vi "DL-SMART-MS-Modify-06-18-7.0.vi"() -> ()   [LabVIEW 2013]
uses:
  <vilib>/Utility/file.llb/Read From Spreadsheet File (DBL).vi
  <userlib>/caLab/Private/CaLabEvent_PV-1D.vi
  <userlib>/caLab/Private/Put_DBL-1D_PV.vi
  <userlib>/caLab/Private/Put_I32_PV.vi
  cal_p.vi
  <userlib>/caLab/Private/Get_PV.vi
  <vilib>/Utility/file.llb/Write To Spreadsheet File (DBL).vi
  <vilib>/vision/driver/NI_Vision_Acquisition_Software.lvlib
  <resource>/objmgr/imaqdx.rc
  <vilib>/Analysis/NI_AALPro.lvlib
panel:
  out "LaserEnergy uJ 2":dbl
  out "idn status":string
  out "MS":cluster{dbl[], "filtered data":dbl[]}(graph)
  out "std sample":T1(array[cluster])
  out "Image":T2(plugin-control)
  out "selected id":i32
  out "selected row":i32
  out "currentNO":string
  out "commet":string
  out "sampleID":string
  in  "Shots/Point":i32=100
  in  "chamber in":bool caption="TakeMS"
  in  "chamber out":bool caption="TakeMS"
  in  "Laser parameter":T4
  in  "ADC parameter":T5
  in  "ShutDownSystem":bool
  in  "ADC reference":refnum<vi>
  in  "SetLaserTransmission":dbl(slide) min=0.0 max=50.0 scale=0.0..20.0
  in  "LaserHV":u8=50 min=1 max=100
  in  "频率/Hz":u8=30
  out "Pul.HV-Real":dbl
  out "Identify Spcetrum":cluster{"ID1:X":dbl[], "ID1:Y":dbl[]}[](graph)
  in  "测试记录":i32(listbox)=6
  in  "Identification Results (单靶鉴定结果)":i32(listbox)=2
  in  "HVEnable":bool
  out "GateClose":bool
  out "LaserOK":bool
  out "HV-OK":bool
  out "Vacuum-OK":bool
  in  "Tab Control":T6(tab)
  in  "helix-Zeta-Step":dbl=100.0
  in  "helix-b":dbl=0.2
  in  "AcquireMS-Methods":u8(ring) items=["SinglePoint", "Multipoints", "MultiTar"]
  in  "Thresh":dbl=-0.005 format="%#_13g"
  in  "right rank":i32=2
  in  "left rank":i32=2
  in  "deBaseline":bool
  in  "MCPHV-Set":dbl=1400.0 min=0.0 max=1600.0
  in  "LensHV-Set":dbl=8000.0 min=0.0 max=10000.0
  in  "Tar.HV-Set":dbl=18010.0 min=0.0 max=20000.0
  in  "Pul.HV-Set":dbl=1400.0 min=0.0 max=2000.0
  in  "PulseDelay":dbl
  in  "ADCFreq":dbl
  in  "CH1_Coupling":u64(ring)=2 items=["Volt DC"=1, "Volt AC"=2, "Ampere DC"=4, "Ampere AC"=8, "Ohm"=16]
  in  "Channel 1_Range":dbl(ring)=4.0 items=["80 V"=80.0, "40 V"=40.0, "20 V"=20.0, "8 V"=8.0, "4 V"=4.0, "2 V"=2.0, "800 mV"=0.8, "400 mV"=0.4, "200 mV"=0.2]
  in  "Anal. Setting File":string="High Mass"
  in  "SettingFileSave":bool caption="TakeMS"
  in  "SettingFileAppl":bool caption="TakeMS"
  in  "SettingDel":bool caption="TakeMS"
  in  "RunADC":bool caption="TakeMS"
  out "ADCstatus":bool
  in  "Vac_Prot.":bool
  in  "Turbo_Fore":bool
  in  "Main_Samp":bool
  in  "Samp_Atmos":bool
  in  "Fore_Samp":bool
  in  "StartPump":bool
  in  "SopPump":bool
  out "TurboSpeed":dbl(knob) scale=0.0..100.0
  out "PumpKW":dbl
  out "PumpAmps":dbl
  out "PumpTemp":u16
  out "PumpVolts":dbl
  in  "laser OFF":bool
  in  "laser ON":bool
  out "cluster":T7
  in  "laser Deactive":bool
  out "A1-position-Y":dbl=45.0 caption="Y" min=0.0 max=55.0
  out "A1-position-X":dbl=53.4 caption="X" min=0.0 max=55.0
  in  "GO":bool
  in  "Y":dbl min=0.0 max=55.0
  in  "X":dbl min=0.0 max=55.0
  in  "A1-Position":bool caption="X-"
  in  "Plat_To_Zero":bool caption="TakeMS"
  in  "Plat_Cal":bool caption="TakeMS"
  out "Y当前":dbl
  out "X当前":dbl
  out "移动":bool
  out "Y满":bool
  out "Y标":bool
  out "X满":bool
  out "Y0":bool
  out "X0":bool
  out "靶位In/Out":bool
  out "仓门":bool
  out "Y过热":bool
  out "X过热":bool
  out "通讯":bool
  in  "Operation Record":i32(listbox)
  in  "OptionRecordLoad 2":bool caption="TakeMS"
  in  "OptionRecordClear":bool caption="TakeMS"
  out "c:":dbl
  out "b:":dbl
  out "a:":dbl
  in  "cancel cal":bool
  in  "cal save":bool
  in  "peak cal":bool
  in  "peak detect":bool
  in  "标准样品":u16(ring) items=["肺炎克雷伯菌", "铜绿假单胞菌"]
  in  "定标参数":i32(listbox)
  out "Tar.HV-Real":dbl
  out "LensHV-Real":dbl
  out "MCPHV-Real":dbl
  out "Lvaccum":dbl=0.83 format="%#_2e"
  out "Hvaccum":dbl=3.4e-05 format="%#_2e"
  in  "H12":bool
  in  "G12":bool
  in  "F12":bool
  in  "E12":bool
  in  "D12":bool
  in  "C12":bool
  in  "B12":bool
  in  "A12":bool
  in  "H11":bool
  in  "G11":bool
  in  "F11":bool
  in  "E11":bool
  in  "D11":bool
  in  "C11":bool
  in  "B11":bool
  in  "A11":bool
  in  "H10":bool
  in  "G10":bool
  in  "F10":bool
  in  "E10":bool
  in  "D10":bool
  in  "C10":bool
  in  "B10":bool
  in  "A10":bool
  in  "H9":bool
  in  "G9":bool
  in  "F9":bool
  in  "E9":bool
  in  "D9":bool
  in  "C9":bool
  in  "B9":bool
  in  "A9":bool
  in  "H8":bool
  in  "G8":bool
  in  "F8":bool
  in  "E8":bool
  in  "D8":bool
  in  "C8":bool
  in  "B8":bool
  in  "A8":bool
  in  "H7":bool
  in  "G7":bool
  in  "F7":bool
  in  "E7":bool
  in  "D7":bool
  in  "C7":bool
  in  "B7":bool
  in  "A7":bool
  in  "H6":bool
  in  "G6":bool
  in  "F6":bool
  in  "E6":bool
  in  "D6":bool
  in  "C6":bool
  in  "B6":bool
  in  "A6":bool
  in  "H5":bool
  in  "G5":bool
  in  "F5":bool
  in  "E5":bool
  in  "D5":bool
  in  "C5":bool
  in  "B5":bool
  in  "A5":bool
  in  "H4":bool
  in  "G4":bool
  in  "F4":bool
  in  "E4":bool
  in  "D4":bool
  in  "C4":bool
  in  "B4":bool
  in  "A4":bool
  in  "H3":bool
  in  "G3":bool
  in  "F3":bool
  in  "E3":bool
  in  "D3":bool
  in  "C3":bool
  in  "B3":bool
  in  "A3":bool
  in  "H2":bool
  in  "G2":bool
  in  "F2":bool
  in  "E2":bool
  in  "D2":bool
  in  "C2":bool
  in  "B2":bool
  in  "A2":bool
  in  "H1":bool
  in  "G1":bool
  in  "F1":bool
  in  "E1":bool
  in  "D1":bool
  in  "C1":bool
  in  "B1":bool
  in  "A1":bool
  in  "Clear":bool caption="TakeMS"
  in  "Add":bool caption="TakeMS"
  in  "TakeMS-Stop":bool caption="TakeMS"
  in  "TakeMS-Run":bool caption="TakeMS"
  # "Laser (激光)"
  # "光栅"
  # "uJ"
  # "Acq.(采谱)"
  # "Vacuum(真空)"
  # "1"
  # "2"
  # "3"
  # "4"
  # "5"
  # "6"
  # "7"
  # "8"
  # "9"
  # "10"
  # "11"
  # "12"
  # "A"
  # "Pa"
  # "High"
  # "B"
  # "Low"
  # "Pa"
  # "C"
  # "H.V.(高压)"
  # "D"
  # "MCP"
  # "V"
  # "E"
  # "Tar."
  # "V"
  # "F"
  # "Pul."
  # "V"
  # "G"
  # "Lens"
  # "V"
  # "H"
  # "Vauum (真空)"
  # "H.V. (高压)"
  # "Laser (激光)"
  # "Gate (仓门)"
  # "mm"
  # "Radian"
  # "H.V. (高压参数)"
  # "ADC(采集卡设置)"
  # "ADCFreq(采样)"
  # "MCP (探测器)"
  # "V"
  # "Hz"
  # "Tar. (靶)"
  # "V"
  # "Setting File(设置文件)"
  # "Coupling"
  # "Pulse (脉冲)"
  # "V"
  # "IntRange"
  # "V"
  # "Lens (透镜)"
  # "Delay (延时)"
  # "ns"
  # "Sole. Valves"
  # "Turbo Pump"
  # "自锁保护"
  # "机械/分子"
  # "主仓/样仓"
  # "样仓/大气"
  # "机械/样仓"
  # "激光器状态"
  # "mm"
  # "mm"
  # "mm"
  # "mm"
  # "mm"
  # "mm"
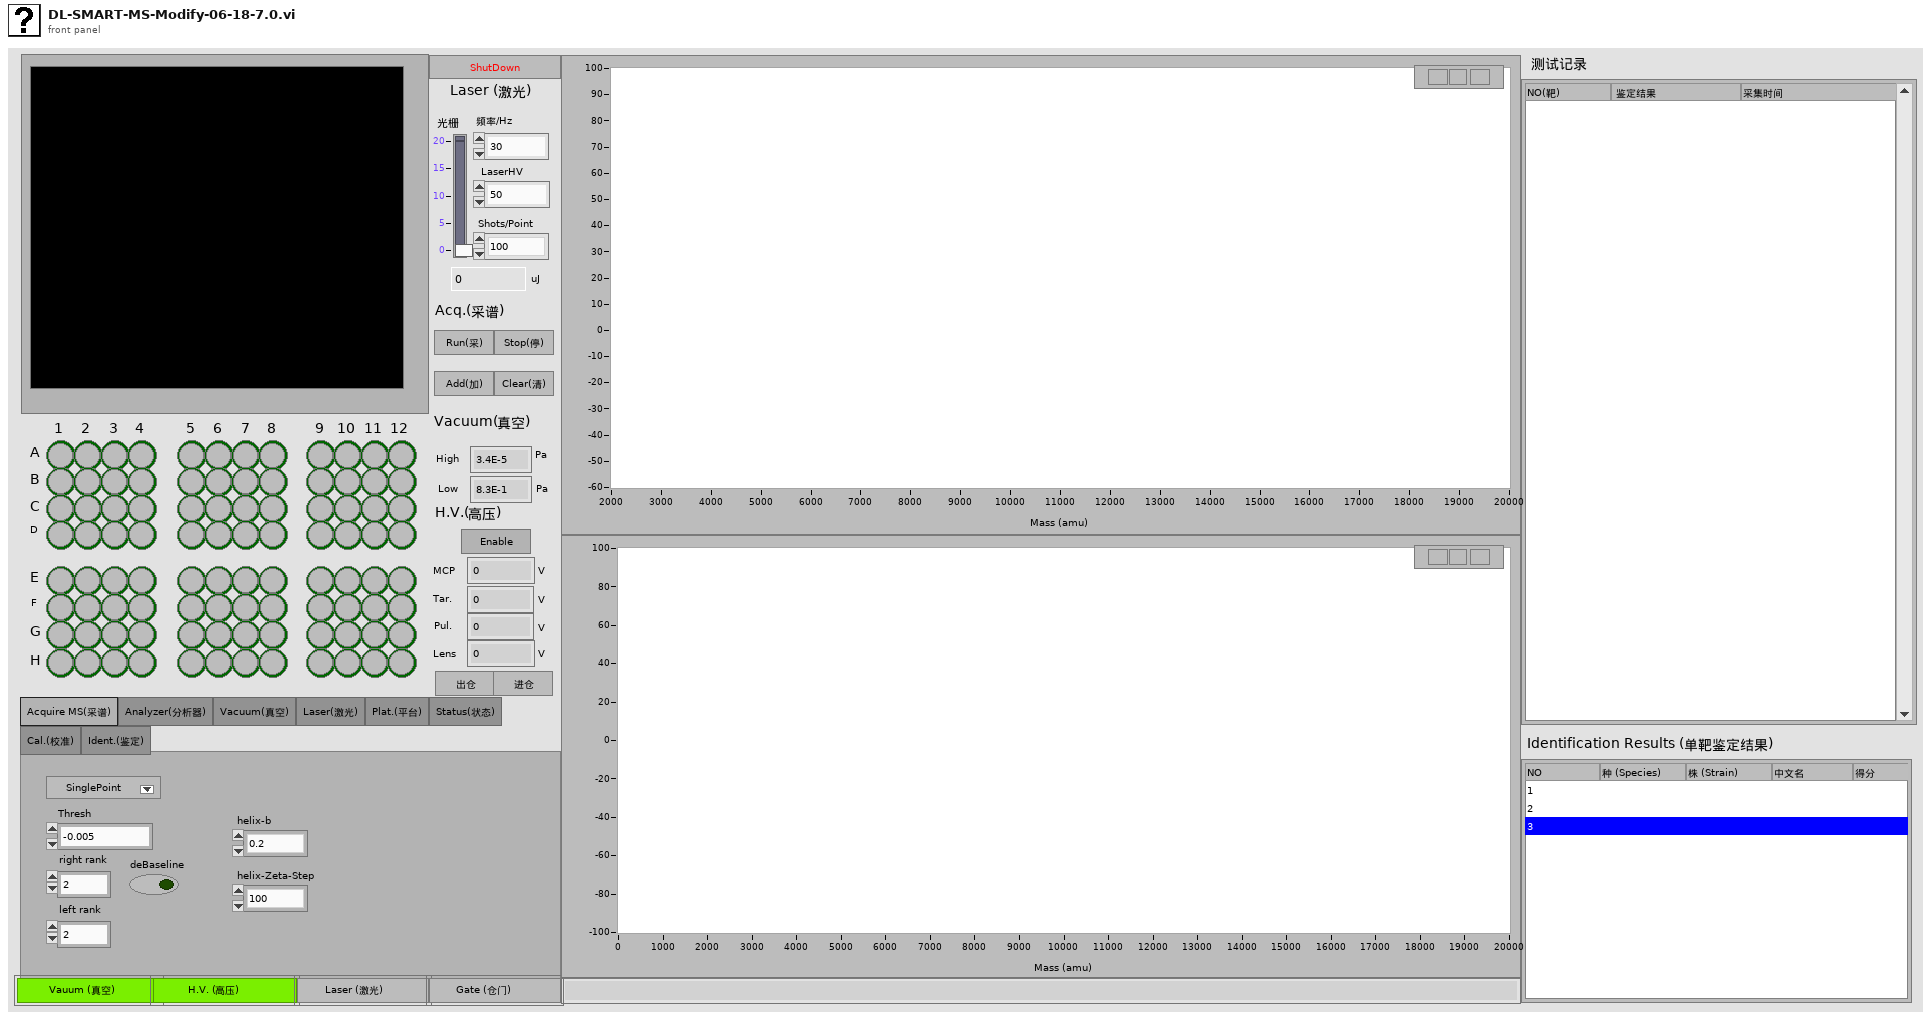
[diagram p1: front panel]
types:
  T1 = cluster{"name":string, "mz":dbl[], "time":dbl[]}[]
  T2 = typedef "IMAQ Image.ctl" = refnum<image>
  T3 = typedef "Semaphore RefNum" = refnum<k1>
  T4 = cluster{"VISA resource name":refnum<visa-resource-name>, "standby":bool, "semaphore in":T3, "SetLaserEnergy":dbl}
  T5 = cluster{"TpDeviceHandle_t":u32, "Record Length/Samples":u64, "ShotsPerPoint":u16}
  T6 = enum32{"Acquire MS(采谱)", "Analyzer(分析器)", "Vacuum(真空)", "Laser(激光)", "Plat.(平台)", "Status(状态)", "Cal.(校准)", "Ident.(鉴定)"}
  T7 = cluster{"链接":bool, "待机":bool, "发射":bool, "[3]":bool, "内存":bool, "测能":bool, "温警":bool, "静态":bool, "操作":bool}
  T8 = cluster{"tag1":string, "tag2":string, "x":dbl[], "y":dbl[], "ID1:X":dbl[], "ID1:Y":dbl[], "ID1:REF:X":dbl[], "ID1:REF:Y":dbl[], "ID2:X":dbl[], "ID2:Y":dbl[], "ID2:REF:X":dbl[], "ID2:REF:Y":dbl[], "ID3:X":dbl[], "ID3:Y":dbl[], "ID3:REF:X":dbl[], "ID3:REF:Y":dbl[], "ID1:TAG1":string, "ID1:TAG2":string, "ID2:TAG1":string, "ID2:TAG2":string, "ID3:TAG1":string, "ID3:TAG2":string, "ID1:NAME":string, "ID2:NAME":string, "ID3:NAME":string, "ID1:SCORE":string, "ID2:SCORE":string, "ID3:SCORE":string, "NO":string}[]
  T9 = cluster{"laser semaphore":T3, "pump semaphore":T3}
  T10 = enum8{"Enabled", "Disabled", "Disabled and Grayed Out"}
  T11 = cluster{"tag1":string, "tag2":string, "x":dbl[], "y":dbl[], "ID1:X":dbl[], "ID1:Y":dbl[], "ID1:REF:X":dbl[], "ID1:REF:Y":dbl[], "ID2:X":dbl[], "ID2:Y":dbl[], "ID2:REF:X":dbl[], "ID2:REF:Y":dbl[], "ID3:X":dbl[], "ID3:Y":dbl[], "ID3:REF:X":dbl[], "ID3:REF:Y":dbl[], "ID1:TAG1":string, "ID1:TAG2":string, "ID2:TAG1":string, "ID2:TAG2":string, "ID3:TAG1":string, "ID3:TAG2":string, "ID1:NAME":string, "ID2:NAME":string, "ID3:NAME":string, "ID1:SCORE":string, "ID2:SCORE":string, "ID3:SCORE":string, "NO":string}
  T12 = cluster{"monitor":refnum<user-event>, "motor status":refnum<user-event>, "motor":refnum<user-event>, "notifier out":refnum<notifier>, "queue out":refnum<queue>, "AI":T3, "DI":T3, "CX":T3, "CY":T3}
  T13 = cluster{"AI Task":refnum<k21>, "AO Task":refnum<k21>, "DO Task":refnum<k21>, "DI Task":refnum<k21>, "PWM x":refnum<k21>, "PWM y":refnum<k21>, "counter x":refnum<k21>, "counter y":refnum<k21>}
  T14 = cluster{"tasks":cluster{"AI Task":refnum<k21>, "AO Task":refnum<k21>, "DO Task":refnum<k21>, "DI Task":refnum<k21>, "PWM x":refnum<k21>, "PWM y":refnum<k21>, "counter x":refnum<k21>, "counter y":refnum<k21>}, "interface":cluster{"monitor":refnum<user-event>, "motor status":refnum<user-event>, "motor":refnum<user-event>, "notifier out":refnum<notifier>, "queue out":refnum<queue>, "AI":T3, "DI":T3, "CX":T3, "CY":T3}, "error out":errorcluster}
  T15 = cluster{"ConfiguredPumpCom":refnum<visa-resource-name>, "ConfiguredLaserCom":refnum<visa-resource-name>}
  T16 = typedef "LVPoint32TypeDef.ctl" = cluster{"Horizontal":i32, "Vertical":i32}
  T17 = typedef "LVRowAndColumnTypeDef.ctl" = cluster{"Row":i32, "Column":i32}
  T18 = cluster{"Type":u32, "Version":u32, "Flags":u32, "SerialNumberHigh":u32, "SerialNumberLow":u32, "BusType":u32, "InterfaceName":string, "VendorName":string, "ModelName":string, "CameraFileName":string, "CameraAttributeURL":string}[]
  T19 = cluster{"Type":u32, "Version":u32, "Flags":u32, "SerialNumberHigh":u32, "SerialNumberLow":u32, "BusType":u32, "InterfaceName":string, "VendorName":string, "ModelName":string, "CameraFileName":string, "CameraAttributeURL":string}
  T20 = typedef "IMAQdx.ctl" = refnum<k21>
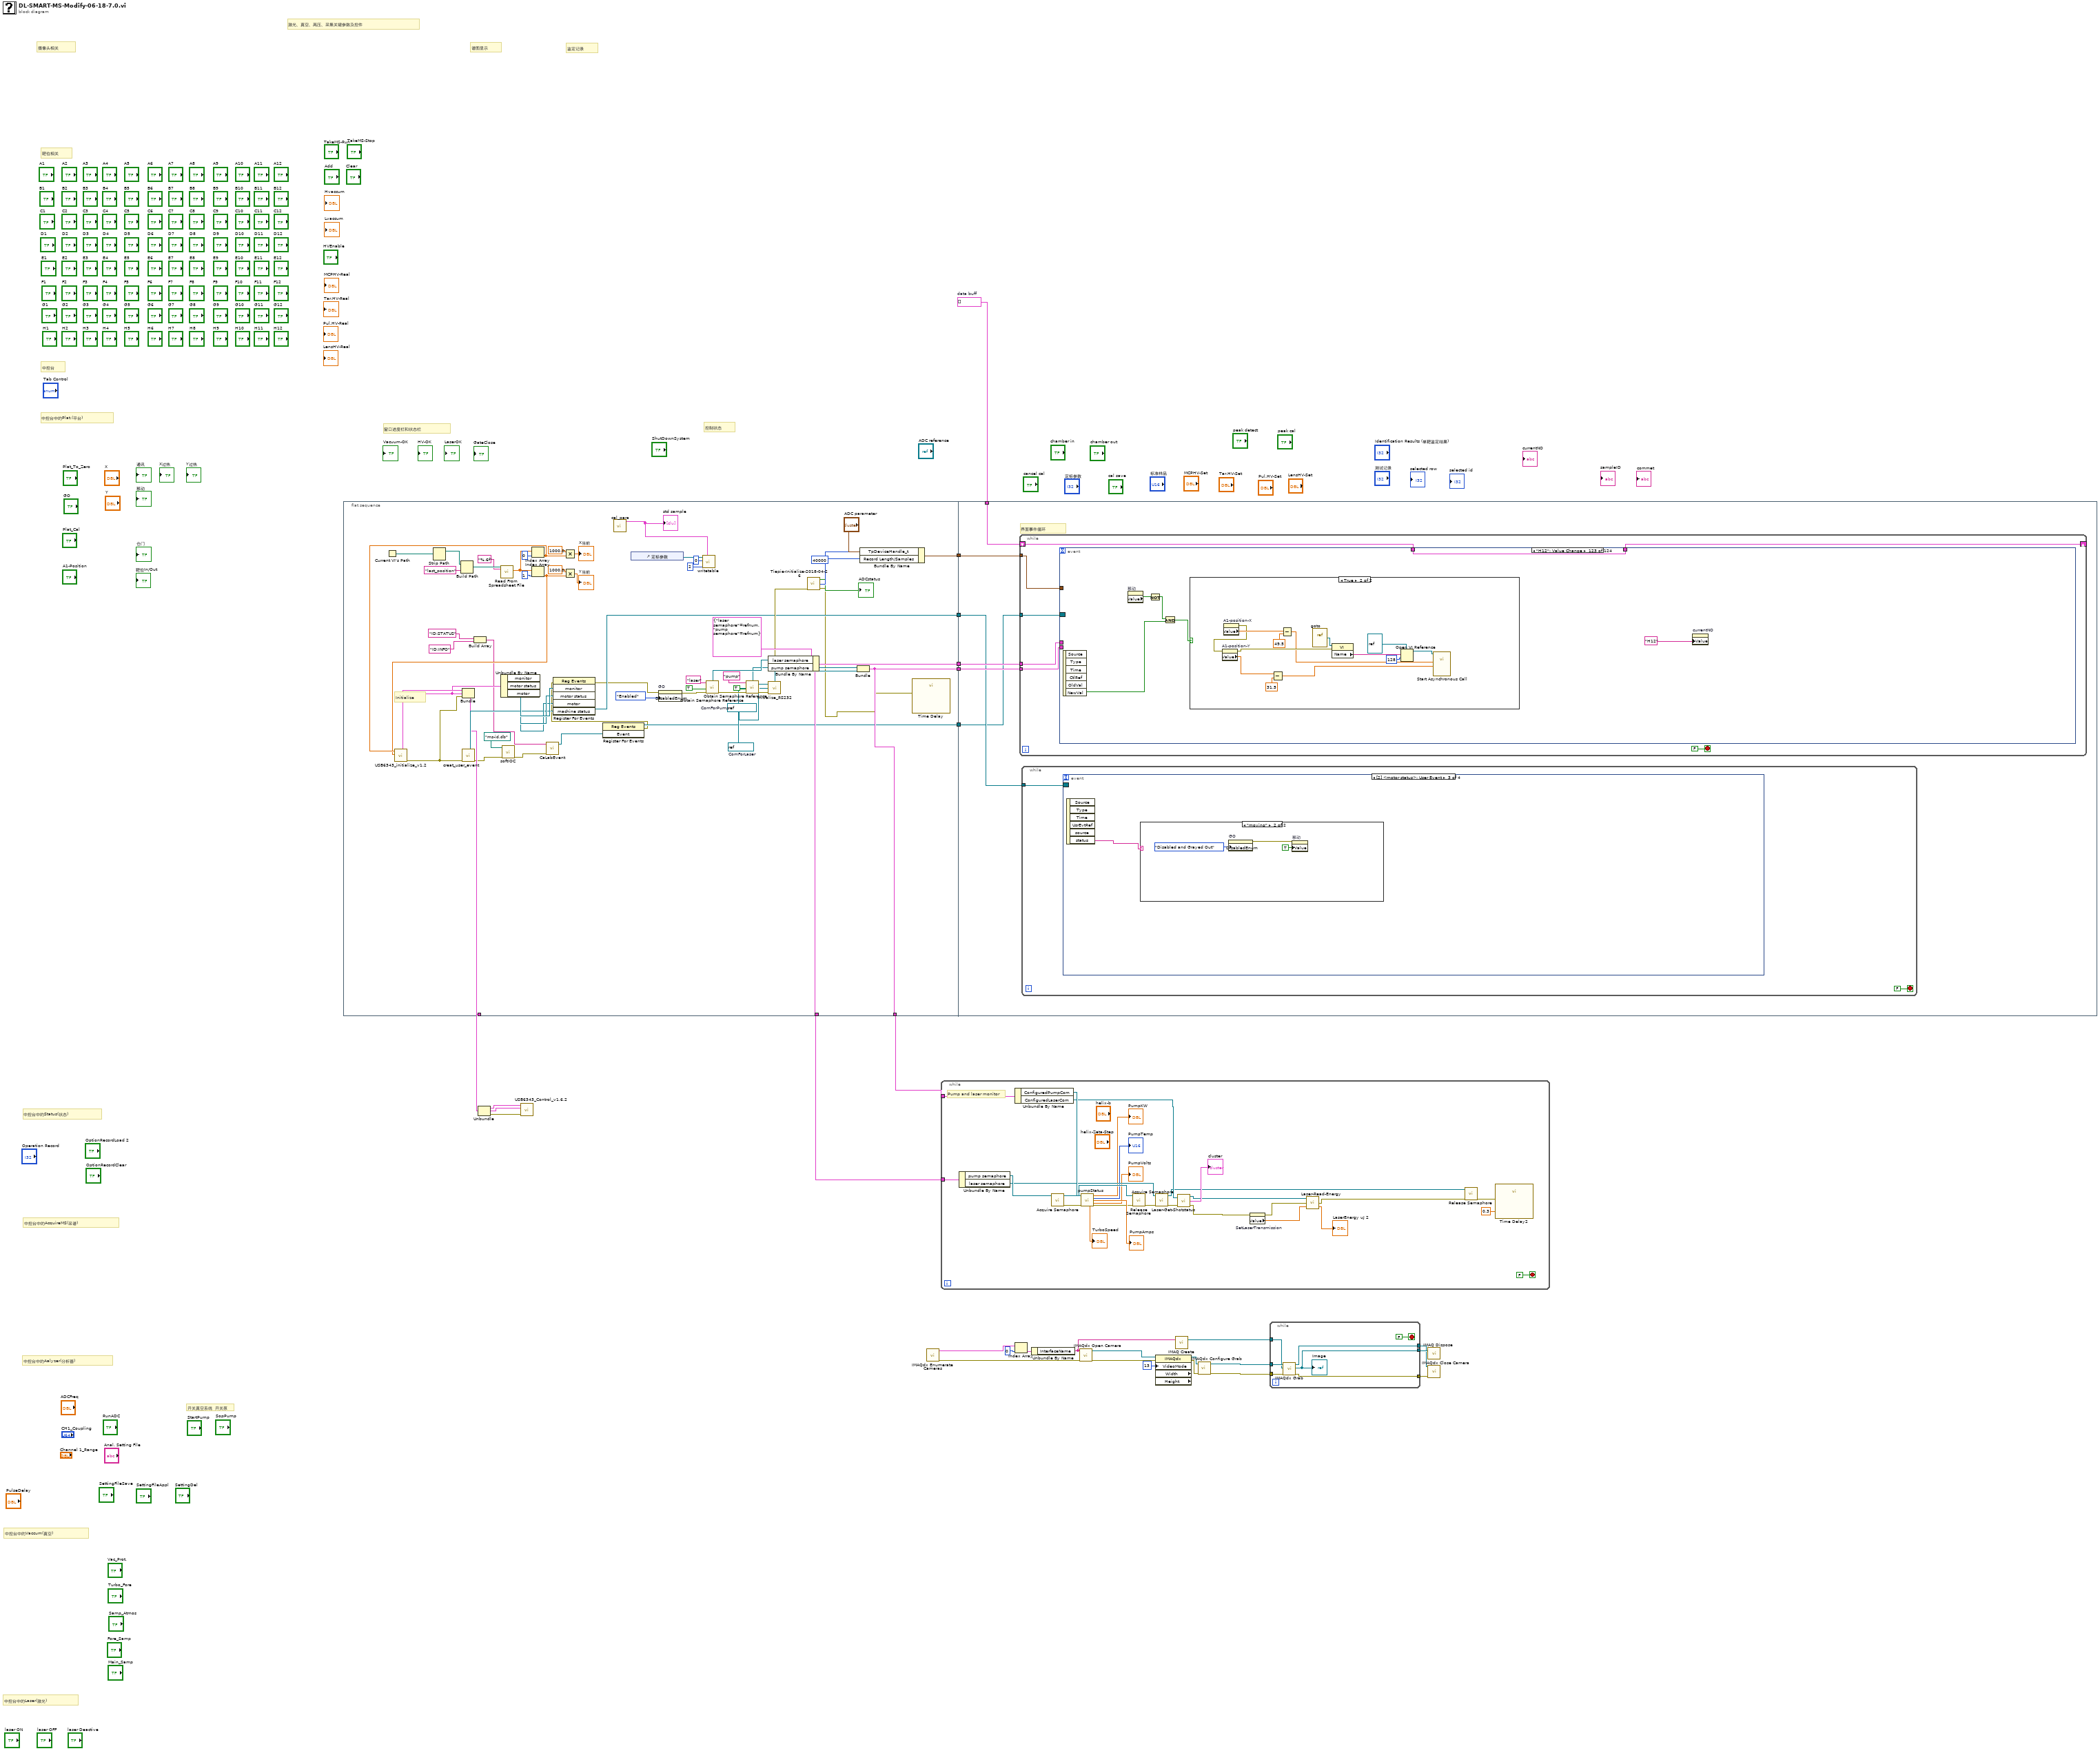
[diagram p0: block diagram]
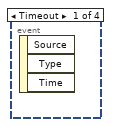
[diagram p2: hidden frame]
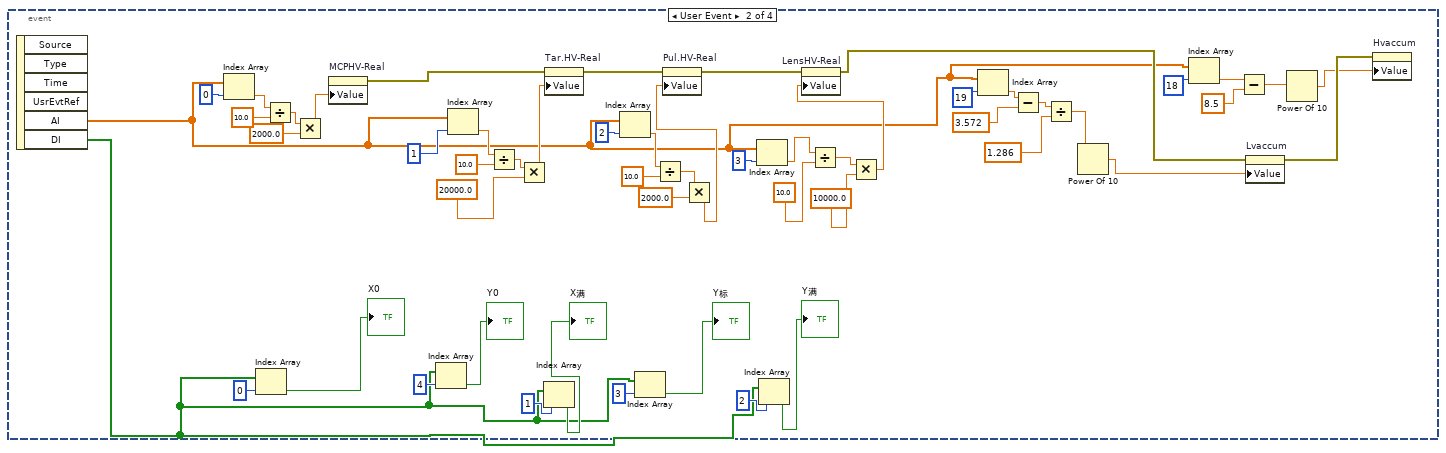
[diagram p3: hidden frame]
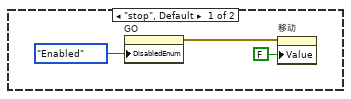
[diagram p4: hidden frame]
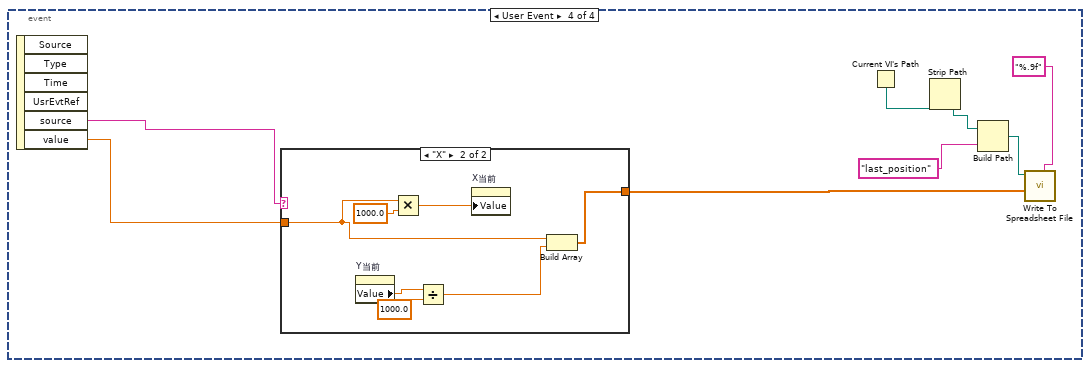
[diagram p5: hidden frame]
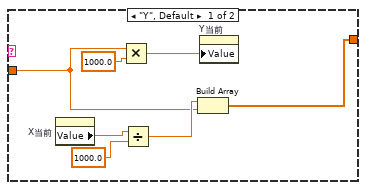
[diagram p6: hidden frame]
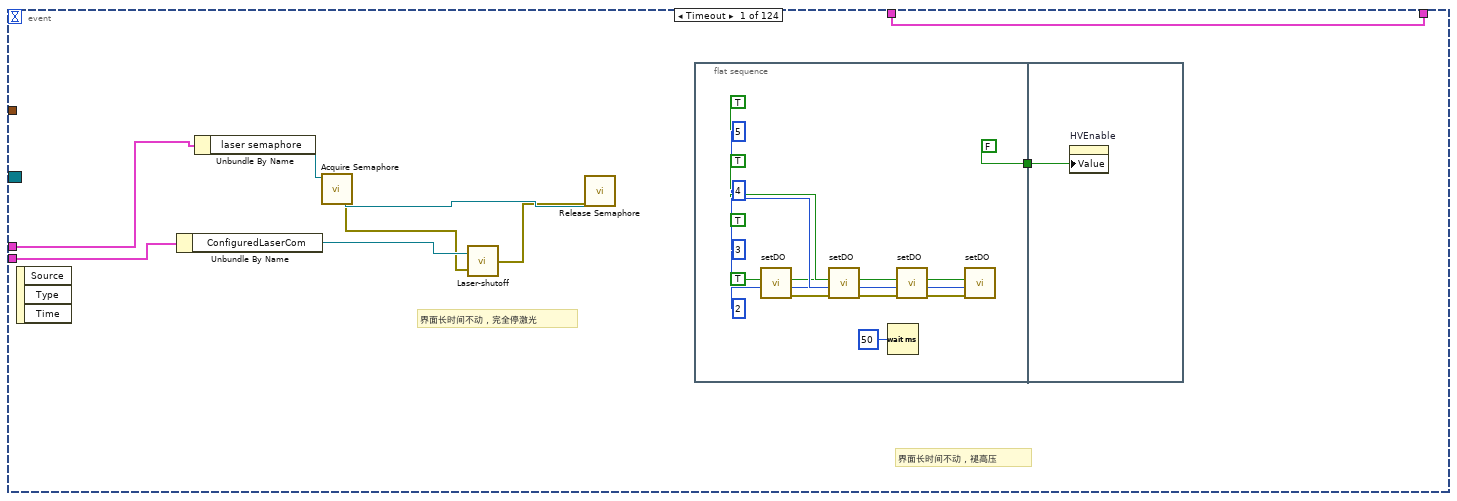
[diagram p7: hidden frame]
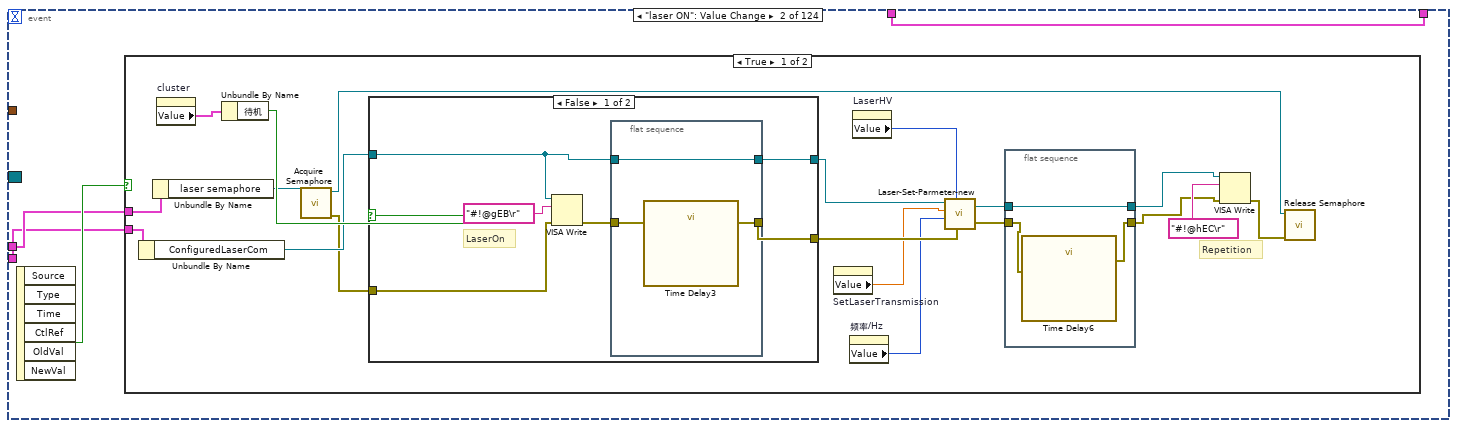
[diagram p8: hidden frame]
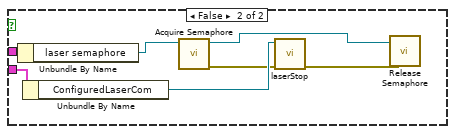
[diagram p10: hidden frame]
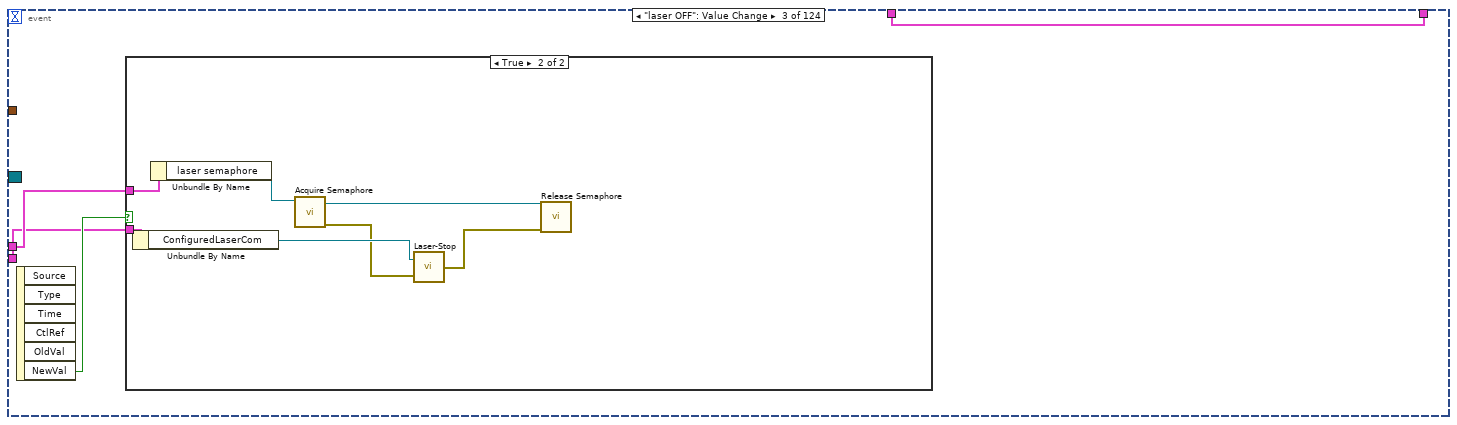
[diagram p11: hidden frame]
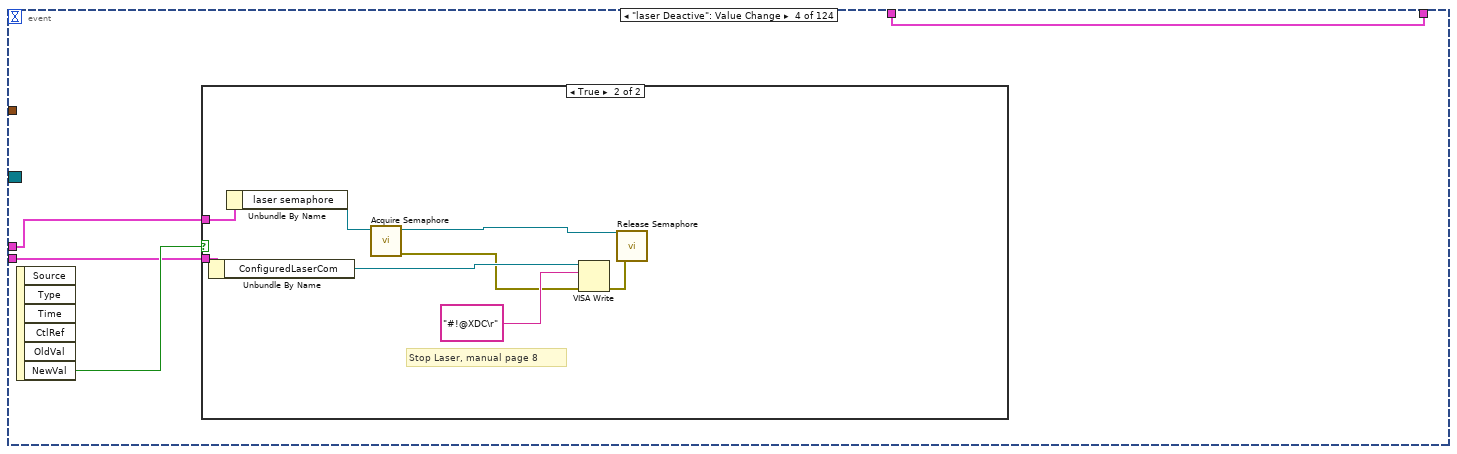
[diagram p13: hidden frame]
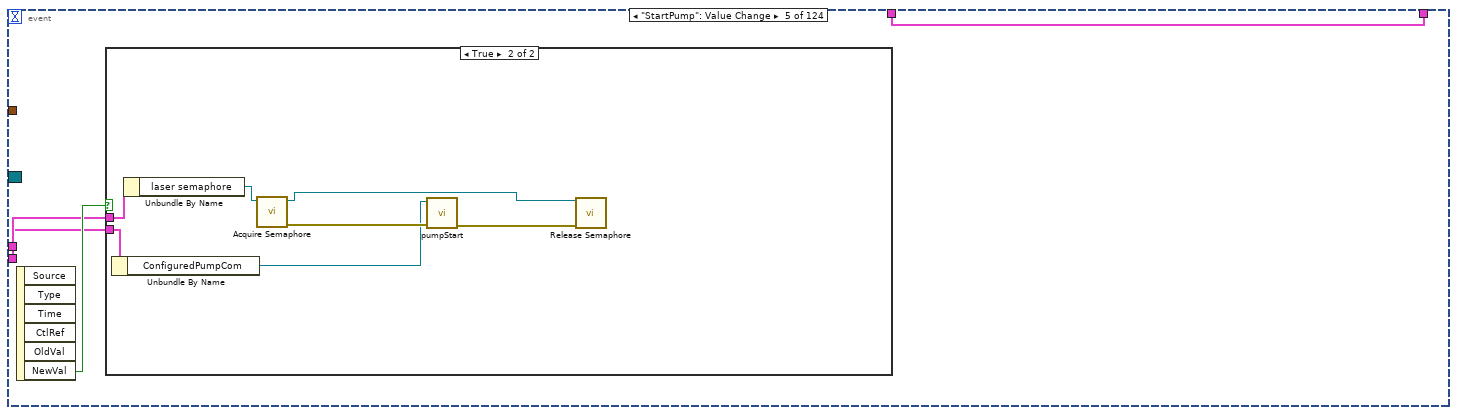
[diagram p15: hidden frame]
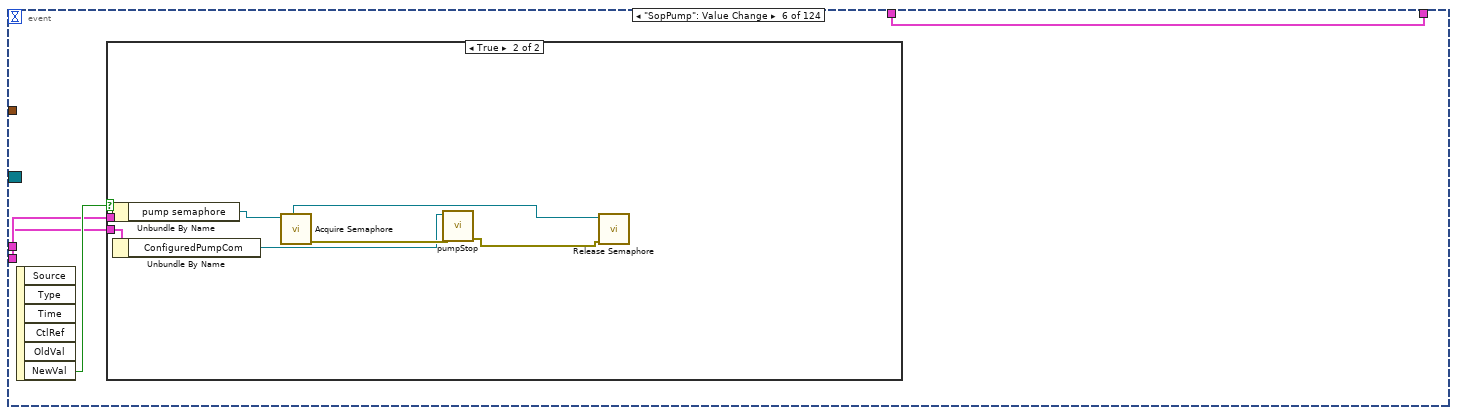
[diagram p17: hidden frame]
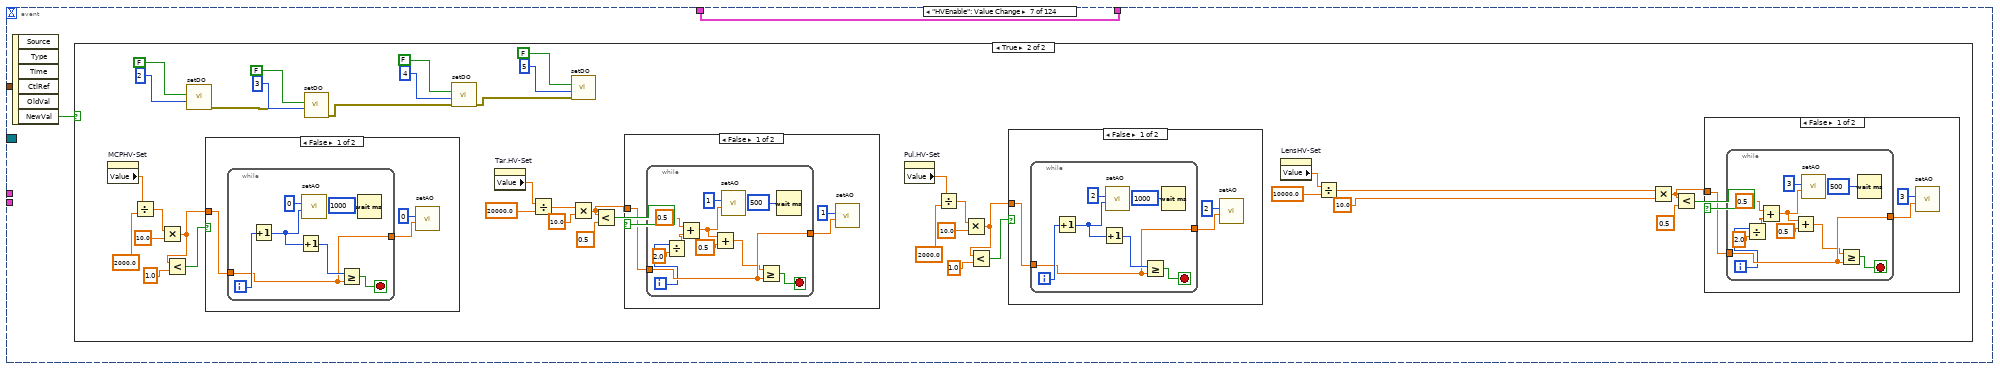
[diagram p19: hidden frame]
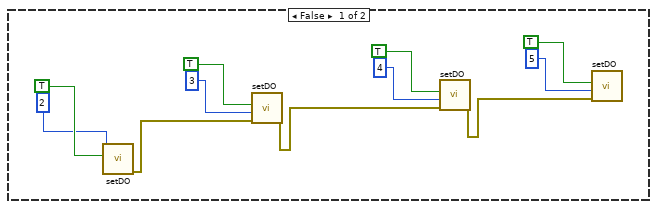
[diagram p20: hidden frame]
diagram:
  w21 = T8 []  # data buff
  # "Pump and laser monitor"
  # "开关真空系统  开关泵"
  # "控制状态"
  # "鉴定记录"
  # "谱图显示"
  # "激光、真空、高压、采集关键参数及控件"
  # "窗口进度栏和状态栏"
  # "中控台中的Laser(激光)"
  # "中控台中的Vaccum(真空)"
  # "中控台中的Aalyzer(分析器)"
  # "中控台中的AcquireMS(采谱)"
  # "中控台中的Status(状态)"
  # "中控台中的Plat.(平台)"
  # "中控台"
  # "靶位相关"
  # "摄像头相关"
  n1 = flat-sequence {
    tunnel: [w43] -> w28
    tunnel: [w68] -> w27
    tunnel: [w68] -> w25
    tunnel: [w67] -> w26
    tunnel: [w67] -> w24
    tunnel: [w71] -> w23
    tunnel: [w60] -> w22
    tunnel: [w30] -> w1
    tunnel: w28 -> [w91]
    tunnel: w27 -> [w95]
    tunnel: w26 -> [w94]
    tunnel: w22 -> [w93]
    tunnel: w21 -> [w92]
    tunnel: w1 -> [w90]
    frame #0 {
      w65 = refnum<visa-resource-name> "COM9"  # ComForLaser
      w66 = refnum<visa-resource-name> "COM10"  # ComForPump
      # "Initialize"
      n2 = Current VI's Path() -> (path=w58:path)
      n3 = Strip Path(path=w58) -> (stripped path=w57:path)  [unwired: 1 out]
      n4 = Build Path(base path=w57, name or relative path="last_position") -> (appended path=w55:path)
      n5 = Build Array("ID:STATUS", "ID:INFO") -> (w32:string[])
      n6 = call-poly <vilib>:"Read From Spreadsheet File.vi"("format (%.3f)"="%.6f", "file path (dialog if empty)"=w55) -> ("first row"=w53:dbl[])  [unwired: 5 in, 4 out]
      n7 = Index Array(array=w53, index=0) -> (element=w50:dbl)
      n8 = Index Array(array=w53, index=1) -> (element=w47:dbl)
      n9 = call "USB6343_initialize_v1.2.vi"("Y initial position"=w47, "X initial position"=w50) -> ("error out"=w72:errorcluster, "interface"=w73:T12, "tasks"=w74:T13)  [unwired: 7 in]
      n10 = Bundle("tasks"=w74, "interface"=w73, "error out"=w72) -> (w71:T14)  [unwired: 1 in]
      n11 = call "creat_user_event.vi"("error in (no error)"=w72) -> ("error out"=w40:errorcluster, "machine status"=w82:refnum<user-event>)  [unwired: 9 in]
      n12 = Unbundle By Name(w73) -> ("monitor"=w89:refnum<user-event>, "motor status"=w88:refnum<user-event>, "motor"=w87:refnum<user-event>)
      n13 = call "softIOC.vi"("error in (no error)"=w40, "路径"=path "ms-id.db") -> ("error out"=w41:errorcluster)  [unwired: 8 in, 1 out]
      n14 = call-poly <userlib>:"CaLabEvent.vi"("error in (no error)"=w41, "PV Names"=w32) -> ("Event"=w31:refnum<user-event>)  [unwired: 7 in, 2 out]
      n15 = Multiply(x=1000.0, y=w50) -> (x*y=→"X当前":dbl)
      n16 = Multiply(x=1000.0, y=w47) -> (x*y=→"Y当前":dbl)
      n17 = register-events(w31) -> (reference out=w30:refnum<event-registration>, error out=w29:errorcluster)  [unwired: 2 in]
      n18 = register-events(error in=w29, w89, w88, w87, w82) -> (reference out=w43:refnum<event-registration>, error out=w39:errorcluster)  [unwired: 1 in]
      n19 = call "cal_para.vi"() -> ("std sample"=w36:T1)  [unwired: 11 in]
      "std sample" <- w36
      n20 = control-ref of="定标参数"() -> (w38:refnum<vi>)
      n21 = property on="GO" class="Bool (strict)"(error in=w39, "DisabledEnum"=T10."Enabled" ("Disabled")) -> (error out=w83:errorcluster)  [unwired: 1 in, 1 out]
      n22 = call "writetable.vi"("std sample"=w36, "col"=2, "type"=0, "reference"=w38) -> ()  [unwired: 8 in]
      n23 = call <vilib>:"Obtain Semaphore Reference.vi"("error in (no error)"=w83, "create if not found (T)"=TRUE, "name (unnamed)"="laser") -> ("error out"=w78:errorcluster, "semaphore"=w75:T3)  [unwired: 2 in, 1 out]
      n24 = call <vilib>:"Obtain Semaphore Reference.vi"("error in (no error)"=w78, "create if not found (T)"=TRUE, "name (unnamed)"="pump") -> ("error out"=w77:errorcluster, "semaphore"=w69:T3)  [unwired: 2 in, 1 out]
      n25 = Bundle By Name(cluster=T9 {"laser semaphore"=refnum, "pump semaphore"=refnum}, "laser semaphore"=w75, "pump semaphore"=w69) -> (w68:T9)
      n26 = call "Initialize_RS232.vi"("error in (no error)"=w77, "ComForLaser"=w65, "ComForPump"=w66) -> ("error out"=w64:errorcluster, "ConfiguredLaserCom"=w80:refnum<visa-resource-name>, "ConfiguredPumpCom"=w81:refnum<visa-resource-name>)
      n27 = call "Tiepie-Initialize-2018-04-26.vi"("error in (no error)"=w64) -> ("error out"=w42:errorcluster, "TpDeviceHandle_t"=w62:u32, "Card-OK"=→"ADCstatus":bool)  [unwired: 3 in]
      n28 = Bundle("ConfiguredPumpCom"=w81, "ConfiguredLaserCom"=w80) -> (w67:T15)  [unwired: 1 in]
      n29 = Bundle By Name(cluster="ADC parameter", "TpDeviceHandle_t"=w62, "Record Length/Samples"=u64 40000) -> (w60:T5)
      n30 = call "Time Delay"("error in (no error)"=w42) -> ()  [unwired: 10 in, 1 out]
    }
    frame #1 {
      # "界面事件循环"
      n31 = while {
        tunnel: w90 -> [w186]
        tunnel: w94 -> [w185]
        tunnel: w95 -> [w184]
        tunnel: w93 -> [w182]
        shift-right: [w180] -> _
        shift-left: w92 -> [w181]
        stop <- FALSE stop-if-true
        n32 = event shown="[122] \"H12\": Value Change" {
          selector: w186 -> [_ _ _ _ _ _ _ _ _ _ _ _ _ _ _ _ _ _ _ _ _ _ _ _ _ _ _ _ _ _ _ _ _ _ _ _ _ _ _ _ _ _ _ _ _ _ _ _ _ _ _ _ _ _ _ _ _ _ _ _ _ _ _ _ _ _ _ _ _ _ _ _ _ _ _ _ _ _ _ _ _ _ _ _ _ _ _ _ _ _ _ _ _ _ _ _ _ _ _ _ _ _ _ _ _ _ _ _ _ _ _ _ _ _ _ _ _ _ _ _ _ _ _ _]
          dyn-events: _ -> [_ _ _ _ _ _ _ _ _ _ _ _ _ _ _ _ _ _ _ _ _ _ _ _ _ _ _ _ _ _ _ _ _ _ _ _ _ _ _ _ _ _ _ _ _ _ _ _ _ _ _ _ _ _ _ _ _ _ _ _ _ _ _ _ _ _ _ _ _ _ _ _ _ _ _ _ _ _ _ _ _ _ _ _ _ _ _ _ _ _ _ _ _ _ _ _ _ _ _ _ _ _ _ _ _ _ _ _ _ _ _ _ _ _ _ _ _ _ _ _ _ _ _ _]
          timeout: _ -> [_ _ _ _ _ _ _ _ _ _ _ _ _ _ _ _ _ _ _ _ _ _ _ _ _ _ _ _ _ _ _ _ _ _ _ _ _ _ _ _ _ _ _ _ _ _ _ _ _ _ _ _ _ _ _ _ _ _ _ _ _ _ _ _ _ _ _ _ _ _ _ _ _ _ _ _ _ _ _ _ _ _ _ _ _ _ _ _ _ _ _ _ _ _ _ _ _ _ _ _ _ _ _ _ _ _ _ _ _ _ _ _ _ _ _ _ _ _ _ _ _ _ _ _]
          tunnel: w185 -> [w189 w211 w254 w265 w277 w288 _ _ _ _ _ _ _ _ w483 w542 _ _ _ _ _ _ _ _ _ _ _ _ _ _ _ _ _ _ _ _ _ _ _ _ _ _ _ _ _ _ _ _ _ _ _ _ _ _ _ _ _ _ _ _ _ _ _ _ _ _ _ _ _ _ _ _ _ _ _ _ _ _ _ _ _ _ _ _ _ _ _ _ _ _ _ _ _ _ _ _ _ _ _ _ _ _ _ _ _ _ _ _ _ _ _ _ _ _ _ _ _ _ _ _ _ _ _ w2602]
          tunnel: w184 -> [w190 w212 w255 w264 w278 w289 _ _ _ _ _ _ _ _ w484 w543 _ _ _ _ _ _ _ _ _ _ _ _ _ _ _ _ _ _ _ _ _ _ _ _ _ _ _ _ _ _ _ _ _ _ _ _ _ _ _ _ _ _ _ _ _ _ _ _ _ _ _ _ _ _ _ _ _ _ _ _ _ _ _ _ _ _ _ _ _ _ _ _ _ _ _ _ _ _ _ _ _ _ _ _ _ _ _ _ _ _ _ _ _ _ _ _ _ _ _ _ _ _ _ _ _ _ _ _]
          tunnel: w182 -> [_ _ _ _ _ _ _ _ _ _ _ _ _ _ w485 _ _ _ _ _ _ _ _ _ _ _ _ _ _ _ _ _ _ _ _ _ _ _ _ _ _ _ _ _ _ _ _ _ _ _ _ _ _ _ _ _ _ _ _ _ _ _ _ _ _ _ _ _ _ _ _ _ _ _ _ _ _ _ _ _ _ _ _ _ _ _ _ _ _ _ _ _ _ _ _ _ _ _ _ _ _ _ _ _ _ _ _ _ _ _ _ _ _ _ _ _ _ _ _ _ _ _ _ _]
          tunnel: w181 -> [w187 w210 w253 w267 w276 w287 w298 w406 w421 w436 w443 w450 w457 w466 w482 w544 w546 w576 w611 w650 w652 w659 w694 w729 w731 w770 w775 w791 w809 w826 w843 w860 w877 w896 w921 w938 w955 w972 w989 w1006 w1025 w1044 w1063 w1082 w1101 w1120 w1139 w1158 w1177 w1196 w1215 w1234 w1253 w1272 w1291 w1310 w1329 w1348 w1367 w1386 w1405 w1424 w1443 w1462 w1481 w1500 w1519 w1538 w1557 w1576 w1599 w1618 w1637 w1656 w1675 w1694 w1713 w1732 w1751 w1770 w1789 w1808 w1827 w1846 w1865 w1884 w1903 w1922 w1941 w1960 w1979 w1998 w2017 w2036 w2055 w2074 w2093 w2112 w2131 w2150 w2169 w2188 w2207 w2226 w2245 w2264 w2283 w2302 w2321 w2340 w2359 w2378 w2397 w2416 w2435 w2454 w2473 w2492 w2511 w2530 w2549 w2568 w2587 w2601]
          tunnel: [w187 w210 w253 w267 w276 w287 w298 w406 w421 w436 w443 w450 w457 w466 w481 w544 w545 w576 w611 w650 w652 w659 w694 w729 w731 w770 w775 w791 w809 w826 w843 w860 w877 w895 w921 w938 w955 w972 w989 w1006 w1025 w1044 w1063 w1082 w1101 w1120 w1139 w1158 w1177 w1196 w1215 w1234 w1253 w1272 w1291 w1310 w1329 w1348 w1367 w1386 w1405 w1424 w1443 w1462 w1481 w1500 w1519 w1538 w1557 w1576 w1599 w1618 w1637 w1656 w1675 w1694 w1713 w1732 w1751 w1770 w1789 w1808 w1827 w1846 w1865 w1884 w1903 w1922 w1941 w1960 w1979 w1998 w2017 w2036 w2055 w2074 w2093 w2112 w2131 w2150 w2169 w2188 w2207 w2226 w2245 w2264 w2283 w2302 w2321 w2340 w2359 w2378 w2397 w2416 w2435 w2454 w2473 w2492 w2511 w2530 w2549 w2568 w2587 w2601] -> w180
          event Timeout {
            # "界面长时间不动，褪高压"
            # "界面长时间不动，完全停激光"
            n33 = event-data() -> ()  [unwired: 1 in, 3 out]
            n34 = Unbundle By Name(w189) -> ("ConfiguredLaserCom"=w193:refnum<visa-resource-name>)
            n35 = Unbundle By Name(w190) -> ("laser semaphore"=w195:T3)
            n36 = call <vilib>:"Acquire Semaphore.vi"("semaphore"=w195) -> ("error out"=w192:errorcluster, "semaphore out"=w194:T3)  [unwired: 4 in, 1 out]
            n37 = call "Laser-shutoff.vi"("error in (no error)"=w192, "VISA resource name"=w193) -> ("error out"=w191:errorcluster)
            n38 = call <vilib>:"Release Semaphore.vi"("error in (no error)"=w191, "semaphore"=w194) -> ()  [unwired: 4 in, 2 out]
            n39 = flat-sequence {
              tunnel: [FALSE ("HVEnable")] -> w188
              tunnel: w188 -> [w209]
              frame #0 {
                n40 = call "setDO.vi"("channel"=2, "on/off"=TRUE) -> ("错误输出"=w206:errorcluster)  [unwired: 9 in]
                n41 = call "setDO.vi"("错误输入（无错误）"=w206, "channel"=3, "on/off"=TRUE) -> ("错误输出"=w207:errorcluster)  [unwired: 8 in]
                n42 = Wait (ms)(milliseconds to wait=u32 50) -> ()  [unwired: 1 out]
                n43 = call "setDO.vi"("错误输入（无错误）"=w207, "channel"=4, "on/off"=TRUE) -> ("错误输出"=w208:errorcluster)  [unwired: 8 in]
                n44 = call "setDO.vi"("错误输入（无错误）"=w208, "channel"=5, "on/off"=TRUE) -> ()  [unwired: 8 in, 1 out]
              }
              frame #1 {
                n45 = property on="HVEnable" class="Bool (strict)"("Value"=w209) -> ()  [unwired: 2 in, 2 out]
              }
            }
          }
          event "laser ON": Value Change {
            n46 = event-data() -> ("NewVal"=w213:bool)  [unwired: 1 in, 5 out]
            n47 = case shown="True" w213 {
              tunnel: w212 -> [w232 w252]
              tunnel: w211 -> [w231 w250]
              frame True {
                # "Repetition"
                n48 = Unbundle By Name(w231) -> ("ConfiguredLaserCom"=w228:refnum<visa-resource-name>)
                n49 = Unbundle By Name(w232) -> ("laser semaphore"=w225:T3)
                n50 = property on="cluster" class="Clust (strict)"() -> ("Value"=w230:T7)  [unwired: 2 in, 2 out]
                n51 = Unbundle By Name(w230) -> ("待机"=w229:bool)
                n52 = call <vilib>:"Acquire Semaphore.vi"("semaphore"=w225) -> ("error out"=w223:errorcluster, "semaphore out"=w224:T3)  [unwired: 4 in, 1 out]
                n53 = case shown="False" w229 {
                  tunnel: w228 -> [w240 w245]
                  tunnel: [w239 w245] -> w222
                  tunnel: [w237 w244] -> w221
                  tunnel: w223 -> [w236 w244]
                  frame False {
                    # "LaserOn"
                    n54 = VISA Write(VISA resource name=w240, write buffer="#!@gEB\r", error in (no error)=w236) -> (error out=w238:errorcluster)  [unwired: 2 out]
                    n55 = flat-sequence {
                      tunnel: w238 -> [w243]
                      tunnel: [w243] -> w237
                      tunnel: w240 -> [w242]
                      tunnel: [w242] -> w239
                      frame #0 {
                        n56 = call "Time Delay3"() -> ()  [unwired: 11 in, 1 out]
                      }
                    }
                  }
                  frame True {
                  }
                }
                n57 = property on="SetLaserTransmission" class="Slide (strict)"() -> ("Value"=w215:dbl)  [unwired: 2 in, 2 out]
                n58 = property on="频率/Hz" class="DigNum (strict)"() -> ("Value"=w214:u8)  [unwired: 2 in, 2 out]
                n59 = property on="LaserHV" class="DigNum (strict)"() -> ("Value"=w216:u8)  [unwired: 2 in, 2 out]
                n60 = call "Laser-Set-Parmeter-new.vi"("error in (no error)"=w221, "LaserHV"=w216, "LaserFreq"=w214, "SetTransmission"=w215, "VISA resource name"=w222) -> ("error out"=w218:errorcluster, "VISA resource name out"=w220:refnum<visa-resource-name>)  [unwired: 1 in]
                n61 = flat-sequence {
                  tunnel: w220 -> [w235]
                  tunnel: [w235] -> w219
                  tunnel: w218 -> [w234]
                  tunnel: [w233] -> w217
                  frame #0 {
                    n62 = call "Time Delay6"("error in (no error)"=w234) -> ("error out"=w233:errorcluster)  [unwired: 10 in]
                  }
                }
                n63 = VISA Write(VISA resource name=w219, write buffer="#!@hEC\r", error in (no error)=w217) -> (error out=w226:errorcluster)  [unwired: 2 out]
                n64 = call <vilib>:"Release Semaphore.vi"("error in (no error)"=w226, "semaphore"=w224) -> ()  [unwired: 4 in, 2 out]
              }
              frame False {
                n65 = Unbundle By Name(w252) -> ("laser semaphore"=w251:T3)
                n66 = Unbundle By Name(w250) -> ("ConfiguredLaserCom"=w249:refnum<visa-resource-name>)
                n67 = call <vilib>:"Acquire Semaphore.vi"("semaphore"=w251) -> ("error out"=w248:errorcluster, "semaphore out"=w246:T3)  [unwired: 4 in, 1 out]
                n68 = call "laserStop.vi"("error in (no error)"=w248, "VISA resource name"=w249) -> ("error out"=w247:errorcluster)  [unwired: 9 in]
                n69 = call <vilib>:"Release Semaphore.vi"("error in (no error)"=w247, "semaphore"=w246) -> ()  [unwired: 4 in, 2 out]
              }
            }
          }
          event "laser OFF": Value Change {
            n70 = event-data() -> ("NewVal"=w256:bool)  [unwired: 1 in, 5 out]
            n71 = case shown="True" w256 {
              tunnel: w255 -> [_ w263]
              tunnel: w254 -> [_ w261]
              frame False {
              }
              frame True {
                n72 = Unbundle By Name(w261) -> ("ConfiguredLaserCom"=w259:refnum<visa-resource-name>)
                n73 = Unbundle By Name(w263) -> ("laser semaphore"=w262:T3)
                n74 = call <vilib>:"Acquire Semaphore.vi"("semaphore"=w262) -> ("error out"=w258:errorcluster, "semaphore out"=w260:T3)  [unwired: 4 in, 1 out]
                n75 = call "Laser-Stop.vi"("error in (no error)"=w258, "VISA resource name"=w259) -> ("error out"=w257:errorcluster)
                n76 = call <vilib>:"Release Semaphore.vi"("error in (no error)"=w257, "semaphore"=w260) -> ()  [unwired: 4 in, 2 out]
              }
            }
          }
          event "laser Deactive": Value Change {
            n77 = event-data() -> ("NewVal"=w266:bool)  [unwired: 1 in, 5 out]
            n78 = case shown="True" w266 {
              tunnel: w264 -> [_ w275]
              tunnel: w265 -> [_ w273]
              frame False {
              }
              frame True {
                # "Stop Laser, manual page 8"
                n79 = Unbundle By Name(w273) -> ("ConfiguredLaserCom"=w270:refnum<visa-resource-name>)
                n80 = Unbundle By Name(w275) -> ("laser semaphore"=w274:T3)
                n81 = call <vilib>:"Acquire Semaphore.vi"("semaphore"=w274) -> ("error out"=w269:errorcluster, "semaphore out"=w272:T3)  [unwired: 4 in, 1 out]
                n82 = VISA Write(VISA resource name=w270, write buffer="#!@XDC\r", error in (no error)=w269) -> (error out=w268:errorcluster)  [unwired: 2 out]
                n83 = call <vilib>:"Release Semaphore.vi"("error in (no error)"=w268, "semaphore"=w272) -> ()  [unwired: 4 in, 2 out]
              }
            }
          }
          event "StartPump": Value Change {
            n84 = event-data() -> ("NewVal"=w279:bool)  [unwired: 1 in, 5 out]
            n85 = case shown="True" w279 {
              tunnel: w278 -> [_ w284]
              tunnel: w277 -> [_ w283]
              frame False {
              }
              frame True {
                n86 = Unbundle By Name(w283) -> ("ConfiguredPumpCom"=w282:refnum<visa-resource-name>)
                n87 = Unbundle By Name(w284) -> ("laser semaphore"=w281:T3)
                n88 = call <vilib>:"Acquire Semaphore.vi"("semaphore"=w281) -> ("error out"=w286:errorcluster, "semaphore out"=w280:T3)  [unwired: 4 in, 1 out]
                n89 = call "pumpStart.vi"("error in (no error)"=w286, "VISA resource name"=w282) -> ("error out"=w285:errorcluster)  [unwired: 9 in]
                n90 = call <vilib>:"Release Semaphore.vi"("error in (no error)"=w285, "semaphore"=w280) -> ()  [unwired: 4 in, 2 out]
              }
            }
          }
          event "SopPump": Value Change {
            n91 = event-data() -> ("NewVal"=w290:bool)  [unwired: 1 in, 5 out]
            n92 = case shown="True" w290 {
              tunnel: w289 -> [_ w294]
              tunnel: w288 -> [_ w292]
              frame False {
              }
              frame True {
                n93 = Unbundle By Name(w294) -> ("pump semaphore"=w293:T3)
                n94 = Unbundle By Name(w292) -> ("ConfiguredPumpCom"=w291:refnum<visa-resource-name>)
                n95 = call <vilib>:"Acquire Semaphore.vi"("semaphore"=w293) -> ("error out"=w297:errorcluster, "semaphore out"=w295:T3)  [unwired: 4 in, 1 out]
                n96 = call "pumpStop.vi"("error in (no error)"=w297, "VISA resource name"=w291) -> ("error out"=w296:errorcluster)  [unwired: 9 in]
                n97 = call <vilib>:"Release Semaphore.vi"("error in (no error)"=w296, "semaphore"=w295) -> ()  [unwired: 4 in, 2 out]
              }
            }
          }
          event "HVEnable": Value Change {
            n98 = event-data() -> ("NewVal"=w299:bool)  [unwired: 1 in, 5 out]
            n99 = case shown="True" w299 {
              frame False {
                n100 = call "setDO.vi"("channel"=2, "on/off"=TRUE) -> ("错误输出"=w302:errorcluster)  [unwired: 9 in]
                n101 = call "setDO.vi"("错误输入（无错误）"=w302, "channel"=3, "on/off"=TRUE) -> ("错误输出"=w301:errorcluster)  [unwired: 8 in]
                n102 = call "setDO.vi"("错误输入（无错误）"=w301, "channel"=4, "on/off"=TRUE) -> ("错误输出"=w300:errorcluster)  [unwired: 8 in]
                n103 = call "setDO.vi"("错误输入（无错误）"=w300, "channel"=5, "on/off"=TRUE) -> ()  [unwired: 8 in, 1 out]
              }
              frame True {
                n104 = property on="MCPHV-Set" class="DigNum (strict)"() -> ("Value"=w335:dbl)  [unwired: 2 in, 2 out]
                n105 = Divide(x=w335, y=2000.0) -> (x/y=w337:dbl)
                n106 = Multiply(x=w337, y=10.0) -> (x*y=w328:dbl)
                n107 = Less?(x=w328, y=1.0) -> (x < y?=w329:bool)
                n108 = call "setDO.vi"("channel"=2, "on/off"=FALSE) -> ("错误输出"=w341:errorcluster)  [unwired: 9 in]
                n109 = case shown="False" w329 {
                  tunnel: w328 -> [w396 w404]
                  frame False {
                    n110 = while {
                      tunnel: w396 -> [w398]
                      tunnel: [w398] -> w394
                      i -> [w402]
                      stop <- w399 stop-if-true
                      n111 = Increment(x=w402) -> (x+1=w401:i32)
                      n112 = Increment(x=w401) -> (x+1=w400:i32)
                      n113 = call "setAO.vi"("value"=w401, "channel"=0) -> ()  [unwired: 9 in, 1 out]
                      n114 = Greater Or Equal?(x=w400, y=w398) -> (x >= y?=w399:bool)
                      n115 = Wait (ms)(milliseconds to wait=1000) -> ()  [unwired: 1 out]
                    }
                    n116 = call "setAO.vi"("value"=w394, "channel"=0) -> ()  [unwired: 9 in, 1 out]
                  }
                  frame True {
                    n117 = call "setAO.vi"("value"=w404, "channel"=0) -> ()  [unwired: 9 in, 1 out]
                  }
                }
                n118 = call "setDO.vi"("错误输入（无错误）"=w341, "channel"=3, "on/off"=FALSE) -> ("错误输出"=w340:errorcluster)  [unwired: 8 in]
                n119 = call "setDO.vi"("错误输入（无错误）"=w340, "channel"=4, "on/off"=FALSE) -> ("错误输出"=w339:errorcluster)  [unwired: 8 in]
                n120 = property on="Tar.HV-Set" class="DigNum (strict)"() -> ("Value"=w331:dbl)  [unwired: 2 in, 2 out]
                n121 = Divide(x=w331, y=20000.0) -> (x/y=w333:dbl)
                n122 = call "setDO.vi"("错误输入（无错误）"=w339, "channel"=5, "on/off"=FALSE) -> ()  [unwired: 8 in, 1 out]
                n123 = Multiply(x=w333, y=10.0) -> (x*y=w325:dbl)
                n124 = Less?(x=w325, y=0.5) -> (x < y?=w326:bool)
                n125 = case shown="False" w326 {
                  tunnel: w325 -> [w380 w392]
                  frame False {
                    n126 = while {
                      tunnel: w380 -> [w389]
                      tunnel: [w389] -> w378
                      i -> [w385]
                      stop <- w390 stop-if-true
                      n127 = Divide(x=w385, y=2.0) -> (x/y=w386:dbl)
                      n128 = Add(x=0.5, y=w386) -> (x+y=w383:dbl)
                      n129 = Add(x=w383, y=0.5) -> (x+y=w381:dbl)
                      n130 = call "setAO.vi"("value"=w383, "channel"=1) -> ()  [unwired: 9 in, 1 out]
                      n131 = Greater Or Equal?(x=w381, y=w389) -> (x >= y?=w390:bool)
                      n132 = Wait (ms)(milliseconds to wait=500) -> ()  [unwired: 1 out]
                    }
                    n133 = call "setAO.vi"("value"=w378, "channel"=1) -> ()  [unwired: 9 in, 1 out]
                  }
                  frame True {
                    n134 = call "setAO.vi"("value"=w392, "channel"=1) -> ()  [unwired: 9 in, 1 out]
                  }
                }
                n135 = property on="Pul.HV-Set" class="DigNum (strict)"() -> ("Value"=w324:dbl)  [unwired: 2 in, 2 out]
                n136 = Divide(x=w324, y=2000.0) -> (x/y=w319:dbl)
                n137 = Multiply(x=w319, y=10.0) -> (x*y=w323:dbl)
                n138 = Less?(x=w323, y=1.0) -> (x < y?=w322:bool)
                n139 = case shown="False" w322 {
                  tunnel: w323 -> [w368 w376]
                  frame False {
                    n140 = while {
                      tunnel: w368 -> [w370]
                      tunnel: [w370] -> w366
                      i -> [w374]
                      stop <- w371 stop-if-true
                      n141 = Increment(x=w374) -> (x+1=w373:i32)
                      n142 = Increment(x=w373) -> (x+1=w372:i32)
                      n143 = call "setAO.vi"("value"=w373, "channel"=2) -> ()  [unwired: 9 in, 1 out]
                      n144 = Greater Or Equal?(x=w372, y=w370) -> (x >= y?=w371:bool)
                      n145 = Wait (ms)(milliseconds to wait=1000) -> ()  [unwired: 1 out]
                    }
                    n146 = call "setAO.vi"("value"=w366, "channel"=2) -> ()  [unwired: 9 in, 1 out]
                  }
                  frame True {
                    n147 = call "setAO.vi"("value"=w376, "channel"=2) -> ()  [unwired: 9 in, 1 out]
                  }
                }
                n148 = property on="LensHV-Set" class="DigNum (strict)"() -> ("Value"=w317:dbl)  [unwired: 2 in, 2 out]
                n149 = Divide(x=w317, y=10000.0) -> (x/y=w312:dbl)
                n150 = Multiply(x=w312, y=10.0) -> (x*y=w316:dbl)
                n151 = Less?(x=w316, y=0.5) -> (x < y?=w315:bool)
                n152 = case shown="False" w315 {
                  tunnel: w316 -> [w352 w364]
                  frame False {
                    n153 = while {
                      tunnel: w352 -> [w361]
                      tunnel: [w361] -> w350
                      i -> [w357]
                      stop <- w362 stop-if-true
                      n154 = Divide(x=w357, y=2.0) -> (x/y=w358:dbl)
                      n155 = Add(x=0.5, y=w358) -> (x+y=w355:dbl)
                      n156 = Add(x=w355, y=0.5) -> (x+y=w353:dbl)
                      n157 = call "setAO.vi"("value"=w355, "channel"=3) -> ()  [unwired: 9 in, 1 out]
                      n158 = Greater Or Equal?(x=w353, y=w361) -> (x >= y?=w362:bool)
                      n159 = Wait (ms)(milliseconds to wait=500) -> ()  [unwired: 1 out]
                    }
                    n160 = call "setAO.vi"("value"=w350, "channel"=3) -> ()  [unwired: 9 in, 1 out]
                  }
                  frame True {
                    n161 = call "setAO.vi"("value"=w364, "channel"=3) -> ()  [unwired: 9 in, 1 out]
                  }
                }
              }
            }
          }
          event "Samp_Atmos": Value Change {
            n162 = event-data() -> ("OldVal"=w407:bool, "NewVal"=w411:bool)  [unwired: 1 in, 4 out]
            n163 = property on="Fore_Samp" class="Bool (strict)"() -> ("Value"=w410:bool)  [unwired: 2 in, 2 out]
            n164 = And(x=w411, y=w410) -> (x .and. y?=w409:bool)
            n165 = Not(x=w409) -> (.not. x?=w408:bool)
            n166 = case shown="True" w408 {
              tunnel: w411 -> [_ w414]
              tunnel: w407 -> [w413 _]
              frame False {
                n167 = property on="Samp_Atmos" class="Bool (strict)"("Value"=w413) -> (error out=w412:errorcluster)  [unwired: 2 in, 1 out]
                n168 = call "Display Message to User7"("error in (no error)"=w412) -> ()  [unwired: 9 in, 2 out]
              }
              frame True {
                n169 = case shown="False" w414 {
                  frame False {
                    n170 = call "setDO.vi"("channel"=6, "on/off"=FALSE) -> ()  [unwired: 9 in, 1 out]
                  }
                  frame True {
                    n171 = property on="Y满" class="Bool (strict)"() -> ("Value"=w418:bool)  [unwired: 2 in, 2 out]
                    n172 = Not(x=w418) -> (.not. x?=w417:bool)
                    n173 = case shown="False" w417 {
                      frame False {
                        n174 = call "setDO.vi"("channel"=6, "on/off"=TRUE) -> ()  [unwired: 9 in, 1 out]
                      }
                      frame True {
                        n175 = call "Display Message to User6"() -> ()  [unwired: 10 in, 2 out]
                      }
                    }
                  }
                }
              }
            }
          }
          event "Fore_Samp": Value Change {
            n176 = event-data() -> ("OldVal"=w422:bool, "NewVal"=w426:bool)  [unwired: 1 in, 4 out]
            n177 = property on="Samp_Atmos" class="Bool (strict)"() -> ("Value"=w425:bool)  [unwired: 2 in, 2 out]
            n178 = And(x=w426, y=w425) -> (x .and. y?=w424:bool)
            n179 = Not(x=w424) -> (.not. x?=w423:bool)
            n180 = case shown="True" w423 {
              tunnel: w426 -> [_ w429]
              tunnel: w422 -> [w428 _]
              frame False {
                n181 = property on="Fore_Samp" class="Bool (strict)"("Value"=w428) -> (error out=w427:errorcluster)  [unwired: 2 in, 1 out]
                n182 = call "Display Message to User8"("error in (no error)"=w427) -> ()  [unwired: 9 in, 2 out]
              }
              frame True {
                n183 = case shown="True" w429 {
                  frame False {
                    n184 = call "setDO.vi"("channel"=7, "on/off"=FALSE) -> ()  [unwired: 9 in, 1 out]
                  }
                  frame True {
                    n185 = property on="Y满" class="Bool (strict)"() -> ("Value"=w433:bool)  [unwired: 2 in, 2 out]
                    n186 = Not(x=w433) -> (.not. x?=w432:bool)
                    n187 = case shown="True" w432 {
                      frame False {
                        n188 = call "setDO.vi"("channel"=7, "on/off"=TRUE) -> ()  [unwired: 9 in, 1 out]
                      }
                      frame True {
                        n189 = call "Display Message to User"() -> ()  [unwired: 10 in, 2 out]
                      }
                    }
                  }
                }
              }
            }
          }
          event "MCPHV-Set": Value Change {
            n190 = event-data() -> ("NewVal"=w437:dbl)  [unwired: 1 in, 5 out]
            n191 = Divide(x=w437, y=2000.0) -> (x/y=w440:dbl)
            n192 = Multiply(x=w440, y=10.0) -> (x*y=w438:dbl)
            n193 = call "setAO.vi"("value"=w438, "channel"=0) -> ()  [unwired: 9 in, 1 out]
          }
          event "Tar.HV-Set": Value Change {
            n194 = event-data() -> ("NewVal"=w449:dbl)  [unwired: 1 in, 5 out]
            n195 = Divide(x=w449, y=20000.0) -> (x/y=w446:dbl)
            n196 = Multiply(x=w446, y=10.0) -> (x*y=w444:dbl)
            n197 = call "setAO.vi"("value"=w444, "channel"=1) -> ()  [unwired: 9 in, 1 out]
          }
          event "Pul.HV-Set": Value Change {
            n198 = event-data() -> ("NewVal"=w456:dbl)  [unwired: 1 in, 5 out]
            n199 = Divide(x=w456, y=2000.0) -> (x/y=w453:dbl)
            n200 = Multiply(x=w453, y=10.0) -> (x*y=w451:dbl)
            n201 = call "setAO.vi"("value"=w451, "channel"=2) -> ()  [unwired: 9 in, 1 out]
          }
          event "LensHV-Set": Value Change {
            n202 = event-data() -> ("NewVal"=w463:dbl)  [unwired: 1 in, 5 out]
            n203 = Divide(x=w463, y=10000.0) -> (x/y=w460:dbl)
            n204 = Multiply(x=w460, y=10.0) -> (x*y=w459:dbl)
            n205 = call "setAO.vi"("value"=w459, "channel"=3) -> ()  [unwired: 9 in, 1 out]
          }
          event "Image": Mouse Down {
            n206 = event-data() -> ("Coords"=w464:T16)  [unwired: 1 in, 7 out]
            n207 = property on="移动" class="Bool (strict)"() -> ("Value"=w465:bool)  [unwired: 2 in, 2 out]
            n208 = case shown="False" w465 {
              tunnel: w464 -> [w476 _]
              frame False {
                w473 = -0.005 ("x")
                n209 = Unbundle(w476) -> ("Horizontal"=w475:i32, "Vertical"=w474:i32)
                n210 = property on="X当前" class="DigNum (strict)"() -> ("Value"=w472:dbl)  [unwired: 2 in, 2 out]
                n211 = property on="Y当前" class="DigNum (strict)"() -> ("Value"=w468:dbl)  [unwired: 2 in, 2 out]
                n212 = Subtract(x=w475, y=252.0) -> (x-y=w478:dbl)
                n213 = Subtract(x=w474, y=191.0) -> (x-y=w477:dbl)
                n214 = Multiply(x=w473, y=w478) -> (x*y=w471:dbl)
                n215 = Multiply(x=w473, y=w477) -> (x*y=w469:dbl)
                n216 = Add(x=w472, y=w471) -> (x+y=w470:dbl)
                n217 = Add(x=w469, y=w468) -> (x+y=w467:dbl)
                n218 = call "goto.vi"("Y(mm)"=w467, "X(mm)"=w470) -> ()  [unwired: 9 in, 1 out]
              }
              frame True {
              }
            }
          }
          event "TakeMS-Run": Value Change {
            n219 = event-data() -> ("NewVal"=w486:bool)  [unwired: 1 in, 5 out]
            n220 = case shown="True" w486 {
              tunnel: w485 -> [_ w502]
              tunnel: w484 -> [_ w499]
              tunnel: w483 -> [_ w498]
              tunnel: w482 -> [w487 w489]
              tunnel: [w487 w488] -> w481
              frame False {
              }
              frame True {
                n221 = Unbundle By Name(w498) -> ("ConfiguredLaserCom"=w495:refnum<visa-resource-name>)
                n222 = Unbundle By Name(w499) -> ("laser semaphore"=w493:T3)
                n223 = property on="cluster" class="Clust (strict)"() -> ("Value"=w497:T7)  [unwired: 2 in, 2 out]
                n224 = Bundle By Name(cluster=w502, "ShotsPerPoint"="Shots/Point") -> (w500:T5)
                n225 = Unbundle By Name(w497) -> ("待机"=w494:bool)
                n226 = property on="SetLaserTransmission" class="Slide (strict)"() -> ("Value"=w492:dbl)  [unwired: 2 in, 2 out]
                n227 = Bundle By Name(cluster="Laser parameter", "VISA resource name"=w495, "standby"=w494, "semaphore in"=w493, "SetLaserEnergy"=w492) -> (w491:T4)
                n228 = case shown="0, Default" "AcquireMS-Methods" {
                  tunnel: w500 -> [w522 _ _]
                  tunnel: w491 -> [w523 _ _]
                  tunnel: w489 -> [w521 w532 w533]
                  tunnel: [w512 w532 w533] -> w488
                  frame 0, Default {
                    n229 = Get Date/Time String() -> (date string=w519:string, time string=w518:string)  [unwired: 3 in]
                    n230 = Concatenate Strings(w519, " " ("字符串"), w518) -> (w513:string)
                    n231 = call "Tiepie-takeData-2018-06-01.vi"("left rank"="left rank", "right rank"="right rank", "deBaseline"="deBaseline", "Thresh"="Thresh", "Laser parameter"=w523, "ADC parameter"=w522) -> ("output cluster"=w504:cluster{dbl[], "filtered data":dbl[]})  [unwired: 1 in, 1 out]
                    "MS" <- w504
                    n232 = Unbundle(w504) -> (w505:dbl[], "filtered data"=w520:dbl[])
                    n233 = property on="currentNO" class="Str"() -> ("Value"=w515:string)  [unwired: 2 in, 2 out]
                    n234 = Bundle By Name(cluster=T11 {"tag1"="", "tag2"="", "x"=[], "y"=[], "ID1:X"=[], "ID1:Y"=[], "ID1:REF:X"=[], "ID1:REF:Y"=[], "ID2:X"=[], "ID2:Y"=[], "ID2:REF:X"=[], "ID2:REF:Y"=[], "ID3:X"=[], "ID3:Y"=[], "ID3:REF:X"=[], "ID3:REF:Y"=[], "ID1:TAG1"="", "ID1:TAG2"="", "ID2:TAG1"="", "ID2:TAG2"="", "ID3:TAG1"="", "ID3:TAG2"="", "ID1:NAME"="", "ID2:NAME"="", "ID3:NAME"="", "ID1:SCORE"="", "ID2:SCORE"="", "ID3:SCORE"="", "NO"=""}, "y"=w520, "x"=w505, "tag1"="未鉴定", "tag2"=w513, "NO"=w515) -> (w514:T11)
                    n235 = Build Array (concatenate)(w521, w514) -> (w512:T8)
                    n236 = for {
                      tunnel: w512 -> [w531] mode=indexing
                      shift-right: [w524] -> w510
                      shift-left: string[][] [] ("Item Names") -> [w526]
                      i -> [w527]
                      n237 = Unbundle By Name(w531) -> ("NO"=w530:string, "tag1"=w529:string, "tag2"=w528:string)
                      n238 = Build Array(w530, w529, w528) -> (w525:string[])
                      n239 = Insert Into Array "Insert Into Array"(array=w526, index (row)=w527, new element=w525) -> (w524:string[][])  [unwired: 1 in]
                    }
                    n240 = property on="测试记录" class="MCListbox (strict)"("ItemNames"=w510) -> ()  [unwired: 2 in, 2 out]
                  }
                  frame 1 {
                  }
                  frame 2 {
                  }
                }
              }
            }
          }
          event "LaserHV", "频率/Hz", "SetLaserTransmission": Value Change {
            n241 = event-data() -> ()  [unwired: 1 in, 6 out]
            n242 = Unbundle By Name(w542) -> ("ConfiguredLaserCom"=w534:refnum<visa-resource-name>)
            n243 = Unbundle By Name(w543) -> ("laser semaphore"=w538:T3)
            n244 = call <vilib>:"Acquire Semaphore.vi"("semaphore"=w538) -> ("error out"=w537:errorcluster, "semaphore out"=w535:T3)  [unwired: 4 in, 1 out]
            n245 = call "Laser-Set-Parmeter-new.vi"("error in (no error)"=w537, "LaserHV"="LaserHV", "LaserFreq"="频率/Hz", "SetTransmission"="SetLaserTransmission", "VISA resource name"=w534) -> ("error out"=w536:errorcluster)  [unwired: 1 in, 1 out]
            n246 = call <vilib>:"Release Semaphore.vi"("error in (no error)"=w536, "semaphore"=w535) -> ()  [unwired: 4 in, 2 out]
          }
          event "测试记录": Shortcut Menu Selection (User) {
            n247 = event-data() -> ("ItemTag"=w547:string)  [unwired: 1 in, 7 out]
            n248 = case shown="\"鉴定\"" w547 {
              tunnel: w546 -> [w548 w555 w562 w567]
              tunnel: [w548 w555 w562 w563] -> w545
              frame "假", Default {
              }
              frame "鉴定" {
                n249 = property on="selected row" class="DigNum (strict)"() -> ("Value"=w551:i32)  [unwired: 2 in, 2 out]
                n250 = Index Array(array=w555, index=w551) -> (element=w561:T11)
                n251 = Unbundle By Name(w561) -> ("x"=w560:dbl[], "y"=w556:dbl[])
                n252 = call-poly <userlib>:"CaLabPut.vi"("Values"=w560, "PV Names"="MS:X") -> ("Error out"=w558:errorcluster)  [unwired: 6 in, 3 out]
                n253 = call-poly <userlib>:"CaLabPut.vi"("Error in (no error)"=w558, "Values"=w556, "PV Names"="MS:Y") -> ("Error out"=w554:errorcluster)  [unwired: 5 in, 3 out]
                n254 = call-poly <userlib>:"CaLabPut.vi"("Error in (no error)"=w554, "Value"=w551, "PV Name"="MS:NUM") -> ("Error out"=w553:errorcluster)  [unwired: 5 in, 3 out]
                n255 = call-poly <userlib>:"CaLabPut.vi"("Error in (no error)"=w553, "Value"=1, "PV Name"="MS:START") -> ()  [unwired: 5 in, 4 out]
              }
              frame "参数" {
              }
              frame "删除" {
                n256 = property on="selected row" class="DigNum (strict)"() -> ("Value"=w566:i32)  [unwired: 2 in, 2 out]
                n257 = Delete From Array "Delete From Array"(array=w567, index=w566) -> (array with subset deleted=w563:T8)  [unwired: 1 in, 1 out]
                n258 = for {
                  tunnel: w563 -> [w575] mode=indexing
                  shift-right: [w568] -> w564
                  shift-left: string[][] [] ("Item Names") -> [w570]
                  i -> [w571]
                  n259 = Unbundle By Name(w575) -> ("NO"=w574:string, "tag1"=w573:string, "tag2"=w572:string)
                  n260 = Build Array(w574, w573, w572) -> (w569:string[])
                  n261 = Insert Into Array "Insert Into Array"(array=w570, index (row)=w571, new element=w569) -> (w568:string[][])  [unwired: 1 in]
                }
                n262 = property on="测试记录" class="MCListbox (strict)"("ItemNames"=w564) -> ()  [unwired: 2 in, 2 out]
              }
            }
          }
          event "测试记录": Mouse Down {
            n263 = event-data() -> ("Coords"=w581:T16)  [unwired: 1 in, 7 out]
            n264 = invoke on="测试记录" class="MCListbox (严格)" method="Point To Row Column"("Point"=w581) -> ("CellPosition"=w580:T17)  [unwired: 6 in, 6 out]
            n265 = Unbundle By Name(w580) -> ("Row"=w577:i32)
            n266 = Array Size(array=w576) -> (size(s)=w579:i32)
            n267 = Greater Or Equal?(x=w579, y=w577) -> (x >= y?=w578:bool)
            n268 = case shown="True" w578 {
              tunnel: w577 -> [_ w608]
              tunnel: w576 -> [_ w609]
              frame False {
              }
              frame True {
                n269 = property on="selected row" class="DigNum (strict)"("Value"=w608) -> ()  [unwired: 2 in, 2 out]
                n270 = Index Array(array=w609, index=w608) -> (element=w607:T11)
                n271 = Unbundle By Name(w607) -> ("ID1:TAG1"=w590:string, "ID1:TAG2"=w604:string, "ID1:NAME"=w603:string, "ID1:SCORE"=w594:string, "ID2:TAG1"=w588:string, "ID2:TAG2"=w601:string, "ID2:NAME"=w600:string, "ID2:SCORE"=w593:string, "ID3:TAG1"=w586:string, "ID3:TAG2"=w585:string, "ID3:NAME"=w584:string, "ID3:SCORE"=w583:string)
                n272 = Build Array("1" ("element"), w590, w604, w603, w594) -> (w602:string[])
                n273 = Build Array("2" ("element"), w588, w601, w600, w593) -> (w597:string[])
                n274 = Build Array("3" ("element"), w586, w585, w584, w583) -> (w592:string[])
                n275 = Insert Into Array(array=string[][] [] ("项名"), index (row)=0 ("索引 (行)"), new element=w602) -> (w599:string[][])  [unwired: 1 in]
                n276 = Insert Into Array(array=w599, index (row)=1 ("索引 (行)"), new element=w597) -> (w596:string[][])  [unwired: 1 in]
                n277 = Insert Into Array(array=w596, index (row)=2 ("索引 (行)"), new element=w592) -> (w591:string[][])  [unwired: 1 in]
                n278 = property on="Identification Results (单靶鉴定结果)" class="MCListbox (strict)"("ItemNames"=w591) -> ()  [unwired: 2 in, 2 out]
              }
            }
          }
          event "Identification Results (单靶鉴定结果)": Mouse Down {
            n279 = event-data() -> ("Coords"=w615:T16)  [unwired: 1 in, 7 out]
            n280 = invoke on="Identification Results (单靶鉴定结果)" class="MCListbox (严格)" method="Point To Row Column"("Point"=w615) -> ("CellPosition"=w614:T17)  [unwired: 6 in, 6 out]
            n281 = Unbundle By Name(w614) -> ("Row"=w610:i32)
            n282 = Less Or Equal?(x=w610, y=2) -> (x <= y?=w612:bool)
            n283 = case shown="True" w612 {
              tunnel: w611 -> [_ w622]
              tunnel: w610 -> [_ w616]
              frame False {
              }
              frame True {
                n284 = property on="selected row" class="DigNum (strict)"() -> ("Value"=w621:i32)  [unwired: 2 in, 2 out]
                n285 = Index Array(array=w622, index=w621) -> (element=w620:T11)
                n286 = case shown="2" w616 {
                  tunnel: w620 -> [w628 w640 w649]
                  tunnel: [w627 w636 w645] -> w619
                  tunnel: [w626 w635 w644] -> w617
                  frame 0, Default {
                    n287 = Unbundle By Name(w628) -> ("x"=w630:dbl[], "y"=w629:dbl[], "ID1:REF:X"=w631:dbl[], "ID1:REF:Y"=w625:dbl[])
                    n288 = Multiply(x=w625, y=-1.0) -> (x*y=w623:dbl[])
                    n289 = Bundle("x"=w630, "y"=w629) -> (w627:cluster{"x":dbl[], "y":dbl[]})  [unwired: 1 in]
                    n290 = Bundle("ID1:REF:X"=w631, w623) -> (w626:cluster{"ID1:REF:X":dbl[], dbl[]})  [unwired: 1 in]
                  }
                  frame 1 {
                    n291 = Unbundle By Name(w640) -> ("x"=w638:dbl[], "y"=w637:dbl[], "ID2:REF:X"=w639:dbl[], "ID2:REF:Y"=w634:dbl[])
                    n292 = Multiply(x=w634, y=-1.0) -> (x*y=w632:dbl[])
                    n293 = Bundle("x"=w638, "y"=w637) -> (w636:cluster{"x":dbl[], "y":dbl[]})  [unwired: 1 in]
                    n294 = Bundle("ID2:REF:X"=w639, w632) -> (w635:cluster{"ID2:REF:X":dbl[], dbl[]})  [unwired: 1 in]
                  }
                  frame 2 {
                    n295 = Unbundle By Name(w649) -> ("x"=w647:dbl[], "y"=w646:dbl[], "ID3:REF:X"=w648:dbl[], "ID3:REF:Y"=w643:dbl[])
                    n296 = Multiply(x=w643, y=-1.0) -> (x*y=w641:dbl[])
                    n297 = Bundle("x"=w647, "y"=w646) -> (w645:cluster{"x":dbl[], "y":dbl[]})  [unwired: 1 in]
                    n298 = Bundle("ID3:REF:X"=w648, w641) -> (w644:cluster{"ID3:REF:X":dbl[], dbl[]})  [unwired: 1 in]
                  }
                }
                n299 = Build Array(w619, w617) -> (→"Identify Spcetrum":cluster{"ID3:REF:X":dbl[], "y":dbl[]}[])
              }
            }
          }
          event "Plat_To_Zero": Value Change {
            n300 = event-data() -> ("NewVal"=w651:bool)  [unwired: 1 in, 5 out]
            n301 = case shown="False" w651 {
              frame False {
              }
              frame True {
                (unwired) TRUE ("plat zeroed")
                n302 = call "plate_cal.vi"() -> ()  [unwired: 11 in, 1 out]
              }
            }
          }
          event "GO": Value Change {
            n303 = event-data() -> ("NewVal"=w654:bool)  [unwired: 1 in, 5 out]
            n304 = property on="移动" class="Bool (strict)"() -> ("Value"=w656:bool)  [unwired: 2 in, 2 out]
            n305 = Not(x=w656) -> (.not. x?=w655:bool)
            n306 = And(x=w655, y=w654) -> (x .and. y?=w653:bool)
            n307 = case shown="True" w653 {
              frame False {
              }
              frame True {
                n308 = property on="X" class="DigNum (strict)"() -> ("Value"=w658:dbl)  [unwired: 2 in, 2 out]
                n309 = property on="Y" class="DigNum (strict)"() -> ("Value"=w657:dbl)  [unwired: 2 in, 2 out]
                n310 = call "goto.vi"("Y(mm)"=w657, "X(mm)"=w658) -> ()  [unwired: 9 in, 1 out]
              }
            }
          }
          event "chamber in": Value Change {
            n311 = event-data() -> ("NewVal"=w661:bool)  [unwired: 1 in, 5 out]
            n312 = property on="HVEnable" class="Bool (strict)"() -> ("Value"=w666:bool)  [unwired: 2 in, 2 out]
            n313 = property on="Y满" class="Bool (strict)"() -> ("Value"=w662:bool)  [unwired: 2 in, 2 out]
            n314 = property on="移动" class="Bool (strict)"() -> ("Value"=w665:bool)  [unwired: 2 in, 2 out]
            n315 = Not(x=w666) -> (.not. x?=w663:bool)
            n316 = Not(x=w665) -> (.not. x?=w664:bool)
            n317 = Compound Arithmetic op=AND(w663, w662, w664, w661) -> (w660:bool)
            n318 = case shown="True" w660 {
              frame False {
              }
              frame True {
                n319 = flat-sequence {
                  tunnel: [w671] -> w667
                  tunnel: w667 -> [w681]
                  frame #0 {
                    n320 = call "样品标识与备注"() -> ("备注"=w668:string, "样品名称"=w669:string)  [unwired: 16 in, 2 out]
                    n321 = property on="sampleID" class="Str"("Value"=w669) -> ()  [unwired: 2 in, 2 out]
                    n322 = property on="commet" class="Str"("Value"=w668) -> ()  [unwired: 2 in, 2 out]
                  }
                  frame #1 {
                    w672 = FALSE ("on/off")
                    # "关样仓/大气"
                    n323 = Wait (ms)(milliseconds to wait=1500) -> ()  [unwired: 1 out]
                    n324 = call "setDO.vi"("channel"=6, "on/off"=w672) -> ("错误输出"=w670:errorcluster)  [unwired: 9 in]
                    n325 = property on="Samp_Atmos" class="Bool (strict)"(error in=w670, "Value"=w672) -> (error out=w671:errorcluster)  [unwired: 1 in, 1 out]
                  }
                  frame #2 {
                    # "开前泵/样仓"
                    n326 = call "setDO.vi"("错误输入（无错误）"=w681, "channel"=7, "on/off"=TRUE) -> ("错误输出"=w680:errorcluster)  [unwired: 8 in]
                    n327 = flat-sequence {
                      tunnel: w680 -> [w691]
                      tunnel: [w691] -> w676
                      frame #0 {
                        n328 = Wait (ms)(milliseconds to wait=10000) -> ()  [unwired: 1 out]
                      }
                    }
                    n329 = property on="Lvaccum" class="DigNum (strict)"(error in=w676) -> (error out=w675:errorcluster, "Value"=w679:dbl)  [unwired: 1 in, 1 out]
                    n330 = Less?(x=w679, y=10) -> (x < y?=w677:bool)
                    n331 = case shown="False" w677 {
                      tunnel: w675 -> [w685 w687]
                      frame False {
                        (unwired) 7
                        n332 = call "setDO.vi"("错误输入（无错误）"=w685, "on/off"=FALSE) -> ("错误输出"=w684:errorcluster)  [unwired: 9 in]
                        n333 = call "Display Message to User4"("error in (no error)"=w684) -> ()  [unwired: 9 in, 2 out]
                      }
                      frame True {
                        n334 = flat-sequence {
                          tunnel: w687 -> [w688]
                          frame #0 {
                            n335 = call "setDO.vi"("错误输入（无错误）"=w688, "channel"=7, "on/off"=FALSE) -> ()  [unwired: 8 in, 1 out]
                          }
                          frame #1 {
                            n336 = call "chamber_in.vi"() -> ()  [unwired: 12 in]
                          }
                        }
                      }
                    }
                  }
                }
              }
            }
          }
          event "chamber out": Value Change {
            n337 = event-data() -> ("NewVal"=w693:bool)  [unwired: 1 in, 5 out]
            n338 = case shown="True" w693 {
              frame False {
              }
              frame True {
                n339 = property on="移动" class="Bool (strict)"() -> ("Value"=w699:bool)  [unwired: 2 in, 2 out]
                n340 = property on="Y满" class="Bool (strict)"() -> ("Value"=w700:bool)  [unwired: 2 in, 2 out]
                n341 = property on="HVEnable" class="Bool (strict)"() -> ("Value"=w701:bool)  [unwired: 2 in, 2 out]
                n342 = Not "非"(x=w699) -> (.not. x?=w697:bool)
                n343 = Not "非"(x=w700) -> (.not. x?=w698:bool)
                n344 = Not "非"(x=w701) -> (.not. x?=w695:bool)
                n345 = Compound Arithmetic op=AND "复合运算"(w695, w698, w697) -> (w696:bool)
                n346 = case shown="True" w696 {
                  frame False {
                    n347 = call "Display Message to User3"() -> ()  [unwired: 10 in, 2 out]
                  }
                  frame True {
                    n348 = flat-sequence {
                      tunnel: [w705] -> w703
                      tunnel: w703 -> [w711]
                      tunnel: [w712] -> w702
                      tunnel: w702 -> [w723]
                      frame #0 {
                        n349 = call "chamber_out.vi"() -> ()  [unwired: 12 in]
                      }
                      frame #1 {
                        w706 = FALSE ("on/off")
                        # "关前泵/样仓"
                        n350 = Wait (ms)(milliseconds to wait=1500) -> ()  [unwired: 1 out]
                        n351 = call "setDO.vi"("channel"=7, "on/off"=w706) -> ("错误输出"=w704:errorcluster)  [unwired: 9 in]
                        n352 = property on="Fore_Samp" class="Bool (strict)"(error in=w704, "Value"=w706) -> (error out=w705:errorcluster)  [unwired: 1 in, 1 out]
                      }
                      frame #2 {
                        # "开样仓/大气"
                        n353 = call "Time Delay4"("error in (no error)"=w711, "Delay Time (s)"=3.0) -> ("error out"=w710:errorcluster)  [unwired: 9 in]
                        n354 = property on="Y满" class="Bool (strict)"(error in=w710) -> (error out=w713:errorcluster, "Value"=w714:bool)  [unwired: 1 in, 1 out]
                        n355 = case shown="True" w714 {
                          tunnel: w713 -> [w716 w718]
                          tunnel: [w715 w717] -> w712
                          frame False {
                            n356 = call "Display Message to User2"("error in (no error)"=w716) -> ("error out"=w715:errorcluster)  [unwired: 9 in, 1 out]
                          }
                          frame True {
                            n357 = call "setDO.vi"("错误输入（无错误）"=w718, "channel"=6, "on/off"=TRUE) -> ("错误输出"=w717:errorcluster)  [unwired: 8 in]
                          }
                        }
                      }
                      frame #3 {
                        n358 = call "Time Delay5"("error in (no error)"=w723, "Delay Time (s)"=3.0) -> ("error out"=w722:errorcluster)  [unwired: 9 in]
                        n359 = call "setDO.vi"("错误输入（无错误）"=w722, "channel"=6, "on/off"=FALSE) -> ()  [unwired: 8 in, 1 out]
                      }
                    }
                  }
                }
              }
            }
          }
          event "标准样品": Value Change {
            n360 = event-data() -> ("NewVal"=w727:u16)  [unwired: 1 in, 5 out]
            n361 = control-ref of="定标参数"() -> (w728:refnum<vi>)
            n362 = local read "std sample"() -> (w726:T1)
            n363 = call "writetable.vi"("std sample"=w726, "type"=w727, "reference"=w728) -> ()  [unwired: 9 in]
          }
          event "peak cal": Value Change {
            n364 = event-data() -> ("NewVal"=w730:bool)  [unwired: 1 in, 5 out]
            n365 = case shown="True" w730 {
              frame False {
              }
              frame True {
                n366 = property on="定标参数" class="MCListbox (strict)"() -> ("ItemNames"=w750:string[][])  [unwired: 2 in, 2 out]
                n367 = Index Array(array=w750, index (col)=1 ("disabled index (col)")) -> (element=w751:string[])  [unwired: 1 in]
                n368 = Index Array(array=w750, index (col)=3 ("disabled index (col)")) -> (element=w748:string[])  [unwired: 1 in]
                n369 = Fract/Exp String To Number(string=w751) -> (number=w740:dbl[])  [unwired: 3 in, 1 out]
                n370 = Fract/Exp String To Number(string=w748) -> (number=w742:dbl[])  [unwired: 3 in, 1 out]
                n371 = call <vilib>:"General Polynomial Fit.vi"("Y"=w740, "polynomial order"=2, "X"=w742) -> ("Polynomial Coefficients"=w744:dbl[])  [unwired: 9 in, 3 out]
                n372 = Index Array(array=w744, index=2) -> (element=w732:dbl)
                "a:" <- w732
                n373 = Index Array(array=w744, index=1) -> (element=w733:dbl)
                "b:" <- w733
                n374 = Index Array(array=w744, index=0) -> (element=w734:dbl)
                "c:" <- w734
                n375 = global write "cal_p.vi" "a"(w732) -> ()
                n376 = global write "cal_p.vi" "b"(w733) -> ()
                n377 = for {
                  tunnel: w742 -> [w765] mode=indexing
                  tunnel: [w769] -> w741 mode=indexing
                  tunnel: w734 -> [w766]
                  tunnel: w733 -> [w767]
                  tunnel: w732 -> [w768]
                  n378 = formula code="m=a*x*x+b*x+c;"("a"=w768, "b"=w767, "c"=w766, "x"=w765) -> ("m"=w769:dbl)
                }
                n379 = global write "cal_p.vi" "c"(w734) -> ()
                n380 = for {
                  tunnel: w741 -> [w763] mode=indexing
                  tunnel: w740 -> [w764] mode=indexing
                  tunnel: [w762] -> w735 mode=indexing
                  n381 = formula code="delta=100*(m-m0)/m0;"("m0"=w764, "m"=w763) -> ("delta"=w762:dbl)
                }
                n382 = control-ref of="定标参数"() -> (w739:refnum<vi>)
                n383 = property on="Property Node" class="MCListbox (strict)"(reference=w739) -> (reference out=w738:refnum<vi>, "ItemNames"=w737:string[][])  [unwired: 1 in, 1 out]
                n384 = for {
                  shift-right: [w758] -> w736
                  shift-left: w737 -> [w761]
                  tunnel: w735 -> [w759] mode=indexing
                  i -> [w760]
                  n385 = Number To Fractional String(number=w759, precision (6)=i16 2) -> (F-format string=w756:string)  [unwired: 2 in]
                  n386 = Concatenate Strings(w756, "%" ("string")) -> (w754:string)
                  n387 = Replace Array Subset(array=w761, new element=w754, index (row)=w760, index (col)=4 ("disabled index (col)")) -> (w758:string[][])
                }
                n388 = property on="Property Node" class="MCListbox (strict)"(reference=w738, "ItemNames"=w736) -> ()  [unwired: 1 in, 2 out]
              }
            }
          }
          event "A1-Position": Value Change {
            n389 = event-data() -> ("NewVal"=w771:bool)  [unwired: 1 in, 5 out]
            n390 = case shown="True" w771 {
              frame False {
              }
              frame True {
                n391 = property on="X当前" class="DigNum (strict)"() -> ("Value"=→"A1-position-X":dbl)  [unwired: 2 in, 2 out]
                n392 = property on="Y当前" class="DigNum (strict)"() -> ("Value"=→"A1-position-Y":dbl)  [unwired: 2 in, 2 out]
              }
            }
          }
          event "A1": Value Change {
            n393 = event-data() -> ("NewVal"=w777:bool)  [unwired: 1 in, 5 out]
            n394 = property on="移动" class="Bool (strict)"() -> ("Value"=w779:bool)  [unwired: 2 in, 2 out]
            n395 = Not(x=w779) -> (.not. x?=w778:bool)
            n396 = And(x=w778, y=w777) -> (x .and. y?=w776:bool)
            n397 = case shown="True" w776 {
              frame False {
              }
              frame True {
                n398 = property on="A1-position-X" class="DigNum (strict)"() -> (error out=w784:errorcluster, "Value"=w782:dbl)  [unwired: 2 in, 1 out]
                n399 = property on="A1-position-Y" class="DigNum (strict)"(error in=w784) -> (error out=w783:errorcluster, "Value"=w781:dbl)  [unwired: 1 in, 1 out]
                n400 = vi-ref "goto.vi"() -> (w788:refnum<vi>)
                n401 = property class="VI"(reference=w788, error in=w783) -> ("Name"=w787:string)  [unwired: 2 out]
                n402 = Open VI Reference(type specifier VI Refnum (for type only)=refnum<vi> refnum, vi path=w787, options=128) -> (vi reference=w785:refnum<vi>)  [unwired: 3 in, 1 out]
                n403 = call-by-ref "Start Asynchronous Call"(reference=w785, "Y(mm)"=w781, "X(mm)"=w782) -> ()  [unwired: 10 in, 3 out]
              }
            }
            n404 = property on="currentNO" class="Str"("Value"="A1") -> ()  [unwired: 2 in, 2 out]
          }
          event "A2": Value Change {
            n405 = event-data() -> ("NewVal"=w792:bool)  [unwired: 1 in, 5 out]
            n406 = property on="移动" class="Bool (strict)"() -> ("Value"=w795:bool)  [unwired: 2 in, 2 out]
            n407 = Not(x=w795) -> (.not. x?=w794:bool)
            n408 = And(x=w794, y=w792) -> (x .and. y?=w793:bool)
            n409 = case shown="True" w793 {
              frame False {
              }
              frame True {
                n410 = property on="A1-position-X" class="DigNum (strict)"() -> (error out=w799:errorcluster, "Value"=w806:dbl)  [unwired: 2 in, 1 out]
                n411 = property on="A1-position-Y" class="DigNum (strict)"(error in=w799) -> (error out=w798:errorcluster, "Value"=w796:dbl)  [unwired: 1 in, 1 out]
                n412 = Subtract(x=w806, y=4.5) -> (x-y=w797:dbl)
                n413 = vi-ref "goto.vi"() -> (w804:refnum<vi>)
                n414 = property class="VI"(reference=w804, error in=w798) -> ("Name"=w803:string)  [unwired: 2 out]
                n415 = Open VI Reference(type specifier VI Refnum (for type only)=refnum<vi> refnum, vi path=w803, options=128) -> (vi reference=w801:refnum<vi>)  [unwired: 3 in, 1 out]
                n416 = call-by-ref "Start Asynchronous Call"(reference=w801, "Y(mm)"=w796, "X(mm)"=w797) -> ()  [unwired: 10 in, 3 out]
              }
            }
            n417 = control-ref of="currentNO"() -> (w789:refnum<vi>)
            n418 = property on="属性节点" class="Str"(reference=w789, "Value"="A2") -> ()  [unwired: 1 in, 2 out]
          }
          event "A3": Value Change {
            n419 = event-data() -> ("NewVal"=w810:bool)  [unwired: 1 in, 5 out]
            n420 = property on="移动" class="Bool (strict)"() -> ("Value"=w813:bool)  [unwired: 2 in, 2 out]
            n421 = Not(x=w813) -> (.not. x?=w812:bool)
            n422 = And(x=w812, y=w810) -> (x .and. y?=w811:bool)
            n423 = case shown="True" w811 {
              frame False {
              }
              frame True {
                n424 = property on="A1-position-X" class="DigNum (strict)"() -> (error out=w817:errorcluster, "Value"=w824:dbl)  [unwired: 2 in, 1 out]
                n425 = property on="A1-position-Y" class="DigNum (strict)"(error in=w817) -> (error out=w816:errorcluster, "Value"=w814:dbl)  [unwired: 1 in, 1 out]
                n426 = Subtract(x=w824, y=9.0) -> (x-y=w815:dbl)
                n427 = vi-ref "goto.vi"() -> (w822:refnum<vi>)
                n428 = property class="VI"(reference=w822, error in=w816) -> ("Name"=w821:string)  [unwired: 2 out]
                n429 = Open VI Reference(type specifier VI Refnum (for type only)=refnum<vi> refnum, vi path=w821, options=128) -> (vi reference=w819:refnum<vi>)  [unwired: 3 in, 1 out]
                n430 = call-by-ref "Start Asynchronous Call"(reference=w819, "Y(mm)"=w814, "X(mm)"=w815) -> ()  [unwired: 10 in, 3 out]
              }
            }
            n431 = control-ref of="currentNO"() -> (w807:refnum<vi>)
            n432 = property on="属性节点" class="Str"(reference=w807, "Value"="A3") -> ()  [unwired: 1 in, 2 out]
          }
          event "A4": Value Change {
            n433 = event-data() -> ("NewVal"=w827:bool)  [unwired: 1 in, 5 out]
            n434 = property on="移动" class="Bool (strict)"() -> ("Value"=w830:bool)  [unwired: 2 in, 2 out]
            n435 = Not(x=w830) -> (.not. x?=w829:bool)
            n436 = And(x=w829, y=w827) -> (x .and. y?=w828:bool)
            n437 = case shown="True" w828 {
              frame False {
              }
              frame True {
                n438 = property on="A1-position-X" class="DigNum (strict)"() -> (error out=w834:errorcluster, "Value"=w841:dbl)  [unwired: 2 in, 1 out]
                n439 = property on="A1-position-Y" class="DigNum (strict)"(error in=w834) -> (error out=w833:errorcluster, "Value"=w831:dbl)  [unwired: 1 in, 1 out]
                n440 = Subtract(x=w841, y=13.5) -> (x-y=w832:dbl)
                n441 = vi-ref "goto.vi"() -> (w839:refnum<vi>)
                n442 = property class="VI"(reference=w839, error in=w833) -> ("Name"=w838:string)  [unwired: 2 out]
                n443 = Open VI Reference(type specifier VI Refnum (for type only)=refnum<vi> refnum, vi path=w838, options=128) -> (vi reference=w836:refnum<vi>)  [unwired: 3 in, 1 out]
                n444 = call-by-ref "Start Asynchronous Call"(reference=w836, "Y(mm)"=w831, "X(mm)"=w832) -> ()  [unwired: 10 in, 3 out]
              }
            }
            n445 = property on="currentNO" class="Str"("Value"="A4") -> ()  [unwired: 2 in, 2 out]
          }
          event "A5": Value Change {
            n446 = event-data() -> ("NewVal"=w844:bool)  [unwired: 1 in, 5 out]
            n447 = property on="移动" class="Bool (strict)"() -> ("Value"=w847:bool)  [unwired: 2 in, 2 out]
            n448 = Not(x=w847) -> (.not. x?=w846:bool)
            n449 = And(x=w846, y=w844) -> (x .and. y?=w845:bool)
            n450 = case shown="True" w845 {
              frame False {
              }
              frame True {
                n451 = property on="A1-position-X" class="DigNum (strict)"() -> (error out=w851:errorcluster, "Value"=w858:dbl)  [unwired: 2 in, 1 out]
                n452 = property on="A1-position-Y" class="DigNum (strict)"(error in=w851) -> (error out=w850:errorcluster, "Value"=w848:dbl)  [unwired: 1 in, 1 out]
                n453 = Subtract(x=w858, y=18) -> (x-y=w849:dbl)
                n454 = vi-ref "goto.vi"() -> (w856:refnum<vi>)
                n455 = property class="VI"(reference=w856, error in=w850) -> ("Name"=w855:string)  [unwired: 2 out]
                n456 = Open VI Reference(type specifier VI Refnum (for type only)=refnum<vi> refnum, vi path=w855, options=128) -> (vi reference=w853:refnum<vi>)  [unwired: 3 in, 1 out]
                n457 = call-by-ref "Start Asynchronous Call"(reference=w853, "Y(mm)"=w848, "X(mm)"=w849) -> ()  [unwired: 10 in, 3 out]
              }
            }
            n458 = property on="currentNO" class="Str"("Value"="A5") -> ()  [unwired: 2 in, 2 out]
          }
          event "A6": Value Change {
            n459 = event-data() -> ("NewVal"=w861:bool)  [unwired: 1 in, 5 out]
            n460 = property on="移动" class="Bool (strict)"() -> ("Value"=w864:bool)  [unwired: 2 in, 2 out]
            n461 = Not(x=w864) -> (.not. x?=w863:bool)
            n462 = And(x=w863, y=w861) -> (x .and. y?=w862:bool)
            n463 = case shown="True" w862 {
              frame False {
              }
              frame True {
                n464 = property on="A1-position-X" class="DigNum (strict)"() -> (error out=w868:errorcluster, "Value"=w875:dbl)  [unwired: 2 in, 1 out]
                n465 = property on="A1-position-Y" class="DigNum (strict)"(error in=w868) -> (error out=w867:errorcluster, "Value"=w865:dbl)  [unwired: 1 in, 1 out]
                n466 = Subtract(x=w875, y=22.5) -> (x-y=w866:dbl)
                n467 = vi-ref "goto.vi"() -> (w873:refnum<vi>)
                n468 = property class="VI"(reference=w873, error in=w867) -> ("Name"=w872:string)  [unwired: 2 out]
                n469 = Open VI Reference(type specifier VI Refnum (for type only)=refnum<vi> refnum, vi path=w872, options=128) -> (vi reference=w870:refnum<vi>)  [unwired: 3 in, 1 out]
                n470 = call-by-ref "Start Asynchronous Call"(reference=w870, "Y(mm)"=w865, "X(mm)"=w866) -> ()  [unwired: 10 in, 3 out]
              }
            }
            n471 = property on="currentNO" class="Str"("Value"="A6") -> ()  [unwired: 2 in, 2 out]
          }
          event "A7": Value Change {
            n472 = event-data() -> ("NewVal"=w878:bool)  [unwired: 1 in, 5 out]
            n473 = property on="移动" class="Bool (strict)"() -> ("Value"=w881:bool)  [unwired: 2 in, 2 out]
            n474 = Not(x=w881) -> (.not. x?=w880:bool)
            n475 = And(x=w880, y=w878) -> (x .and. y?=w879:bool)
            n476 = case shown="True" w879 {
              frame False {
              }
              frame True {
                n477 = property on="A1-position-X" class="DigNum (strict)"() -> (error out=w885:errorcluster, "Value"=w892:dbl)  [unwired: 2 in, 1 out]
                n478 = property on="A1-position-Y" class="DigNum (strict)"(error in=w885) -> (error out=w884:errorcluster, "Value"=w882:dbl)  [unwired: 1 in, 1 out]
                n479 = Subtract(x=w892, y=27) -> (x-y=w883:dbl)
                n480 = vi-ref "goto.vi"() -> (w890:refnum<vi>)
                n481 = property class="VI"(reference=w890, error in=w884) -> ("Name"=w889:string)  [unwired: 2 out]
                n482 = Open VI Reference(type specifier VI Refnum (for type only)=refnum<vi> refnum, vi path=w889, options=128) -> (vi reference=w887:refnum<vi>)  [unwired: 3 in, 1 out]
                n483 = call-by-ref "Start Asynchronous Call"(reference=w887, "Y(mm)"=w882, "X(mm)"=w883) -> ()  [unwired: 10 in, 3 out]
              }
            }
            n484 = property on="currentNO" class="Str"("Value"="A7") -> ()  [unwired: 2 in, 2 out]
          }
          event User Event {
            n485 = event-data() -> ("PV name"=w894:string, "value array (string)"=w893:string[])  [unwired: 1 in, 9 out]
            n486 = case shown="\"ID:STATUS\"" w894 {
              tunnel: w896 -> [w900 w906]
              tunnel: [w900 w909] -> w895
              tunnel: w893 -> [w899 _]
              frame "ID:INFO", Default {
                n487 = Index Array(array=w899, index=0) -> (element=→"idn status":string)
              }
              frame "ID:STATUS" {
                n488 = call "getIOCdata.vi"() -> ("输出簇"=w907:T11)  [unwired: 11 in]
                n489 = call-poly <userlib>:"CaLabGet.vi"("PV Name"="MS:NUM") -> ("1rst Value (number)"=w905:dbl)  [unwired: 8 in, 6 out]
                n490 = Index Array(array=w906, index=w905) -> (element=w904:T11)
                n491 = Unbundle By Name(w904) -> ("NO"=w903:string, "tag2"=w902:string)
                n492 = Bundle By Name(cluster=w907, "NO"=w903, "tag2"=w902) -> (w901:T11)
                n493 = Replace Array Subset "Replace Array Subset"(array=w906, new element=w901, index=w905) -> (w909:T8)
                n494 = for {
                  tunnel: w909 -> [w919] mode=indexing
                  shift-right: [w912] -> w908
                  shift-left: string[][] [] ("Item Names") -> [w914]
                  i -> [w915]
                  n495 = Unbundle By Name(w919) -> ("NO"=w918:string, "tag1"=w917:string, "tag2"=w916:string)
                  n496 = Build Array(w918, w917, w916) -> (w913:string[])
                  n497 = Insert Into Array "Insert Into Array"(array=w914, index (row)=w915, new element=w913) -> (w912:string[][])  [unwired: 1 in]
                }
                n498 = property on="测试记录" class="MCListbox (strict)"("ItemNames"=w908) -> ()  [unwired: 2 in, 2 out]
              }
            }
          }
          event "A8": Value Change {
            n499 = event-data() -> ("NewVal"=w922:bool)  [unwired: 1 in, 5 out]
            n500 = property on="移动" class="Bool (strict)"() -> ("Value"=w925:bool)  [unwired: 2 in, 2 out]
            n501 = Not(x=w925) -> (.not. x?=w924:bool)
            n502 = And(x=w924, y=w922) -> (x .and. y?=w923:bool)
            n503 = case shown="False" w923 {
              frame False {
              }
              frame True {
                n504 = property on="A1-position-X" class="DigNum (strict)"() -> (error out=w929:errorcluster, "Value"=w936:dbl)  [unwired: 2 in, 1 out]
                n505 = property on="A1-position-Y" class="DigNum (strict)"(error in=w929) -> (error out=w928:errorcluster, "Value"=w926:dbl)  [unwired: 1 in, 1 out]
                n506 = Subtract(x=w936, y=31.5) -> (x-y=w927:dbl)
                n507 = vi-ref "goto.vi"() -> (w934:refnum<vi>)
                n508 = property class="VI"(reference=w934, error in=w928) -> ("Name"=w933:string)  [unwired: 2 out]
                n509 = Open VI Reference(type specifier VI Refnum (for type only)=refnum<vi> refnum, vi path=w933, options=128) -> (vi reference=w931:refnum<vi>)  [unwired: 3 in, 1 out]
                n510 = call-by-ref "Start Asynchronous Call"(reference=w931, "Y(mm)"=w926, "X(mm)"=w927) -> ()  [unwired: 10 in, 3 out]
              }
            }
            n511 = property on="currentNO" class="Str"("Value"="A8") -> ()  [unwired: 2 in, 2 out]
          }
          event "A9": Value Change {
            n512 = event-data() -> ("NewVal"=w939:bool)  [unwired: 1 in, 5 out]
            n513 = property on="移动" class="Bool (strict)"() -> ("Value"=w942:bool)  [unwired: 2 in, 2 out]
            n514 = Not(x=w942) -> (.not. x?=w941:bool)
            n515 = And(x=w941, y=w939) -> (x .and. y?=w940:bool)
            n516 = case shown="True" w940 {
              frame False {
              }
              frame True {
                n517 = property on="A1-position-X" class="DigNum (strict)"() -> (error out=w946:errorcluster, "Value"=w953:dbl)  [unwired: 2 in, 1 out]
                n518 = property on="A1-position-Y" class="DigNum (strict)"(error in=w946) -> (error out=w945:errorcluster, "Value"=w943:dbl)  [unwired: 1 in, 1 out]
                n519 = Subtract(x=w953, y=36) -> (x-y=w944:dbl)
                n520 = vi-ref "goto.vi"() -> (w951:refnum<vi>)
                n521 = property class="VI"(reference=w951, error in=w945) -> ("Name"=w950:string)  [unwired: 2 out]
                n522 = Open VI Reference(type specifier VI Refnum (for type only)=refnum<vi> refnum, vi path=w950, options=128) -> (vi reference=w948:refnum<vi>)  [unwired: 3 in, 1 out]
                n523 = call-by-ref "Start Asynchronous Call"(reference=w948, "Y(mm)"=w943, "X(mm)"=w944) -> ()  [unwired: 10 in, 3 out]
              }
            }
            n524 = property on="currentNO" class="Str"("Value"="A9") -> ()  [unwired: 2 in, 2 out]
          }
          event "A10": Value Change {
            n525 = event-data() -> ("NewVal"=w956:bool)  [unwired: 1 in, 5 out]
            n526 = property on="移动" class="Bool (strict)"() -> ("Value"=w959:bool)  [unwired: 2 in, 2 out]
            n527 = Not(x=w959) -> (.not. x?=w958:bool)
            n528 = And(x=w958, y=w956) -> (x .and. y?=w957:bool)
            n529 = case shown="True" w957 {
              frame False {
              }
              frame True {
                n530 = property on="A1-position-X" class="DigNum (strict)"() -> (error out=w963:errorcluster, "Value"=w970:dbl)  [unwired: 2 in, 1 out]
                n531 = property on="A1-position-Y" class="DigNum (strict)"(error in=w963) -> (error out=w962:errorcluster, "Value"=w960:dbl)  [unwired: 1 in, 1 out]
                n532 = Subtract(x=w970, y=40.5) -> (x-y=w961:dbl)
                n533 = vi-ref "goto.vi"() -> (w968:refnum<vi>)
                n534 = property class="VI"(reference=w968, error in=w962) -> ("Name"=w967:string)  [unwired: 2 out]
                n535 = Open VI Reference(type specifier VI Refnum (for type only)=refnum<vi> refnum, vi path=w967, options=128) -> (vi reference=w965:refnum<vi>)  [unwired: 3 in, 1 out]
                n536 = call-by-ref "Start Asynchronous Call"(reference=w965, "Y(mm)"=w960, "X(mm)"=w961) -> ()  [unwired: 10 in, 3 out]
              }
            }
            n537 = property on="currentNO" class="Str"("Value"="A10") -> ()  [unwired: 2 in, 2 out]
          }
          event "A11": Value Change {
            n538 = event-data() -> ("NewVal"=w973:bool)  [unwired: 1 in, 5 out]
            n539 = property on="移动" class="Bool (strict)"() -> ("Value"=w976:bool)  [unwired: 2 in, 2 out]
            n540 = Not(x=w976) -> (.not. x?=w975:bool)
            n541 = And(x=w975, y=w973) -> (x .and. y?=w974:bool)
            n542 = case shown="True" w974 {
              frame False {
              }
              frame True {
                n543 = property on="A1-position-X" class="DigNum (strict)"() -> (error out=w980:errorcluster, "Value"=w987:dbl)  [unwired: 2 in, 1 out]
                n544 = property on="A1-position-Y" class="DigNum (strict)"(error in=w980) -> (error out=w979:errorcluster, "Value"=w977:dbl)  [unwired: 1 in, 1 out]
                n545 = Subtract(x=w987, y=45) -> (x-y=w978:dbl)
                n546 = vi-ref "goto.vi"() -> (w985:refnum<vi>)
                n547 = property class="VI"(reference=w985, error in=w979) -> ("Name"=w984:string)  [unwired: 2 out]
                n548 = Open VI Reference(type specifier VI Refnum (for type only)=refnum<vi> refnum, vi path=w984, options=128) -> (vi reference=w982:refnum<vi>)  [unwired: 3 in, 1 out]
                n549 = call-by-ref "Start Asynchronous Call"(reference=w982, "Y(mm)"=w977, "X(mm)"=w978) -> ()  [unwired: 10 in, 3 out]
              }
            }
            n550 = property on="currentNO" class="Str"("Value"="A11") -> ()  [unwired: 2 in, 2 out]
          }
          event "A12": Value Change {
            n551 = event-data() -> ("NewVal"=w990:bool)  [unwired: 1 in, 5 out]
            n552 = property on="移动" class="Bool (strict)"() -> ("Value"=w993:bool)  [unwired: 2 in, 2 out]
            n553 = Not(x=w993) -> (.not. x?=w992:bool)
            n554 = And(x=w992, y=w990) -> (x .and. y?=w991:bool)
            n555 = case shown="True" w991 {
              frame False {
              }
              frame True {
                n556 = property on="A1-position-X" class="DigNum (strict)"() -> (error out=w997:errorcluster, "Value"=w1004:dbl)  [unwired: 2 in, 1 out]
                n557 = property on="A1-position-Y" class="DigNum (strict)"(error in=w997) -> (error out=w996:errorcluster, "Value"=w994:dbl)  [unwired: 1 in, 1 out]
                n558 = Subtract(x=w1004, y=49.5) -> (x-y=w995:dbl)
                n559 = vi-ref "goto.vi"() -> (w1002:refnum<vi>)
                n560 = property class="VI"(reference=w1002, error in=w996) -> ("Name"=w1001:string)  [unwired: 2 out]
                n561 = Open VI Reference(type specifier VI Refnum (for type only)=refnum<vi> refnum, vi path=w1001, options=128) -> (vi reference=w999:refnum<vi>)  [unwired: 3 in, 1 out]
                n562 = call-by-ref "Start Asynchronous Call"(reference=w999, "Y(mm)"=w994, "X(mm)"=w995) -> ()  [unwired: 10 in, 3 out]
              }
            }
            n563 = property on="currentNO" class="Str"("Value"="A12") -> ()  [unwired: 2 in, 2 out]
          }
          event "B1": Value Change {
            n564 = event-data() -> ("NewVal"=w1007:bool)  [unwired: 1 in, 5 out]
            n565 = property on="移动" class="Bool (strict)"() -> ("Value"=w1010:bool)  [unwired: 2 in, 2 out]
            n566 = Not(x=w1010) -> (.not. x?=w1009:bool)
            n567 = And(x=w1009, y=w1007) -> (x .and. y?=w1008:bool)
            n568 = case shown="True" w1008 {
              frame False {
              }
              frame True {
                n569 = property on="A1-position-X" class="DigNum (strict)"() -> (error out=w1016:errorcluster, "Value"=w1023:dbl)  [unwired: 2 in, 1 out]
                n570 = property on="A1-position-Y" class="DigNum (strict)"(error in=w1016) -> (error out=w1015:errorcluster, "Value"=w1012:dbl)  [unwired: 1 in, 1 out]
                n571 = Subtract(x=w1012, y=4.5) -> (x-y=w1011:dbl)
                n572 = Subtract(x=w1023, y=0) -> (x-y=w1014:dbl)
                n573 = vi-ref "goto.vi"() -> (w1021:refnum<vi>)
                n574 = property class="VI"(reference=w1021, error in=w1015) -> ("Name"=w1020:string)  [unwired: 2 out]
                n575 = Open VI Reference(type specifier VI Refnum (for type only)=refnum<vi> refnum, vi path=w1020, options=128) -> (vi reference=w1018:refnum<vi>)  [unwired: 3 in, 1 out]
                n576 = call-by-ref "Start Asynchronous Call"(reference=w1018, "Y(mm)"=w1011, "X(mm)"=w1014) -> ()  [unwired: 10 in, 3 out]
              }
            }
            n577 = property on="currentNO" class="Str"("Value"="B1") -> ()  [unwired: 2 in, 2 out]
          }
          event "B2": Value Change {
            n578 = event-data() -> ("NewVal"=w1026:bool)  [unwired: 1 in, 5 out]
            n579 = property on="移动" class="Bool (strict)"() -> ("Value"=w1029:bool)  [unwired: 2 in, 2 out]
            n580 = Not(x=w1029) -> (.not. x?=w1028:bool)
            n581 = And(x=w1028, y=w1026) -> (x .and. y?=w1027:bool)
            n582 = case shown="True" w1027 {
              frame False {
              }
              frame True {
                n583 = property on="A1-position-X" class="DigNum (strict)"() -> (error out=w1035:errorcluster, "Value"=w1042:dbl)  [unwired: 2 in, 1 out]
                n584 = property on="A1-position-Y" class="DigNum (strict)"(error in=w1035) -> (error out=w1034:errorcluster, "Value"=w1031:dbl)  [unwired: 1 in, 1 out]
                n585 = Subtract(x=w1031, y=4.5) -> (x-y=w1030:dbl)
                n586 = Subtract(x=w1042, y=4.5) -> (x-y=w1033:dbl)
                n587 = vi-ref "goto.vi"() -> (w1040:refnum<vi>)
                n588 = property class="VI"(reference=w1040, error in=w1034) -> ("Name"=w1039:string)  [unwired: 2 out]
                n589 = Open VI Reference(type specifier VI Refnum (for type only)=refnum<vi> refnum, vi path=w1039, options=128) -> (vi reference=w1037:refnum<vi>)  [unwired: 3 in, 1 out]
                n590 = call-by-ref "Start Asynchronous Call"(reference=w1037, "Y(mm)"=w1030, "X(mm)"=w1033) -> ()  [unwired: 10 in, 3 out]
              }
            }
            n591 = property on="currentNO" class="Str"("Value"="B2") -> ()  [unwired: 2 in, 2 out]
          }
          event "B3": Value Change {
            n592 = event-data() -> ("NewVal"=w1045:bool)  [unwired: 1 in, 5 out]
            n593 = property on="移动" class="Bool (strict)"() -> ("Value"=w1048:bool)  [unwired: 2 in, 2 out]
            n594 = Not(x=w1048) -> (.not. x?=w1047:bool)
            n595 = And(x=w1047, y=w1045) -> (x .and. y?=w1046:bool)
            n596 = case shown="True" w1046 {
              frame False {
              }
              frame True {
                n597 = property on="A1-position-X" class="DigNum (strict)"() -> (error out=w1054:errorcluster, "Value"=w1061:dbl)  [unwired: 2 in, 1 out]
                n598 = property on="A1-position-Y" class="DigNum (strict)"(error in=w1054) -> (error out=w1053:errorcluster, "Value"=w1050:dbl)  [unwired: 1 in, 1 out]
                n599 = Subtract(x=w1050, y=4.5) -> (x-y=w1049:dbl)
                n600 = Subtract(x=w1061, y=9) -> (x-y=w1052:dbl)
                n601 = vi-ref "goto.vi"() -> (w1059:refnum<vi>)
                n602 = property class="VI"(reference=w1059, error in=w1053) -> ("Name"=w1058:string)  [unwired: 2 out]
                n603 = Open VI Reference(type specifier VI Refnum (for type only)=refnum<vi> refnum, vi path=w1058, options=128) -> (vi reference=w1056:refnum<vi>)  [unwired: 3 in, 1 out]
                n604 = call-by-ref "Start Asynchronous Call"(reference=w1056, "Y(mm)"=w1049, "X(mm)"=w1052) -> ()  [unwired: 10 in, 3 out]
              }
            }
            n605 = property on="currentNO" class="Str"("Value"="B3") -> ()  [unwired: 2 in, 2 out]
          }
          event "B4": Value Change {
            n606 = event-data() -> ("NewVal"=w1064:bool)  [unwired: 1 in, 5 out]
            n607 = property on="移动" class="Bool (strict)"() -> ("Value"=w1067:bool)  [unwired: 2 in, 2 out]
            n608 = Not(x=w1067) -> (.not. x?=w1066:bool)
            n609 = And(x=w1066, y=w1064) -> (x .and. y?=w1065:bool)
            n610 = case shown="True" w1065 {
              frame False {
              }
              frame True {
                n611 = property on="A1-position-X" class="DigNum (strict)"() -> (error out=w1073:errorcluster, "Value"=w1080:dbl)  [unwired: 2 in, 1 out]
                n612 = property on="A1-position-Y" class="DigNum (strict)"(error in=w1073) -> (error out=w1072:errorcluster, "Value"=w1069:dbl)  [unwired: 1 in, 1 out]
                n613 = Subtract(x=w1069, y=4.5) -> (x-y=w1068:dbl)
                n614 = Subtract(x=w1080, y=13.5) -> (x-y=w1071:dbl)
                n615 = vi-ref "goto.vi"() -> (w1078:refnum<vi>)
                n616 = property class="VI"(reference=w1078, error in=w1072) -> ("Name"=w1077:string)  [unwired: 2 out]
                n617 = Open VI Reference(type specifier VI Refnum (for type only)=refnum<vi> refnum, vi path=w1077, options=128) -> (vi reference=w1075:refnum<vi>)  [unwired: 3 in, 1 out]
                n618 = call-by-ref "Start Asynchronous Call"(reference=w1075, "Y(mm)"=w1068, "X(mm)"=w1071) -> ()  [unwired: 10 in, 3 out]
              }
            }
            n619 = property on="currentNO" class="Str"("Value"="B4") -> ()  [unwired: 2 in, 2 out]
          }
          event "B5": Value Change {
            n620 = event-data() -> ("NewVal"=w1083:bool)  [unwired: 1 in, 5 out]
            n621 = property on="移动" class="Bool (strict)"() -> ("Value"=w1086:bool)  [unwired: 2 in, 2 out]
            n622 = Not(x=w1086) -> (.not. x?=w1085:bool)
            n623 = And(x=w1085, y=w1083) -> (x .and. y?=w1084:bool)
            n624 = case shown="True" w1084 {
              frame False {
              }
              frame True {
                n625 = property on="A1-position-X" class="DigNum (strict)"() -> (error out=w1092:errorcluster, "Value"=w1099:dbl)  [unwired: 2 in, 1 out]
                n626 = property on="A1-position-Y" class="DigNum (strict)"(error in=w1092) -> (error out=w1091:errorcluster, "Value"=w1088:dbl)  [unwired: 1 in, 1 out]
                n627 = Subtract(x=w1088, y=4.5) -> (x-y=w1087:dbl)
                n628 = Subtract(x=w1099, y=18) -> (x-y=w1090:dbl)
                n629 = vi-ref "goto.vi"() -> (w1097:refnum<vi>)
                n630 = property class="VI"(reference=w1097, error in=w1091) -> ("Name"=w1096:string)  [unwired: 2 out]
                n631 = Open VI Reference(type specifier VI Refnum (for type only)=refnum<vi> refnum, vi path=w1096, options=128) -> (vi reference=w1094:refnum<vi>)  [unwired: 3 in, 1 out]
                n632 = call-by-ref "Start Asynchronous Call"(reference=w1094, "Y(mm)"=w1087, "X(mm)"=w1090) -> ()  [unwired: 10 in, 3 out]
              }
            }
            n633 = property on="currentNO" class="Str"("Value"="B5") -> ()  [unwired: 2 in, 2 out]
          }
          event "B6": Value Change {
            n634 = event-data() -> ("NewVal"=w1102:bool)  [unwired: 1 in, 5 out]
            n635 = property on="移动" class="Bool (strict)"() -> ("Value"=w1105:bool)  [unwired: 2 in, 2 out]
            n636 = Not(x=w1105) -> (.not. x?=w1104:bool)
            n637 = And(x=w1104, y=w1102) -> (x .and. y?=w1103:bool)
            n638 = case shown="True" w1103 {
              frame False {
              }
              frame True {
                n639 = property on="A1-position-X" class="DigNum (strict)"() -> (error out=w1111:errorcluster, "Value"=w1118:dbl)  [unwired: 2 in, 1 out]
                n640 = property on="A1-position-Y" class="DigNum (strict)"(error in=w1111) -> (error out=w1110:errorcluster, "Value"=w1107:dbl)  [unwired: 1 in, 1 out]
                n641 = Subtract(x=w1107, y=4.5) -> (x-y=w1106:dbl)
                n642 = Subtract(x=w1118, y=22.5) -> (x-y=w1109:dbl)
                n643 = vi-ref "goto.vi"() -> (w1116:refnum<vi>)
                n644 = property class="VI"(reference=w1116, error in=w1110) -> ("Name"=w1115:string)  [unwired: 2 out]
                n645 = Open VI Reference(type specifier VI Refnum (for type only)=refnum<vi> refnum, vi path=w1115, options=128) -> (vi reference=w1113:refnum<vi>)  [unwired: 3 in, 1 out]
                n646 = call-by-ref "Start Asynchronous Call"(reference=w1113, "Y(mm)"=w1106, "X(mm)"=w1109) -> ()  [unwired: 10 in, 3 out]
              }
            }
            n647 = property on="currentNO" class="Str"("Value"="B6") -> ()  [unwired: 2 in, 2 out]
          }
          event "B7": Value Change {
            n648 = event-data() -> ("NewVal"=w1121:bool)  [unwired: 1 in, 5 out]
            n649 = property on="移动" class="Bool (strict)"() -> ("Value"=w1124:bool)  [unwired: 2 in, 2 out]
            n650 = Not(x=w1124) -> (.not. x?=w1123:bool)
            n651 = And(x=w1123, y=w1121) -> (x .and. y?=w1122:bool)
            n652 = case shown="True" w1122 {
              frame False {
              }
              frame True {
                n653 = property on="A1-position-X" class="DigNum (strict)"() -> (error out=w1130:errorcluster, "Value"=w1137:dbl)  [unwired: 2 in, 1 out]
                n654 = property on="A1-position-Y" class="DigNum (strict)"(error in=w1130) -> (error out=w1129:errorcluster, "Value"=w1126:dbl)  [unwired: 1 in, 1 out]
                n655 = Subtract(x=w1126, y=4.5) -> (x-y=w1125:dbl)
                n656 = Subtract(x=w1137, y=27) -> (x-y=w1128:dbl)
                n657 = vi-ref "goto.vi"() -> (w1135:refnum<vi>)
                n658 = property class="VI"(reference=w1135, error in=w1129) -> ("Name"=w1134:string)  [unwired: 2 out]
                n659 = Open VI Reference(type specifier VI Refnum (for type only)=refnum<vi> refnum, vi path=w1134, options=128) -> (vi reference=w1132:refnum<vi>)  [unwired: 3 in, 1 out]
                n660 = call-by-ref "Start Asynchronous Call"(reference=w1132, "Y(mm)"=w1125, "X(mm)"=w1128) -> ()  [unwired: 10 in, 3 out]
              }
            }
            n661 = property on="currentNO" class="Str"("Value"="B7") -> ()  [unwired: 2 in, 2 out]
          }
          event "B8": Value Change {
            n662 = event-data() -> ("NewVal"=w1140:bool)  [unwired: 1 in, 5 out]
            n663 = property on="移动" class="Bool (strict)"() -> ("Value"=w1143:bool)  [unwired: 2 in, 2 out]
            n664 = Not(x=w1143) -> (.not. x?=w1142:bool)
            n665 = And(x=w1142, y=w1140) -> (x .and. y?=w1141:bool)
            n666 = case shown="True" w1141 {
              frame False {
              }
              frame True {
                n667 = property on="A1-position-X" class="DigNum (strict)"() -> (error out=w1149:errorcluster, "Value"=w1156:dbl)  [unwired: 2 in, 1 out]
                n668 = property on="A1-position-Y" class="DigNum (strict)"(error in=w1149) -> (error out=w1148:errorcluster, "Value"=w1145:dbl)  [unwired: 1 in, 1 out]
                n669 = Subtract(x=w1145, y=4.5) -> (x-y=w1144:dbl)
                n670 = Subtract(x=w1156, y=31.5) -> (x-y=w1147:dbl)
                n671 = vi-ref "goto.vi"() -> (w1154:refnum<vi>)
                n672 = property class="VI"(reference=w1154, error in=w1148) -> ("Name"=w1153:string)  [unwired: 2 out]
                n673 = Open VI Reference(type specifier VI Refnum (for type only)=refnum<vi> refnum, vi path=w1153, options=128) -> (vi reference=w1151:refnum<vi>)  [unwired: 3 in, 1 out]
                n674 = call-by-ref "Start Asynchronous Call"(reference=w1151, "Y(mm)"=w1144, "X(mm)"=w1147) -> ()  [unwired: 10 in, 3 out]
              }
            }
            n675 = property on="currentNO" class="Str"("Value"="B8") -> ()  [unwired: 2 in, 2 out]
          }
          event "B9": Value Change {
            n676 = event-data() -> ("NewVal"=w1159:bool)  [unwired: 1 in, 5 out]
            n677 = property on="移动" class="Bool (strict)"() -> ("Value"=w1162:bool)  [unwired: 2 in, 2 out]
            n678 = Not(x=w1162) -> (.not. x?=w1161:bool)
            n679 = And(x=w1161, y=w1159) -> (x .and. y?=w1160:bool)
            n680 = case shown="True" w1160 {
              frame False {
              }
              frame True {
                n681 = property on="A1-position-X" class="DigNum (strict)"() -> (error out=w1168:errorcluster, "Value"=w1175:dbl)  [unwired: 2 in, 1 out]
                n682 = property on="A1-position-Y" class="DigNum (strict)"(error in=w1168) -> (error out=w1167:errorcluster, "Value"=w1164:dbl)  [unwired: 1 in, 1 out]
                n683 = Subtract(x=w1164, y=4.5) -> (x-y=w1163:dbl)
                n684 = Subtract(x=w1175, y=36) -> (x-y=w1166:dbl)
                n685 = vi-ref "goto.vi"() -> (w1173:refnum<vi>)
                n686 = property class="VI"(reference=w1173, error in=w1167) -> ("Name"=w1172:string)  [unwired: 2 out]
                n687 = Open VI Reference(type specifier VI Refnum (for type only)=refnum<vi> refnum, vi path=w1172, options=128) -> (vi reference=w1170:refnum<vi>)  [unwired: 3 in, 1 out]
                n688 = call-by-ref "Start Asynchronous Call"(reference=w1170, "Y(mm)"=w1163, "X(mm)"=w1166) -> ()  [unwired: 10 in, 3 out]
              }
            }
            n689 = property on="currentNO" class="Str"("Value"="B9") -> ()  [unwired: 2 in, 2 out]
          }
          event "B10": Value Change {
            n690 = event-data() -> ("NewVal"=w1178:bool)  [unwired: 1 in, 5 out]
            n691 = property on="移动" class="Bool (strict)"() -> ("Value"=w1181:bool)  [unwired: 2 in, 2 out]
            n692 = Not(x=w1181) -> (.not. x?=w1180:bool)
            n693 = And(x=w1180, y=w1178) -> (x .and. y?=w1179:bool)
            n694 = case shown="True" w1179 {
              frame False {
              }
              frame True {
                n695 = property on="A1-position-X" class="DigNum (strict)"() -> (error out=w1187:errorcluster, "Value"=w1194:dbl)  [unwired: 2 in, 1 out]
                n696 = property on="A1-position-Y" class="DigNum (strict)"(error in=w1187) -> (error out=w1186:errorcluster, "Value"=w1183:dbl)  [unwired: 1 in, 1 out]
                n697 = Subtract(x=w1183, y=4.5) -> (x-y=w1182:dbl)
                n698 = Subtract(x=w1194, y=40.5) -> (x-y=w1185:dbl)
                n699 = vi-ref "goto.vi"() -> (w1192:refnum<vi>)
                n700 = property class="VI"(reference=w1192, error in=w1186) -> ("Name"=w1191:string)  [unwired: 2 out]
                n701 = Open VI Reference(type specifier VI Refnum (for type only)=refnum<vi> refnum, vi path=w1191, options=128) -> (vi reference=w1189:refnum<vi>)  [unwired: 3 in, 1 out]
                n702 = call-by-ref "Start Asynchronous Call"(reference=w1189, "Y(mm)"=w1182, "X(mm)"=w1185) -> ()  [unwired: 10 in, 3 out]
              }
            }
            n703 = property on="currentNO" class="Str"("Value"="B10") -> ()  [unwired: 2 in, 2 out]
          }
          event "B11": Value Change {
            n704 = event-data() -> ("NewVal"=w1197:bool)  [unwired: 1 in, 5 out]
            n705 = property on="移动" class="Bool (strict)"() -> ("Value"=w1200:bool)  [unwired: 2 in, 2 out]
            n706 = Not(x=w1200) -> (.not. x?=w1199:bool)
            n707 = And(x=w1199, y=w1197) -> (x .and. y?=w1198:bool)
            n708 = case shown="True" w1198 {
              frame False {
              }
              frame True {
                n709 = property on="A1-position-X" class="DigNum (strict)"() -> (error out=w1206:errorcluster, "Value"=w1213:dbl)  [unwired: 2 in, 1 out]
                n710 = property on="A1-position-Y" class="DigNum (strict)"(error in=w1206) -> (error out=w1205:errorcluster, "Value"=w1202:dbl)  [unwired: 1 in, 1 out]
                n711 = Subtract(x=w1202, y=4.5) -> (x-y=w1201:dbl)
                n712 = Subtract(x=w1213, y=45) -> (x-y=w1204:dbl)
                n713 = vi-ref "goto.vi"() -> (w1211:refnum<vi>)
                n714 = property class="VI"(reference=w1211, error in=w1205) -> ("Name"=w1210:string)  [unwired: 2 out]
                n715 = Open VI Reference(type specifier VI Refnum (for type only)=refnum<vi> refnum, vi path=w1210, options=128) -> (vi reference=w1208:refnum<vi>)  [unwired: 3 in, 1 out]
                n716 = call-by-ref "Start Asynchronous Call"(reference=w1208, "Y(mm)"=w1201, "X(mm)"=w1204) -> ()  [unwired: 10 in, 3 out]
              }
            }
            n717 = property on="currentNO" class="Str"("Value"="B11") -> ()  [unwired: 2 in, 2 out]
          }
          event "B12": Value Change {
            n718 = event-data() -> ("NewVal"=w1216:bool)  [unwired: 1 in, 5 out]
            n719 = property on="移动" class="Bool (strict)"() -> ("Value"=w1219:bool)  [unwired: 2 in, 2 out]
            n720 = Not(x=w1219) -> (.not. x?=w1218:bool)
            n721 = And(x=w1218, y=w1216) -> (x .and. y?=w1217:bool)
            n722 = case shown="True" w1217 {
              frame False {
              }
              frame True {
                n723 = property on="A1-position-X" class="DigNum (strict)"() -> (error out=w1225:errorcluster, "Value"=w1232:dbl)  [unwired: 2 in, 1 out]
                n724 = property on="A1-position-Y" class="DigNum (strict)"(error in=w1225) -> (error out=w1224:errorcluster, "Value"=w1221:dbl)  [unwired: 1 in, 1 out]
                n725 = Subtract(x=w1221, y=4.5) -> (x-y=w1220:dbl)
                n726 = Subtract(x=w1232, y=49.5) -> (x-y=w1223:dbl)
                n727 = vi-ref "goto.vi"() -> (w1230:refnum<vi>)
                n728 = property class="VI"(reference=w1230, error in=w1224) -> ("Name"=w1229:string)  [unwired: 2 out]
                n729 = Open VI Reference(type specifier VI Refnum (for type only)=refnum<vi> refnum, vi path=w1229, options=128) -> (vi reference=w1227:refnum<vi>)  [unwired: 3 in, 1 out]
                n730 = call-by-ref "Start Asynchronous Call"(reference=w1227, "Y(mm)"=w1220, "X(mm)"=w1223) -> ()  [unwired: 10 in, 3 out]
              }
            }
            n731 = property on="currentNO" class="Str"("Value"="B12") -> ()  [unwired: 2 in, 2 out]
          }
          event "C1": Value Change {
            n732 = event-data() -> ("NewVal"=w1235:bool)  [unwired: 1 in, 5 out]
            n733 = property on="移动" class="Bool (strict)"() -> ("Value"=w1238:bool)  [unwired: 2 in, 2 out]
            n734 = Not(x=w1238) -> (.not. x?=w1237:bool)
            n735 = And(x=w1237, y=w1235) -> (x .and. y?=w1236:bool)
            n736 = case shown="True" w1236 {
              frame False {
              }
              frame True {
                n737 = property on="A1-position-X" class="DigNum (strict)"() -> (error out=w1244:errorcluster, "Value"=w1251:dbl)  [unwired: 2 in, 1 out]
                n738 = property on="A1-position-Y" class="DigNum (strict)"(error in=w1244) -> (error out=w1243:errorcluster, "Value"=w1240:dbl)  [unwired: 1 in, 1 out]
                n739 = Subtract(x=w1240, y=9) -> (x-y=w1239:dbl)
                n740 = Subtract(x=w1251, y=0) -> (x-y=w1242:dbl)
                n741 = vi-ref "goto.vi"() -> (w1249:refnum<vi>)
                n742 = property class="VI"(reference=w1249, error in=w1243) -> ("Name"=w1248:string)  [unwired: 2 out]
                n743 = Open VI Reference(type specifier VI Refnum (for type only)=refnum<vi> refnum, vi path=w1248, options=128) -> (vi reference=w1246:refnum<vi>)  [unwired: 3 in, 1 out]
                n744 = call-by-ref "Start Asynchronous Call"(reference=w1246, "Y(mm)"=w1239, "X(mm)"=w1242) -> ()  [unwired: 10 in, 3 out]
              }
            }
            n745 = property on="currentNO" class="Str"("Value"="C1") -> ()  [unwired: 2 in, 2 out]
          }
          event "C2": Value Change {
            n746 = event-data() -> ("NewVal"=w1254:bool)  [unwired: 1 in, 5 out]
            n747 = property on="移动" class="Bool (strict)"() -> ("Value"=w1257:bool)  [unwired: 2 in, 2 out]
            n748 = Not(x=w1257) -> (.not. x?=w1256:bool)
            n749 = And(x=w1256, y=w1254) -> (x .and. y?=w1255:bool)
            n750 = case shown="True" w1255 {
              frame False {
              }
              frame True {
                n751 = property on="A1-position-X" class="DigNum (strict)"() -> (error out=w1263:errorcluster, "Value"=w1270:dbl)  [unwired: 2 in, 1 out]
                n752 = property on="A1-position-Y" class="DigNum (strict)"(error in=w1263) -> (error out=w1262:errorcluster, "Value"=w1259:dbl)  [unwired: 1 in, 1 out]
                n753 = Subtract(x=w1259, y=9) -> (x-y=w1258:dbl)
                n754 = Subtract(x=w1270, y=4.5) -> (x-y=w1261:dbl)
                n755 = vi-ref "goto.vi"() -> (w1268:refnum<vi>)
                n756 = property class="VI"(reference=w1268, error in=w1262) -> ("Name"=w1267:string)  [unwired: 2 out]
                n757 = Open VI Reference(type specifier VI Refnum (for type only)=refnum<vi> refnum, vi path=w1267, options=128) -> (vi reference=w1265:refnum<vi>)  [unwired: 3 in, 1 out]
                n758 = call-by-ref "Start Asynchronous Call"(reference=w1265, "Y(mm)"=w1258, "X(mm)"=w1261) -> ()  [unwired: 10 in, 3 out]
              }
            }
            n759 = property on="currentNO" class="Str"("Value"="C2") -> ()  [unwired: 2 in, 2 out]
          }
          event "C3": Value Change {
            n760 = event-data() -> ("NewVal"=w1273:bool)  [unwired: 1 in, 5 out]
            n761 = property on="移动" class="Bool (strict)"() -> ("Value"=w1276:bool)  [unwired: 2 in, 2 out]
            n762 = Not(x=w1276) -> (.not. x?=w1275:bool)
            n763 = And(x=w1275, y=w1273) -> (x .and. y?=w1274:bool)
            n764 = case shown="True" w1274 {
              frame False {
              }
              frame True {
                n765 = property on="A1-position-X" class="DigNum (strict)"() -> (error out=w1282:errorcluster, "Value"=w1289:dbl)  [unwired: 2 in, 1 out]
                n766 = property on="A1-position-Y" class="DigNum (strict)"(error in=w1282) -> (error out=w1281:errorcluster, "Value"=w1278:dbl)  [unwired: 1 in, 1 out]
                n767 = Subtract(x=w1278, y=9) -> (x-y=w1277:dbl)
                n768 = Subtract(x=w1289, y=9) -> (x-y=w1280:dbl)
                n769 = vi-ref "goto.vi"() -> (w1287:refnum<vi>)
                n770 = property class="VI"(reference=w1287, error in=w1281) -> ("Name"=w1286:string)  [unwired: 2 out]
                n771 = Open VI Reference(type specifier VI Refnum (for type only)=refnum<vi> refnum, vi path=w1286, options=128) -> (vi reference=w1284:refnum<vi>)  [unwired: 3 in, 1 out]
                n772 = call-by-ref "Start Asynchronous Call"(reference=w1284, "Y(mm)"=w1277, "X(mm)"=w1280) -> ()  [unwired: 10 in, 3 out]
              }
            }
            n773 = property on="currentNO" class="Str"("Value"="C3") -> ()  [unwired: 2 in, 2 out]
          }
          event "C4": Value Change {
            n774 = event-data() -> ("NewVal"=w1292:bool)  [unwired: 1 in, 5 out]
            n775 = property on="移动" class="Bool (strict)"() -> ("Value"=w1295:bool)  [unwired: 2 in, 2 out]
            n776 = Not(x=w1295) -> (.not. x?=w1294:bool)
            n777 = And(x=w1294, y=w1292) -> (x .and. y?=w1293:bool)
            n778 = case shown="True" w1293 {
              frame False {
              }
              frame True {
                n779 = property on="A1-position-X" class="DigNum (strict)"() -> (error out=w1301:errorcluster, "Value"=w1308:dbl)  [unwired: 2 in, 1 out]
                n780 = property on="A1-position-Y" class="DigNum (strict)"(error in=w1301) -> (error out=w1300:errorcluster, "Value"=w1297:dbl)  [unwired: 1 in, 1 out]
                n781 = Subtract(x=w1297, y=9) -> (x-y=w1296:dbl)
                n782 = Subtract(x=w1308, y=13.5) -> (x-y=w1299:dbl)
                n783 = vi-ref "goto.vi"() -> (w1306:refnum<vi>)
                n784 = property class="VI"(reference=w1306, error in=w1300) -> ("Name"=w1305:string)  [unwired: 2 out]
                n785 = Open VI Reference(type specifier VI Refnum (for type only)=refnum<vi> refnum, vi path=w1305, options=128) -> (vi reference=w1303:refnum<vi>)  [unwired: 3 in, 1 out]
                n786 = call-by-ref "Start Asynchronous Call"(reference=w1303, "Y(mm)"=w1296, "X(mm)"=w1299) -> ()  [unwired: 10 in, 3 out]
              }
            }
            n787 = property on="currentNO" class="Str"("Value"="C4") -> ()  [unwired: 2 in, 2 out]
          }
          event "C5": Value Change {
            n788 = event-data() -> ("NewVal"=w1311:bool)  [unwired: 1 in, 5 out]
            n789 = property on="移动" class="Bool (strict)"() -> ("Value"=w1314:bool)  [unwired: 2 in, 2 out]
            n790 = Not(x=w1314) -> (.not. x?=w1313:bool)
            n791 = And(x=w1313, y=w1311) -> (x .and. y?=w1312:bool)
            n792 = case shown="True" w1312 {
              frame False {
              }
              frame True {
                n793 = property on="A1-position-X" class="DigNum (strict)"() -> (error out=w1320:errorcluster, "Value"=w1327:dbl)  [unwired: 2 in, 1 out]
                n794 = property on="A1-position-Y" class="DigNum (strict)"(error in=w1320) -> (error out=w1319:errorcluster, "Value"=w1316:dbl)  [unwired: 1 in, 1 out]
                n795 = Subtract(x=w1316, y=9) -> (x-y=w1315:dbl)
                n796 = Subtract(x=w1327, y=18) -> (x-y=w1318:dbl)
                n797 = vi-ref "goto.vi"() -> (w1325:refnum<vi>)
                n798 = property class="VI"(reference=w1325, error in=w1319) -> ("Name"=w1324:string)  [unwired: 2 out]
                n799 = Open VI Reference(type specifier VI Refnum (for type only)=refnum<vi> refnum, vi path=w1324, options=128) -> (vi reference=w1322:refnum<vi>)  [unwired: 3 in, 1 out]
                n800 = call-by-ref "Start Asynchronous Call"(reference=w1322, "Y(mm)"=w1315, "X(mm)"=w1318) -> ()  [unwired: 10 in, 3 out]
              }
            }
            n801 = property on="currentNO" class="Str"("Value"="C5") -> ()  [unwired: 2 in, 2 out]
          }
          event "C6": Value Change {
            n802 = event-data() -> ("NewVal"=w1330:bool)  [unwired: 1 in, 5 out]
            n803 = property on="移动" class="Bool (strict)"() -> ("Value"=w1333:bool)  [unwired: 2 in, 2 out]
            n804 = Not(x=w1333) -> (.not. x?=w1332:bool)
            n805 = And(x=w1332, y=w1330) -> (x .and. y?=w1331:bool)
            n806 = case shown="True" w1331 {
              frame False {
              }
              frame True {
                n807 = property on="A1-position-X" class="DigNum (strict)"() -> (error out=w1339:errorcluster, "Value"=w1346:dbl)  [unwired: 2 in, 1 out]
                n808 = property on="A1-position-Y" class="DigNum (strict)"(error in=w1339) -> (error out=w1338:errorcluster, "Value"=w1335:dbl)  [unwired: 1 in, 1 out]
                n809 = Subtract(x=w1335, y=9) -> (x-y=w1334:dbl)
                n810 = Subtract(x=w1346, y=22.5) -> (x-y=w1337:dbl)
                n811 = vi-ref "goto.vi"() -> (w1344:refnum<vi>)
                n812 = property class="VI"(reference=w1344, error in=w1338) -> ("Name"=w1343:string)  [unwired: 2 out]
                n813 = Open VI Reference(type specifier VI Refnum (for type only)=refnum<vi> refnum, vi path=w1343, options=128) -> (vi reference=w1341:refnum<vi>)  [unwired: 3 in, 1 out]
                n814 = call-by-ref "Start Asynchronous Call"(reference=w1341, "Y(mm)"=w1334, "X(mm)"=w1337) -> ()  [unwired: 10 in, 3 out]
              }
            }
            n815 = property on="currentNO" class="Str"("Value"="C6") -> ()  [unwired: 2 in, 2 out]
          }
          event "C7": Value Change {
            n816 = event-data() -> ("NewVal"=w1349:bool)  [unwired: 1 in, 5 out]
            n817 = property on="移动" class="Bool (strict)"() -> ("Value"=w1352:bool)  [unwired: 2 in, 2 out]
            n818 = Not(x=w1352) -> (.not. x?=w1351:bool)
            n819 = And(x=w1351, y=w1349) -> (x .and. y?=w1350:bool)
            n820 = case shown="True" w1350 {
              frame False {
              }
              frame True {
                n821 = property on="A1-position-X" class="DigNum (strict)"() -> (error out=w1358:errorcluster, "Value"=w1365:dbl)  [unwired: 2 in, 1 out]
                n822 = property on="A1-position-Y" class="DigNum (strict)"(error in=w1358) -> (error out=w1357:errorcluster, "Value"=w1354:dbl)  [unwired: 1 in, 1 out]
                n823 = Subtract(x=w1354, y=9) -> (x-y=w1353:dbl)
                n824 = Subtract(x=w1365, y=27) -> (x-y=w1356:dbl)
                n825 = vi-ref "goto.vi"() -> (w1363:refnum<vi>)
                n826 = property class="VI"(reference=w1363, error in=w1357) -> ("Name"=w1362:string)  [unwired: 2 out]
                n827 = Open VI Reference(type specifier VI Refnum (for type only)=refnum<vi> refnum, vi path=w1362, options=128) -> (vi reference=w1360:refnum<vi>)  [unwired: 3 in, 1 out]
                n828 = call-by-ref "Start Asynchronous Call"(reference=w1360, "Y(mm)"=w1353, "X(mm)"=w1356) -> ()  [unwired: 10 in, 3 out]
              }
            }
            n829 = property on="currentNO" class="Str"("Value"="C7") -> ()  [unwired: 2 in, 2 out]
          }
          event "C8": Value Change {
            n830 = event-data() -> ("NewVal"=w1368:bool)  [unwired: 1 in, 5 out]
            n831 = property on="移动" class="Bool (strict)"() -> ("Value"=w1371:bool)  [unwired: 2 in, 2 out]
            n832 = Not(x=w1371) -> (.not. x?=w1370:bool)
            n833 = And(x=w1370, y=w1368) -> (x .and. y?=w1369:bool)
            n834 = case shown="True" w1369 {
              frame False {
              }
              frame True {
                n835 = property on="A1-position-X" class="DigNum (strict)"() -> (error out=w1377:errorcluster, "Value"=w1384:dbl)  [unwired: 2 in, 1 out]
                n836 = property on="A1-position-Y" class="DigNum (strict)"(error in=w1377) -> (error out=w1376:errorcluster, "Value"=w1373:dbl)  [unwired: 1 in, 1 out]
                n837 = Subtract(x=w1373, y=9) -> (x-y=w1372:dbl)
                n838 = Subtract(x=w1384, y=31.5) -> (x-y=w1375:dbl)
                n839 = vi-ref "goto.vi"() -> (w1382:refnum<vi>)
                n840 = property class="VI"(reference=w1382, error in=w1376) -> ("Name"=w1381:string)  [unwired: 2 out]
                n841 = Open VI Reference(type specifier VI Refnum (for type only)=refnum<vi> refnum, vi path=w1381, options=128) -> (vi reference=w1379:refnum<vi>)  [unwired: 3 in, 1 out]
                n842 = call-by-ref "Start Asynchronous Call"(reference=w1379, "Y(mm)"=w1372, "X(mm)"=w1375) -> ()  [unwired: 10 in, 3 out]
              }
            }
            n843 = property on="currentNO" class="Str"("Value"="C8") -> ()  [unwired: 2 in, 2 out]
          }
          event "C9": Value Change {
            n844 = event-data() -> ("NewVal"=w1387:bool)  [unwired: 1 in, 5 out]
            n845 = property on="移动" class="Bool (strict)"() -> ("Value"=w1390:bool)  [unwired: 2 in, 2 out]
            n846 = Not(x=w1390) -> (.not. x?=w1389:bool)
            n847 = And(x=w1389, y=w1387) -> (x .and. y?=w1388:bool)
            n848 = case shown="True" w1388 {
              frame False {
              }
              frame True {
                n849 = property on="A1-position-X" class="DigNum (strict)"() -> (error out=w1396:errorcluster, "Value"=w1403:dbl)  [unwired: 2 in, 1 out]
                n850 = property on="A1-position-Y" class="DigNum (strict)"(error in=w1396) -> (error out=w1395:errorcluster, "Value"=w1392:dbl)  [unwired: 1 in, 1 out]
                n851 = Subtract(x=w1392, y=9) -> (x-y=w1391:dbl)
                n852 = Subtract(x=w1403, y=36) -> (x-y=w1394:dbl)
                n853 = vi-ref "goto.vi"() -> (w1401:refnum<vi>)
                n854 = property class="VI"(reference=w1401, error in=w1395) -> ("Name"=w1400:string)  [unwired: 2 out]
                n855 = Open VI Reference(type specifier VI Refnum (for type only)=refnum<vi> refnum, vi path=w1400, options=128) -> (vi reference=w1398:refnum<vi>)  [unwired: 3 in, 1 out]
                n856 = call-by-ref "Start Asynchronous Call"(reference=w1398, "Y(mm)"=w1391, "X(mm)"=w1394) -> ()  [unwired: 10 in, 3 out]
              }
            }
            n857 = property on="currentNO" class="Str"("Value"="C9") -> ()  [unwired: 2 in, 2 out]
          }
          event "C10": Value Change {
            n858 = event-data() -> ("NewVal"=w1406:bool)  [unwired: 1 in, 5 out]
            n859 = property on="移动" class="Bool (strict)"() -> ("Value"=w1409:bool)  [unwired: 2 in, 2 out]
            n860 = Not(x=w1409) -> (.not. x?=w1408:bool)
            n861 = And(x=w1408, y=w1406) -> (x .and. y?=w1407:bool)
            n862 = case shown="True" w1407 {
              frame False {
              }
              frame True {
                n863 = property on="A1-position-X" class="DigNum (strict)"() -> (error out=w1415:errorcluster, "Value"=w1422:dbl)  [unwired: 2 in, 1 out]
                n864 = property on="A1-position-Y" class="DigNum (strict)"(error in=w1415) -> (error out=w1414:errorcluster, "Value"=w1411:dbl)  [unwired: 1 in, 1 out]
                n865 = Subtract(x=w1411, y=9) -> (x-y=w1410:dbl)
                n866 = Subtract(x=w1422, y=40.5) -> (x-y=w1413:dbl)
                n867 = vi-ref "goto.vi"() -> (w1420:refnum<vi>)
                n868 = property class="VI"(reference=w1420, error in=w1414) -> ("Name"=w1419:string)  [unwired: 2 out]
                n869 = Open VI Reference(type specifier VI Refnum (for type only)=refnum<vi> refnum, vi path=w1419, options=128) -> (vi reference=w1417:refnum<vi>)  [unwired: 3 in, 1 out]
                n870 = call-by-ref "Start Asynchronous Call"(reference=w1417, "Y(mm)"=w1410, "X(mm)"=w1413) -> ()  [unwired: 10 in, 3 out]
              }
            }
            n871 = property on="currentNO" class="Str"("Value"="C10") -> ()  [unwired: 2 in, 2 out]
          }
          event "C11": Value Change {
            n872 = event-data() -> ("NewVal"=w1425:bool)  [unwired: 1 in, 5 out]
            n873 = property on="移动" class="Bool (strict)"() -> ("Value"=w1428:bool)  [unwired: 2 in, 2 out]
            n874 = Not(x=w1428) -> (.not. x?=w1427:bool)
            n875 = And(x=w1427, y=w1425) -> (x .and. y?=w1426:bool)
            n876 = case shown="True" w1426 {
              frame False {
              }
              frame True {
                n877 = property on="A1-position-X" class="DigNum (strict)"() -> (error out=w1434:errorcluster, "Value"=w1441:dbl)  [unwired: 2 in, 1 out]
                n878 = property on="A1-position-Y" class="DigNum (strict)"(error in=w1434) -> (error out=w1433:errorcluster, "Value"=w1430:dbl)  [unwired: 1 in, 1 out]
                n879 = Subtract(x=w1430, y=9) -> (x-y=w1429:dbl)
                n880 = Subtract(x=w1441, y=45) -> (x-y=w1432:dbl)
                n881 = vi-ref "goto.vi"() -> (w1439:refnum<vi>)
                n882 = property class="VI"(reference=w1439, error in=w1433) -> ("Name"=w1438:string)  [unwired: 2 out]
                n883 = Open VI Reference(type specifier VI Refnum (for type only)=refnum<vi> refnum, vi path=w1438, options=128) -> (vi reference=w1436:refnum<vi>)  [unwired: 3 in, 1 out]
                n884 = call-by-ref "Start Asynchronous Call"(reference=w1436, "Y(mm)"=w1429, "X(mm)"=w1432) -> ()  [unwired: 10 in, 3 out]
              }
            }
            n885 = property on="currentNO" class="Str"("Value"="C11") -> ()  [unwired: 2 in, 2 out]
          }
          event "C12": Value Change {
            n886 = event-data() -> ("NewVal"=w1444:bool)  [unwired: 1 in, 5 out]
            n887 = property on="移动" class="Bool (strict)"() -> ("Value"=w1447:bool)  [unwired: 2 in, 2 out]
            n888 = Not(x=w1447) -> (.not. x?=w1446:bool)
            n889 = And(x=w1446, y=w1444) -> (x .and. y?=w1445:bool)
            n890 = case shown="True" w1445 {
              frame False {
              }
              frame True {
                n891 = property on="A1-position-X" class="DigNum (strict)"() -> (error out=w1453:errorcluster, "Value"=w1460:dbl)  [unwired: 2 in, 1 out]
                n892 = property on="A1-position-Y" class="DigNum (strict)"(error in=w1453) -> (error out=w1452:errorcluster, "Value"=w1449:dbl)  [unwired: 1 in, 1 out]
                n893 = Subtract(x=w1449, y=9) -> (x-y=w1448:dbl)
                n894 = Subtract(x=w1460, y=49.5) -> (x-y=w1451:dbl)
                n895 = vi-ref "goto.vi"() -> (w1458:refnum<vi>)
                n896 = property class="VI"(reference=w1458, error in=w1452) -> ("Name"=w1457:string)  [unwired: 2 out]
                n897 = Open VI Reference(type specifier VI Refnum (for type only)=refnum<vi> refnum, vi path=w1457, options=128) -> (vi reference=w1455:refnum<vi>)  [unwired: 3 in, 1 out]
                n898 = call-by-ref "Start Asynchronous Call"(reference=w1455, "Y(mm)"=w1448, "X(mm)"=w1451) -> ()  [unwired: 10 in, 3 out]
              }
            }
            n899 = property on="currentNO" class="Str"("Value"="C12") -> ()  [unwired: 2 in, 2 out]
          }
          event "D1": Value Change {
            n900 = event-data() -> ("NewVal"=w1463:bool)  [unwired: 1 in, 5 out]
            n901 = property on="移动" class="Bool (strict)"() -> ("Value"=w1466:bool)  [unwired: 2 in, 2 out]
            n902 = Not(x=w1466) -> (.not. x?=w1465:bool)
            n903 = And(x=w1465, y=w1463) -> (x .and. y?=w1464:bool)
            n904 = case shown="True" w1464 {
              frame False {
              }
              frame True {
                n905 = property on="A1-position-X" class="DigNum (strict)"() -> (error out=w1472:errorcluster, "Value"=w1479:dbl)  [unwired: 2 in, 1 out]
                n906 = property on="A1-position-Y" class="DigNum (strict)"(error in=w1472) -> (error out=w1471:errorcluster, "Value"=w1468:dbl)  [unwired: 1 in, 1 out]
                n907 = Subtract(x=w1468, y=13.5) -> (x-y=w1467:dbl)
                n908 = Subtract(x=w1479, y=0) -> (x-y=w1470:dbl)
                n909 = vi-ref "goto.vi"() -> (w1477:refnum<vi>)
                n910 = property class="VI"(reference=w1477, error in=w1471) -> ("Name"=w1476:string)  [unwired: 2 out]
                n911 = Open VI Reference(type specifier VI Refnum (for type only)=refnum<vi> refnum, vi path=w1476, options=128) -> (vi reference=w1474:refnum<vi>)  [unwired: 3 in, 1 out]
                n912 = call-by-ref "Start Asynchronous Call"(reference=w1474, "Y(mm)"=w1467, "X(mm)"=w1470) -> ()  [unwired: 10 in, 3 out]
              }
            }
            n913 = property on="currentNO" class="Str"("Value"="D1") -> ()  [unwired: 2 in, 2 out]
          }
          event "D2": Value Change {
            n914 = event-data() -> ("NewVal"=w1482:bool)  [unwired: 1 in, 5 out]
            n915 = property on="移动" class="Bool (strict)"() -> ("Value"=w1485:bool)  [unwired: 2 in, 2 out]
            n916 = Not(x=w1485) -> (.not. x?=w1484:bool)
            n917 = And(x=w1484, y=w1482) -> (x .and. y?=w1483:bool)
            n918 = case shown="True" w1483 {
              frame False {
              }
              frame True {
                n919 = property on="A1-position-X" class="DigNum (strict)"() -> (error out=w1491:errorcluster, "Value"=w1498:dbl)  [unwired: 2 in, 1 out]
                n920 = property on="A1-position-Y" class="DigNum (strict)"(error in=w1491) -> (error out=w1490:errorcluster, "Value"=w1487:dbl)  [unwired: 1 in, 1 out]
                n921 = Subtract(x=w1487, y=13.5) -> (x-y=w1486:dbl)
                n922 = Subtract(x=w1498, y=4.5) -> (x-y=w1489:dbl)
                n923 = vi-ref "goto.vi"() -> (w1496:refnum<vi>)
                n924 = property class="VI"(reference=w1496, error in=w1490) -> ("Name"=w1495:string)  [unwired: 2 out]
                n925 = Open VI Reference(type specifier VI Refnum (for type only)=refnum<vi> refnum, vi path=w1495, options=128) -> (vi reference=w1493:refnum<vi>)  [unwired: 3 in, 1 out]
                n926 = call-by-ref "Start Asynchronous Call"(reference=w1493, "Y(mm)"=w1486, "X(mm)"=w1489) -> ()  [unwired: 10 in, 3 out]
              }
            }
            n927 = property on="currentNO" class="Str"("Value"="D2") -> ()  [unwired: 2 in, 2 out]
          }
          event "D3": Value Change {
            n928 = event-data() -> ("NewVal"=w1501:bool)  [unwired: 1 in, 5 out]
            n929 = property on="移动" class="Bool (strict)"() -> ("Value"=w1504:bool)  [unwired: 2 in, 2 out]
            n930 = Not(x=w1504) -> (.not. x?=w1503:bool)
            n931 = And(x=w1503, y=w1501) -> (x .and. y?=w1502:bool)
            n932 = case shown="True" w1502 {
              frame False {
              }
              frame True {
                n933 = property on="A1-position-X" class="DigNum (strict)"() -> (error out=w1510:errorcluster, "Value"=w1517:dbl)  [unwired: 2 in, 1 out]
                n934 = property on="A1-position-Y" class="DigNum (strict)"(error in=w1510) -> (error out=w1509:errorcluster, "Value"=w1506:dbl)  [unwired: 1 in, 1 out]
                n935 = Subtract(x=w1506, y=13.5) -> (x-y=w1505:dbl)
                n936 = Subtract(x=w1517, y=9) -> (x-y=w1508:dbl)
                n937 = vi-ref "goto.vi"() -> (w1515:refnum<vi>)
                n938 = property class="VI"(reference=w1515, error in=w1509) -> ("Name"=w1514:string)  [unwired: 2 out]
                n939 = Open VI Reference(type specifier VI Refnum (for type only)=refnum<vi> refnum, vi path=w1514, options=128) -> (vi reference=w1512:refnum<vi>)  [unwired: 3 in, 1 out]
                n940 = call-by-ref "Start Asynchronous Call"(reference=w1512, "Y(mm)"=w1505, "X(mm)"=w1508) -> ()  [unwired: 10 in, 3 out]
              }
            }
            n941 = property on="currentNO" class="Str"("Value"="D3") -> ()  [unwired: 2 in, 2 out]
          }
          event "D4": Value Change {
            n942 = event-data() -> ("NewVal"=w1520:bool)  [unwired: 1 in, 5 out]
            n943 = property on="移动" class="Bool (strict)"() -> ("Value"=w1523:bool)  [unwired: 2 in, 2 out]
            n944 = Not(x=w1523) -> (.not. x?=w1522:bool)
            n945 = And(x=w1522, y=w1520) -> (x .and. y?=w1521:bool)
            n946 = case shown="True" w1521 {
              frame False {
              }
              frame True {
                n947 = property on="A1-position-X" class="DigNum (strict)"() -> (error out=w1529:errorcluster, "Value"=w1536:dbl)  [unwired: 2 in, 1 out]
                n948 = property on="A1-position-Y" class="DigNum (strict)"(error in=w1529) -> (error out=w1528:errorcluster, "Value"=w1525:dbl)  [unwired: 1 in, 1 out]
                n949 = Subtract(x=w1525, y=13.5) -> (x-y=w1524:dbl)
                n950 = Subtract(x=w1536, y=13.5) -> (x-y=w1527:dbl)
                n951 = vi-ref "goto.vi"() -> (w1534:refnum<vi>)
                n952 = property class="VI"(reference=w1534, error in=w1528) -> ("Name"=w1533:string)  [unwired: 2 out]
                n953 = Open VI Reference(type specifier VI Refnum (for type only)=refnum<vi> refnum, vi path=w1533, options=128) -> (vi reference=w1531:refnum<vi>)  [unwired: 3 in, 1 out]
                n954 = call-by-ref "Start Asynchronous Call"(reference=w1531, "Y(mm)"=w1524, "X(mm)"=w1527) -> ()  [unwired: 10 in, 3 out]
              }
            }
            n955 = property on="currentNO" class="Str"("Value"="D4") -> ()  [unwired: 2 in, 2 out]
          }
          event "D5": Value Change {
            n956 = event-data() -> ("NewVal"=w1539:bool)  [unwired: 1 in, 5 out]
            n957 = property on="移动" class="Bool (strict)"() -> ("Value"=w1542:bool)  [unwired: 2 in, 2 out]
            n958 = Not(x=w1542) -> (.not. x?=w1541:bool)
            n959 = And(x=w1541, y=w1539) -> (x .and. y?=w1540:bool)
            n960 = case shown="True" w1540 {
              frame False {
              }
              frame True {
                n961 = property on="A1-position-X" class="DigNum (strict)"() -> (error out=w1548:errorcluster, "Value"=w1555:dbl)  [unwired: 2 in, 1 out]
                n962 = property on="A1-position-Y" class="DigNum (strict)"(error in=w1548) -> (error out=w1547:errorcluster, "Value"=w1544:dbl)  [unwired: 1 in, 1 out]
                n963 = Subtract(x=w1544, y=13.5) -> (x-y=w1543:dbl)
                n964 = Subtract(x=w1555, y=18) -> (x-y=w1546:dbl)
                n965 = vi-ref "goto.vi"() -> (w1553:refnum<vi>)
                n966 = property class="VI"(reference=w1553, error in=w1547) -> ("Name"=w1552:string)  [unwired: 2 out]
                n967 = Open VI Reference(type specifier VI Refnum (for type only)=refnum<vi> refnum, vi path=w1552, options=128) -> (vi reference=w1550:refnum<vi>)  [unwired: 3 in, 1 out]
                n968 = call-by-ref "Start Asynchronous Call"(reference=w1550, "Y(mm)"=w1543, "X(mm)"=w1546) -> ()  [unwired: 10 in, 3 out]
              }
            }
            n969 = property on="currentNO" class="Str"("Value"="D5") -> ()  [unwired: 2 in, 2 out]
          }
          event "D6": Value Change {
            n970 = event-data() -> ("NewVal"=w1558:bool)  [unwired: 1 in, 5 out]
            n971 = property on="移动" class="Bool (strict)"() -> ("Value"=w1561:bool)  [unwired: 2 in, 2 out]
            n972 = Not(x=w1561) -> (.not. x?=w1560:bool)
            n973 = And(x=w1560, y=w1558) -> (x .and. y?=w1559:bool)
            n974 = case shown="True" w1559 {
              frame False {
              }
              frame True {
                n975 = property on="A1-position-X" class="DigNum (strict)"() -> (error out=w1567:errorcluster, "Value"=w1574:dbl)  [unwired: 2 in, 1 out]
                n976 = property on="A1-position-Y" class="DigNum (strict)"(error in=w1567) -> (error out=w1566:errorcluster, "Value"=w1563:dbl)  [unwired: 1 in, 1 out]
                n977 = Subtract(x=w1563, y=13.5) -> (x-y=w1562:dbl)
                n978 = Subtract(x=w1574, y=22.5) -> (x-y=w1565:dbl)
                n979 = vi-ref "goto.vi"() -> (w1572:refnum<vi>)
                n980 = property class="VI"(reference=w1572, error in=w1566) -> ("Name"=w1571:string)  [unwired: 2 out]
                n981 = Open VI Reference(type specifier VI Refnum (for type only)=refnum<vi> refnum, vi path=w1571, options=128) -> (vi reference=w1569:refnum<vi>)  [unwired: 3 in, 1 out]
                n982 = call-by-ref "Start Asynchronous Call"(reference=w1569, "Y(mm)"=w1562, "X(mm)"=w1565) -> ()  [unwired: 10 in, 3 out]
              }
            }
            n983 = property on="currentNO" class="Str"("Value"="D6") -> ()  [unwired: 2 in, 2 out]
          }
          event "D7": Value Change {
            n984 = event-data() -> ("NewVal"=w1577:bool)  [unwired: 1 in, 5 out]
            n985 = property on="移动" class="Bool (strict)"() -> ("Value"=w1580:bool)  [unwired: 2 in, 2 out]
            n986 = Not(x=w1580) -> (.not. x?=w1579:bool)
            n987 = And(x=w1579, y=w1577) -> (x .and. y?=w1578:bool)
            n988 = case shown="True" w1578 {
              frame False {
              }
              frame True {
                n989 = property on="A1-position-X" class="DigNum (strict)"() -> (error out=w1586:errorcluster, "Value"=w1593:dbl)  [unwired: 2 in, 1 out]
                n990 = property on="A1-position-Y" class="DigNum (strict)"(error in=w1586) -> (error out=w1585:errorcluster, "Value"=w1582:dbl)  [unwired: 1 in, 1 out]
                n991 = Subtract(x=w1582, y=13.5) -> (x-y=w1581:dbl)
                n992 = Subtract(x=w1593, y=27) -> (x-y=w1584:dbl)
                n993 = vi-ref "goto.vi"() -> (w1591:refnum<vi>)
                n994 = property class="VI"(reference=w1591, error in=w1585) -> ("Name"=w1590:string)  [unwired: 2 out]
                n995 = Open VI Reference(type specifier VI Refnum (for type only)=refnum<vi> refnum, vi path=w1590, options=128) -> (vi reference=w1588:refnum<vi>)  [unwired: 3 in, 1 out]
                n996 = call-by-ref "Start Asynchronous Call"(reference=w1588, "Y(mm)"=w1581, "X(mm)"=w1584) -> ()  [unwired: 10 in, 3 out]
              }
            }
            n997 = property on="currentNO" class="Str"("Value"="D7") -> ()  [unwired: 2 in, 2 out]
          }
          event "D8": Value Change {
            n998 = event-data() -> ("NewVal"=w1595:bool)  [unwired: 1 in, 5 out]
            n999 = property on="移动" class="Bool (strict)"() -> ("Value"=w1598:bool)  [unwired: 2 in, 2 out]
            n1000 = Not(x=w1598) -> (.not. x?=w1597:bool)
            n1001 = And(x=w1597, y=w1595) -> (x .and. y?=w1596:bool)
            n1002 = case shown="True" w1596 {
              frame False {
              }
              frame True {
                n1003 = property on="A1-position-X" class="DigNum (strict)"() -> (error out=w1605:errorcluster, "Value"=w1612:dbl)  [unwired: 2 in, 1 out]
                n1004 = property on="A1-position-Y" class="DigNum (strict)"(error in=w1605) -> (error out=w1604:errorcluster, "Value"=w1601:dbl)  [unwired: 1 in, 1 out]
                n1005 = Subtract(x=w1601, y=13.5) -> (x-y=w1600:dbl)
                n1006 = Subtract(x=w1612, y=31.5) -> (x-y=w1603:dbl)
                n1007 = vi-ref "goto.vi"() -> (w1610:refnum<vi>)
                n1008 = property class="VI"(reference=w1610, error in=w1604) -> ("Name"=w1609:string)  [unwired: 2 out]
                n1009 = Open VI Reference(type specifier VI Refnum (for type only)=refnum<vi> refnum, vi path=w1609, options=128) -> (vi reference=w1607:refnum<vi>)  [unwired: 3 in, 1 out]
                n1010 = call-by-ref "Start Asynchronous Call"(reference=w1607, "Y(mm)"=w1600, "X(mm)"=w1603) -> ()  [unwired: 10 in, 3 out]
              }
            }
            n1011 = property on="currentNO" class="Str"("Value"="D8") -> ()  [unwired: 2 in, 2 out]
          }
          event "D9": Value Change {
            n1012 = event-data() -> ("NewVal"=w1614:bool)  [unwired: 1 in, 5 out]
            n1013 = property on="移动" class="Bool (strict)"() -> ("Value"=w1617:bool)  [unwired: 2 in, 2 out]
            n1014 = Not(x=w1617) -> (.not. x?=w1616:bool)
            n1015 = And(x=w1616, y=w1614) -> (x .and. y?=w1615:bool)
            n1016 = case shown="True" w1615 {
              frame False {
              }
              frame True {
                n1017 = property on="A1-position-X" class="DigNum (strict)"() -> (error out=w1624:errorcluster, "Value"=w1631:dbl)  [unwired: 2 in, 1 out]
                n1018 = property on="A1-position-Y" class="DigNum (strict)"(error in=w1624) -> (error out=w1623:errorcluster, "Value"=w1620:dbl)  [unwired: 1 in, 1 out]
                n1019 = Subtract(x=w1620, y=13.5) -> (x-y=w1619:dbl)
                n1020 = Subtract(x=w1631, y=36) -> (x-y=w1622:dbl)
                n1021 = vi-ref "goto.vi"() -> (w1629:refnum<vi>)
                n1022 = property class="VI"(reference=w1629, error in=w1623) -> ("Name"=w1628:string)  [unwired: 2 out]
                n1023 = Open VI Reference(type specifier VI Refnum (for type only)=refnum<vi> refnum, vi path=w1628, options=128) -> (vi reference=w1626:refnum<vi>)  [unwired: 3 in, 1 out]
                n1024 = call-by-ref "Start Asynchronous Call"(reference=w1626, "Y(mm)"=w1619, "X(mm)"=w1622) -> ()  [unwired: 10 in, 3 out]
              }
            }
            n1025 = property on="currentNO" class="Str"("Value"="D9") -> ()  [unwired: 2 in, 2 out]
          }
          event "D10": Value Change {
            n1026 = event-data() -> ("NewVal"=w1633:bool)  [unwired: 1 in, 5 out]
            n1027 = property on="移动" class="Bool (strict)"() -> ("Value"=w1636:bool)  [unwired: 2 in, 2 out]
            n1028 = Not(x=w1636) -> (.not. x?=w1635:bool)
            n1029 = And(x=w1635, y=w1633) -> (x .and. y?=w1634:bool)
            n1030 = case shown="True" w1634 {
              frame False {
              }
              frame True {
                n1031 = property on="A1-position-X" class="DigNum (strict)"() -> (error out=w1643:errorcluster, "Value"=w1650:dbl)  [unwired: 2 in, 1 out]
                n1032 = property on="A1-position-Y" class="DigNum (strict)"(error in=w1643) -> (error out=w1642:errorcluster, "Value"=w1639:dbl)  [unwired: 1 in, 1 out]
                n1033 = Subtract(x=w1639, y=13.5) -> (x-y=w1638:dbl)
                n1034 = Subtract(x=w1650, y=40.5) -> (x-y=w1641:dbl)
                n1035 = vi-ref "goto.vi"() -> (w1648:refnum<vi>)
                n1036 = property class="VI"(reference=w1648, error in=w1642) -> ("Name"=w1647:string)  [unwired: 2 out]
                n1037 = Open VI Reference(type specifier VI Refnum (for type only)=refnum<vi> refnum, vi path=w1647, options=128) -> (vi reference=w1645:refnum<vi>)  [unwired: 3 in, 1 out]
                n1038 = call-by-ref "Start Asynchronous Call"(reference=w1645, "Y(mm)"=w1638, "X(mm)"=w1641) -> ()  [unwired: 10 in, 3 out]
              }
            }
            n1039 = property on="currentNO" class="Str"("Value"="D10") -> ()  [unwired: 2 in, 2 out]
          }
          event "D11": Value Change {
            n1040 = event-data() -> ("NewVal"=w1652:bool)  [unwired: 1 in, 5 out]
            n1041 = property on="移动" class="Bool (strict)"() -> ("Value"=w1655:bool)  [unwired: 2 in, 2 out]
            n1042 = Not(x=w1655) -> (.not. x?=w1654:bool)
            n1043 = And(x=w1654, y=w1652) -> (x .and. y?=w1653:bool)
            n1044 = case shown="True" w1653 {
              frame False {
              }
              frame True {
                n1045 = property on="A1-position-X" class="DigNum (strict)"() -> (error out=w1662:errorcluster, "Value"=w1669:dbl)  [unwired: 2 in, 1 out]
                n1046 = property on="A1-position-Y" class="DigNum (strict)"(error in=w1662) -> (error out=w1661:errorcluster, "Value"=w1658:dbl)  [unwired: 1 in, 1 out]
                n1047 = Subtract(x=w1658, y=13.5) -> (x-y=w1657:dbl)
                n1048 = Subtract(x=w1669, y=45) -> (x-y=w1660:dbl)
                n1049 = vi-ref "goto.vi"() -> (w1667:refnum<vi>)
                n1050 = property class="VI"(reference=w1667, error in=w1661) -> ("Name"=w1666:string)  [unwired: 2 out]
                n1051 = Open VI Reference(type specifier VI Refnum (for type only)=refnum<vi> refnum, vi path=w1666, options=128) -> (vi reference=w1664:refnum<vi>)  [unwired: 3 in, 1 out]
                n1052 = call-by-ref "Start Asynchronous Call"(reference=w1664, "Y(mm)"=w1657, "X(mm)"=w1660) -> ()  [unwired: 10 in, 3 out]
              }
            }
            n1053 = property on="currentNO" class="Str"("Value"="D11") -> ()  [unwired: 2 in, 2 out]
          }
          event "D12": Value Change {
            n1054 = event-data() -> ("NewVal"=w1671:bool)  [unwired: 1 in, 5 out]
            n1055 = property on="移动" class="Bool (strict)"() -> ("Value"=w1674:bool)  [unwired: 2 in, 2 out]
            n1056 = Not(x=w1674) -> (.not. x?=w1673:bool)
            n1057 = And(x=w1673, y=w1671) -> (x .and. y?=w1672:bool)
            n1058 = case shown="True" w1672 {
              frame False {
              }
              frame True {
                n1059 = property on="A1-position-X" class="DigNum (strict)"() -> (error out=w1681:errorcluster, "Value"=w1688:dbl)  [unwired: 2 in, 1 out]
                n1060 = property on="A1-position-Y" class="DigNum (strict)"(error in=w1681) -> (error out=w1680:errorcluster, "Value"=w1677:dbl)  [unwired: 1 in, 1 out]
                n1061 = Subtract(x=w1677, y=13.5) -> (x-y=w1676:dbl)
                n1062 = Subtract(x=w1688, y=49.5) -> (x-y=w1679:dbl)
                n1063 = vi-ref "goto.vi"() -> (w1686:refnum<vi>)
                n1064 = property class="VI"(reference=w1686, error in=w1680) -> ("Name"=w1685:string)  [unwired: 2 out]
                n1065 = Open VI Reference(type specifier VI Refnum (for type only)=refnum<vi> refnum, vi path=w1685, options=128) -> (vi reference=w1683:refnum<vi>)  [unwired: 3 in, 1 out]
                n1066 = call-by-ref "Start Asynchronous Call"(reference=w1683, "Y(mm)"=w1676, "X(mm)"=w1679) -> ()  [unwired: 10 in, 3 out]
              }
            }
            n1067 = property on="currentNO" class="Str"("Value"="D12") -> ()  [unwired: 2 in, 2 out]
          }
          event "E1": Value Change {
            n1068 = event-data() -> ("NewVal"=w1690:bool)  [unwired: 1 in, 5 out]
            n1069 = property on="移动" class="Bool (strict)"() -> ("Value"=w1693:bool)  [unwired: 2 in, 2 out]
            n1070 = Not(x=w1693) -> (.not. x?=w1692:bool)
            n1071 = And(x=w1692, y=w1690) -> (x .and. y?=w1691:bool)
            n1072 = case shown="True" w1691 {
              frame False {
              }
              frame True {
                n1073 = property on="A1-position-X" class="DigNum (strict)"() -> (error out=w1700:errorcluster, "Value"=w1707:dbl)  [unwired: 2 in, 1 out]
                n1074 = property on="A1-position-Y" class="DigNum (strict)"(error in=w1700) -> (error out=w1699:errorcluster, "Value"=w1696:dbl)  [unwired: 1 in, 1 out]
                n1075 = Subtract(x=w1696, y=18.0) -> (x-y=w1695:dbl)
                n1076 = Subtract(x=w1707, y=0) -> (x-y=w1698:dbl)
                n1077 = vi-ref "goto.vi"() -> (w1705:refnum<vi>)
                n1078 = property class="VI"(reference=w1705, error in=w1699) -> ("Name"=w1704:string)  [unwired: 2 out]
                n1079 = Open VI Reference(type specifier VI Refnum (for type only)=refnum<vi> refnum, vi path=w1704, options=128) -> (vi reference=w1702:refnum<vi>)  [unwired: 3 in, 1 out]
                n1080 = call-by-ref "Start Asynchronous Call"(reference=w1702, "Y(mm)"=w1695, "X(mm)"=w1698) -> ()  [unwired: 10 in, 3 out]
              }
            }
            n1081 = property on="currentNO" class="Str"("Value"="E1") -> ()  [unwired: 2 in, 2 out]
          }
          event "E2": Value Change {
            n1082 = event-data() -> ("NewVal"=w1709:bool)  [unwired: 1 in, 5 out]
            n1083 = property on="移动" class="Bool (strict)"() -> ("Value"=w1712:bool)  [unwired: 2 in, 2 out]
            n1084 = Not(x=w1712) -> (.not. x?=w1711:bool)
            n1085 = And(x=w1711, y=w1709) -> (x .and. y?=w1710:bool)
            n1086 = case shown="True" w1710 {
              frame False {
              }
              frame True {
                n1087 = property on="A1-position-X" class="DigNum (strict)"() -> (error out=w1719:errorcluster, "Value"=w1726:dbl)  [unwired: 2 in, 1 out]
                n1088 = property on="A1-position-Y" class="DigNum (strict)"(error in=w1719) -> (error out=w1718:errorcluster, "Value"=w1715:dbl)  [unwired: 1 in, 1 out]
                n1089 = Subtract(x=w1715, y=18.0) -> (x-y=w1714:dbl)
                n1090 = Subtract(x=w1726, y=4.5) -> (x-y=w1717:dbl)
                n1091 = vi-ref "goto.vi"() -> (w1724:refnum<vi>)
                n1092 = property class="VI"(reference=w1724, error in=w1718) -> ("Name"=w1723:string)  [unwired: 2 out]
                n1093 = Open VI Reference(type specifier VI Refnum (for type only)=refnum<vi> refnum, vi path=w1723, options=128) -> (vi reference=w1721:refnum<vi>)  [unwired: 3 in, 1 out]
                n1094 = call-by-ref "Start Asynchronous Call"(reference=w1721, "Y(mm)"=w1714, "X(mm)"=w1717) -> ()  [unwired: 10 in, 3 out]
              }
            }
            n1095 = property on="currentNO" class="Str"("Value"="E2") -> ()  [unwired: 2 in, 2 out]
          }
          event "E3": Value Change {
            n1096 = event-data() -> ("NewVal"=w1728:bool)  [unwired: 1 in, 5 out]
            n1097 = property on="移动" class="Bool (strict)"() -> ("Value"=w1731:bool)  [unwired: 2 in, 2 out]
            n1098 = Not(x=w1731) -> (.not. x?=w1730:bool)
            n1099 = And(x=w1730, y=w1728) -> (x .and. y?=w1729:bool)
            n1100 = case shown="True" w1729 {
              frame False {
              }
              frame True {
                n1101 = property on="A1-position-X" class="DigNum (strict)"() -> (error out=w1738:errorcluster, "Value"=w1745:dbl)  [unwired: 2 in, 1 out]
                n1102 = property on="A1-position-Y" class="DigNum (strict)"(error in=w1738) -> (error out=w1737:errorcluster, "Value"=w1734:dbl)  [unwired: 1 in, 1 out]
                n1103 = Subtract(x=w1734, y=18.0) -> (x-y=w1733:dbl)
                n1104 = Subtract(x=w1745, y=9) -> (x-y=w1736:dbl)
                n1105 = vi-ref "goto.vi"() -> (w1743:refnum<vi>)
                n1106 = property class="VI"(reference=w1743, error in=w1737) -> ("Name"=w1742:string)  [unwired: 2 out]
                n1107 = Open VI Reference(type specifier VI Refnum (for type only)=refnum<vi> refnum, vi path=w1742, options=128) -> (vi reference=w1740:refnum<vi>)  [unwired: 3 in, 1 out]
                n1108 = call-by-ref "Start Asynchronous Call"(reference=w1740, "Y(mm)"=w1733, "X(mm)"=w1736) -> ()  [unwired: 10 in, 3 out]
              }
            }
            n1109 = property on="currentNO" class="Str"("Value"="E3") -> ()  [unwired: 2 in, 2 out]
          }
          event "E4": Value Change {
            n1110 = event-data() -> ("NewVal"=w1747:bool)  [unwired: 1 in, 5 out]
            n1111 = property on="移动" class="Bool (strict)"() -> ("Value"=w1750:bool)  [unwired: 2 in, 2 out]
            n1112 = Not(x=w1750) -> (.not. x?=w1749:bool)
            n1113 = And(x=w1749, y=w1747) -> (x .and. y?=w1748:bool)
            n1114 = case shown="True" w1748 {
              frame False {
              }
              frame True {
                n1115 = property on="A1-position-X" class="DigNum (strict)"() -> (error out=w1757:errorcluster, "Value"=w1764:dbl)  [unwired: 2 in, 1 out]
                n1116 = property on="A1-position-Y" class="DigNum (strict)"(error in=w1757) -> (error out=w1756:errorcluster, "Value"=w1753:dbl)  [unwired: 1 in, 1 out]
                n1117 = Subtract(x=w1753, y=18.0) -> (x-y=w1752:dbl)
                n1118 = Subtract(x=w1764, y=13.5) -> (x-y=w1755:dbl)
                n1119 = vi-ref "goto.vi"() -> (w1762:refnum<vi>)
                n1120 = property class="VI"(reference=w1762, error in=w1756) -> ("Name"=w1761:string)  [unwired: 2 out]
                n1121 = Open VI Reference(type specifier VI Refnum (for type only)=refnum<vi> refnum, vi path=w1761, options=128) -> (vi reference=w1759:refnum<vi>)  [unwired: 3 in, 1 out]
                n1122 = call-by-ref "Start Asynchronous Call"(reference=w1759, "Y(mm)"=w1752, "X(mm)"=w1755) -> ()  [unwired: 10 in, 3 out]
              }
            }
            n1123 = property on="currentNO" class="Str"("Value"="E4") -> ()  [unwired: 2 in, 2 out]
          }
          event "E5": Value Change {
            n1124 = event-data() -> ("NewVal"=w1766:bool)  [unwired: 1 in, 5 out]
            n1125 = property on="移动" class="Bool (strict)"() -> ("Value"=w1769:bool)  [unwired: 2 in, 2 out]
            n1126 = Not(x=w1769) -> (.not. x?=w1768:bool)
            n1127 = And(x=w1768, y=w1766) -> (x .and. y?=w1767:bool)
            n1128 = case shown="True" w1767 {
              frame False {
              }
              frame True {
                n1129 = property on="A1-position-X" class="DigNum (strict)"() -> (error out=w1776:errorcluster, "Value"=w1783:dbl)  [unwired: 2 in, 1 out]
                n1130 = property on="A1-position-Y" class="DigNum (strict)"(error in=w1776) -> (error out=w1775:errorcluster, "Value"=w1772:dbl)  [unwired: 1 in, 1 out]
                n1131 = Subtract(x=w1772, y=18.0) -> (x-y=w1771:dbl)
                n1132 = Subtract(x=w1783, y=18) -> (x-y=w1774:dbl)
                n1133 = vi-ref "goto.vi"() -> (w1781:refnum<vi>)
                n1134 = property class="VI"(reference=w1781, error in=w1775) -> ("Name"=w1780:string)  [unwired: 2 out]
                n1135 = Open VI Reference(type specifier VI Refnum (for type only)=refnum<vi> refnum, vi path=w1780, options=128) -> (vi reference=w1778:refnum<vi>)  [unwired: 3 in, 1 out]
                n1136 = call-by-ref "Start Asynchronous Call"(reference=w1778, "Y(mm)"=w1771, "X(mm)"=w1774) -> ()  [unwired: 10 in, 3 out]
              }
            }
            n1137 = property on="currentNO" class="Str"("Value"="E5") -> ()  [unwired: 2 in, 2 out]
          }
          event "E6": Value Change {
            n1138 = event-data() -> ("NewVal"=w1785:bool)  [unwired: 1 in, 5 out]
            n1139 = property on="移动" class="Bool (strict)"() -> ("Value"=w1788:bool)  [unwired: 2 in, 2 out]
            n1140 = Not(x=w1788) -> (.not. x?=w1787:bool)
            n1141 = And(x=w1787, y=w1785) -> (x .and. y?=w1786:bool)
            n1142 = case shown="True" w1786 {
              frame False {
              }
              frame True {
                n1143 = property on="A1-position-X" class="DigNum (strict)"() -> (error out=w1795:errorcluster, "Value"=w1802:dbl)  [unwired: 2 in, 1 out]
                n1144 = property on="A1-position-Y" class="DigNum (strict)"(error in=w1795) -> (error out=w1794:errorcluster, "Value"=w1791:dbl)  [unwired: 1 in, 1 out]
                n1145 = Subtract(x=w1791, y=18.0) -> (x-y=w1790:dbl)
                n1146 = Subtract(x=w1802, y=22.5) -> (x-y=w1793:dbl)
                n1147 = vi-ref "goto.vi"() -> (w1800:refnum<vi>)
                n1148 = property class="VI"(reference=w1800, error in=w1794) -> ("Name"=w1799:string)  [unwired: 2 out]
                n1149 = Open VI Reference(type specifier VI Refnum (for type only)=refnum<vi> refnum, vi path=w1799, options=128) -> (vi reference=w1797:refnum<vi>)  [unwired: 3 in, 1 out]
                n1150 = call-by-ref "Start Asynchronous Call"(reference=w1797, "Y(mm)"=w1790, "X(mm)"=w1793) -> ()  [unwired: 10 in, 3 out]
              }
            }
            n1151 = property on="currentNO" class="Str"("Value"="E6") -> ()  [unwired: 2 in, 2 out]
          }
          event "E7": Value Change {
            n1152 = event-data() -> ("NewVal"=w1804:bool)  [unwired: 1 in, 5 out]
            n1153 = property on="移动" class="Bool (strict)"() -> ("Value"=w1807:bool)  [unwired: 2 in, 2 out]
            n1154 = Not(x=w1807) -> (.not. x?=w1806:bool)
            n1155 = And(x=w1806, y=w1804) -> (x .and. y?=w1805:bool)
            n1156 = case shown="True" w1805 {
              frame False {
              }
              frame True {
                n1157 = property on="A1-position-X" class="DigNum (strict)"() -> (error out=w1814:errorcluster, "Value"=w1821:dbl)  [unwired: 2 in, 1 out]
                n1158 = property on="A1-position-Y" class="DigNum (strict)"(error in=w1814) -> (error out=w1813:errorcluster, "Value"=w1810:dbl)  [unwired: 1 in, 1 out]
                n1159 = Subtract(x=w1810, y=18.0) -> (x-y=w1809:dbl)
                n1160 = Subtract(x=w1821, y=27) -> (x-y=w1812:dbl)
                n1161 = vi-ref "goto.vi"() -> (w1819:refnum<vi>)
                n1162 = property class="VI"(reference=w1819, error in=w1813) -> ("Name"=w1818:string)  [unwired: 2 out]
                n1163 = Open VI Reference(type specifier VI Refnum (for type only)=refnum<vi> refnum, vi path=w1818, options=128) -> (vi reference=w1816:refnum<vi>)  [unwired: 3 in, 1 out]
                n1164 = call-by-ref "Start Asynchronous Call"(reference=w1816, "Y(mm)"=w1809, "X(mm)"=w1812) -> ()  [unwired: 10 in, 3 out]
              }
            }
            n1165 = property on="currentNO" class="Str"("Value"="E7") -> ()  [unwired: 2 in, 2 out]
          }
          event "E8": Value Change {
            n1166 = event-data() -> ("NewVal"=w1823:bool)  [unwired: 1 in, 5 out]
            n1167 = property on="移动" class="Bool (strict)"() -> ("Value"=w1826:bool)  [unwired: 2 in, 2 out]
            n1168 = Not(x=w1826) -> (.not. x?=w1825:bool)
            n1169 = And(x=w1825, y=w1823) -> (x .and. y?=w1824:bool)
            n1170 = case shown="True" w1824 {
              frame False {
              }
              frame True {
                n1171 = property on="A1-position-X" class="DigNum (strict)"() -> (error out=w1833:errorcluster, "Value"=w1840:dbl)  [unwired: 2 in, 1 out]
                n1172 = property on="A1-position-Y" class="DigNum (strict)"(error in=w1833) -> (error out=w1832:errorcluster, "Value"=w1829:dbl)  [unwired: 1 in, 1 out]
                n1173 = Subtract(x=w1829, y=18.0) -> (x-y=w1828:dbl)
                n1174 = Subtract(x=w1840, y=31.5) -> (x-y=w1831:dbl)
                n1175 = vi-ref "goto.vi"() -> (w1838:refnum<vi>)
                n1176 = property class="VI"(reference=w1838, error in=w1832) -> ("Name"=w1837:string)  [unwired: 2 out]
                n1177 = Open VI Reference(type specifier VI Refnum (for type only)=refnum<vi> refnum, vi path=w1837, options=128) -> (vi reference=w1835:refnum<vi>)  [unwired: 3 in, 1 out]
                n1178 = call-by-ref "Start Asynchronous Call"(reference=w1835, "Y(mm)"=w1828, "X(mm)"=w1831) -> ()  [unwired: 10 in, 3 out]
              }
            }
            n1179 = property on="currentNO" class="Str"("Value"="E8") -> ()  [unwired: 2 in, 2 out]
          }
          event "E9": Value Change {
            n1180 = event-data() -> ("NewVal"=w1842:bool)  [unwired: 1 in, 5 out]
            n1181 = property on="移动" class="Bool (strict)"() -> ("Value"=w1845:bool)  [unwired: 2 in, 2 out]
            n1182 = Not(x=w1845) -> (.not. x?=w1844:bool)
            n1183 = And(x=w1844, y=w1842) -> (x .and. y?=w1843:bool)
            n1184 = case shown="True" w1843 {
              frame False {
              }
              frame True {
                n1185 = property on="A1-position-X" class="DigNum (strict)"() -> (error out=w1852:errorcluster, "Value"=w1859:dbl)  [unwired: 2 in, 1 out]
                n1186 = property on="A1-position-Y" class="DigNum (strict)"(error in=w1852) -> (error out=w1851:errorcluster, "Value"=w1848:dbl)  [unwired: 1 in, 1 out]
                n1187 = Subtract(x=w1848, y=18.0) -> (x-y=w1847:dbl)
                n1188 = Subtract(x=w1859, y=36.0) -> (x-y=w1850:dbl)
                n1189 = vi-ref "goto.vi"() -> (w1857:refnum<vi>)
                n1190 = property class="VI"(reference=w1857, error in=w1851) -> ("Name"=w1856:string)  [unwired: 2 out]
                n1191 = Open VI Reference(type specifier VI Refnum (for type only)=refnum<vi> refnum, vi path=w1856, options=128) -> (vi reference=w1854:refnum<vi>)  [unwired: 3 in, 1 out]
                n1192 = call-by-ref "Start Asynchronous Call"(reference=w1854, "Y(mm)"=w1847, "X(mm)"=w1850) -> ()  [unwired: 10 in, 3 out]
              }
            }
            n1193 = property on="currentNO" class="Str"("Value"="E9") -> ()  [unwired: 2 in, 2 out]
          }
          event "E10": Value Change {
            n1194 = event-data() -> ("NewVal"=w1861:bool)  [unwired: 1 in, 5 out]
            n1195 = property on="移动" class="Bool (strict)"() -> ("Value"=w1862:bool)  [unwired: 2 in, 2 out]
            n1196 = Not(x=w1862) -> (.not. x?=w1863:bool)
            n1197 = And(x=w1863, y=w1861) -> (x .and. y?=w1864:bool)
            n1198 = case shown="True" w1864 {
              frame False {
              }
              frame True {
                n1199 = property on="A1-position-X" class="DigNum (strict)"() -> (error out=w1871:errorcluster, "Value"=w1878:dbl)  [unwired: 2 in, 1 out]
                n1200 = property on="A1-position-Y" class="DigNum (strict)"(error in=w1871) -> (error out=w1870:errorcluster, "Value"=w1867:dbl)  [unwired: 1 in, 1 out]
                n1201 = Subtract(x=w1867, y=18.0) -> (x-y=w1866:dbl)
                n1202 = Subtract(x=w1878, y=40.5) -> (x-y=w1869:dbl)
                n1203 = vi-ref "goto.vi"() -> (w1876:refnum<vi>)
                n1204 = property class="VI"(reference=w1876, error in=w1870) -> ("Name"=w1875:string)  [unwired: 2 out]
                n1205 = Open VI Reference(type specifier VI Refnum (for type only)=refnum<vi> refnum, vi path=w1875, options=128) -> (vi reference=w1873:refnum<vi>)  [unwired: 3 in, 1 out]
                n1206 = call-by-ref "Start Asynchronous Call"(reference=w1873, "Y(mm)"=w1866, "X(mm)"=w1869) -> ()  [unwired: 10 in, 3 out]
              }
            }
            n1207 = property on="currentNO" class="Str"("Value"="E10") -> ()  [unwired: 2 in, 2 out]
          }
          event "E11": Value Change {
            n1208 = event-data() -> ("NewVal"=w1880:bool)  [unwired: 1 in, 5 out]
            n1209 = property on="移动" class="Bool (strict)"() -> ("Value"=w1883:bool)  [unwired: 2 in, 2 out]
            n1210 = Not(x=w1883) -> (.not. x?=w1882:bool)
            n1211 = And(x=w1882, y=w1880) -> (x .and. y?=w1881:bool)
            n1212 = case shown="True" w1881 {
              frame False {
              }
              frame True {
                n1213 = property on="A1-position-X" class="DigNum (strict)"() -> (error out=w1890:errorcluster, "Value"=w1897:dbl)  [unwired: 2 in, 1 out]
                n1214 = property on="A1-position-Y" class="DigNum (strict)"(error in=w1890) -> (error out=w1889:errorcluster, "Value"=w1886:dbl)  [unwired: 1 in, 1 out]
                n1215 = Subtract(x=w1886, y=18.0) -> (x-y=w1885:dbl)
                n1216 = Subtract(x=w1897, y=45.0) -> (x-y=w1888:dbl)
                n1217 = vi-ref "goto.vi"() -> (w1895:refnum<vi>)
                n1218 = property class="VI"(reference=w1895, error in=w1889) -> ("Name"=w1894:string)  [unwired: 2 out]
                n1219 = Open VI Reference(type specifier VI Refnum (for type only)=refnum<vi> refnum, vi path=w1894, options=128) -> (vi reference=w1892:refnum<vi>)  [unwired: 3 in, 1 out]
                n1220 = call-by-ref "Start Asynchronous Call"(reference=w1892, "Y(mm)"=w1885, "X(mm)"=w1888) -> ()  [unwired: 10 in, 3 out]
              }
            }
            n1221 = property on="currentNO" class="Str"("Value"="E11") -> ()  [unwired: 2 in, 2 out]
          }
          event "E12": Value Change {
            n1222 = event-data() -> ("NewVal"=w1899:bool)  [unwired: 1 in, 5 out]
            n1223 = property on="移动" class="Bool (strict)"() -> ("Value"=w1902:bool)  [unwired: 2 in, 2 out]
            n1224 = Not(x=w1902) -> (.not. x?=w1901:bool)
            n1225 = And(x=w1901, y=w1899) -> (x .and. y?=w1900:bool)
            n1226 = case shown="True" w1900 {
              frame False {
              }
              frame True {
                n1227 = property on="A1-position-X" class="DigNum (strict)"() -> (error out=w1909:errorcluster, "Value"=w1916:dbl)  [unwired: 2 in, 1 out]
                n1228 = property on="A1-position-Y" class="DigNum (strict)"(error in=w1909) -> (error out=w1908:errorcluster, "Value"=w1905:dbl)  [unwired: 1 in, 1 out]
                n1229 = Subtract(x=w1905, y=18.0) -> (x-y=w1904:dbl)
                n1230 = Subtract(x=w1916, y=49.5) -> (x-y=w1907:dbl)
                n1231 = vi-ref "goto.vi"() -> (w1914:refnum<vi>)
                n1232 = property class="VI"(reference=w1914, error in=w1908) -> ("Name"=w1913:string)  [unwired: 2 out]
                n1233 = Open VI Reference(type specifier VI Refnum (for type only)=refnum<vi> refnum, vi path=w1913, options=128) -> (vi reference=w1911:refnum<vi>)  [unwired: 3 in, 1 out]
                n1234 = call-by-ref "Start Asynchronous Call"(reference=w1911, "Y(mm)"=w1904, "X(mm)"=w1907) -> ()  [unwired: 10 in, 3 out]
              }
            }
            n1235 = property on="currentNO" class="Str"("Value"="E12") -> ()  [unwired: 2 in, 2 out]
          }
          event "F1": Value Change {
            n1236 = event-data() -> ("NewVal"=w1918:bool)  [unwired: 1 in, 5 out]
            n1237 = property on="移动" class="Bool (strict)"() -> ("Value"=w1921:bool)  [unwired: 2 in, 2 out]
            n1238 = Not(x=w1921) -> (.not. x?=w1920:bool)
            n1239 = And(x=w1920, y=w1918) -> (x .and. y?=w1919:bool)
            n1240 = case shown="True" w1919 {
              frame False {
              }
              frame True {
                n1241 = property on="A1-position-X" class="DigNum (strict)"() -> (error out=w1928:errorcluster, "Value"=w1935:dbl)  [unwired: 2 in, 1 out]
                n1242 = property on="A1-position-Y" class="DigNum (strict)"(error in=w1928) -> (error out=w1927:errorcluster, "Value"=w1924:dbl)  [unwired: 1 in, 1 out]
                n1243 = Subtract(x=w1924, y=22.5) -> (x-y=w1923:dbl)
                n1244 = Subtract(x=w1935, y=0) -> (x-y=w1926:dbl)
                n1245 = vi-ref "goto.vi"() -> (w1933:refnum<vi>)
                n1246 = property class="VI"(reference=w1933, error in=w1927) -> ("Name"=w1932:string)  [unwired: 2 out]
                n1247 = Open VI Reference(type specifier VI Refnum (for type only)=refnum<vi> refnum, vi path=w1932, options=128) -> (vi reference=w1930:refnum<vi>)  [unwired: 3 in, 1 out]
                n1248 = call-by-ref "Start Asynchronous Call"(reference=w1930, "Y(mm)"=w1923, "X(mm)"=w1926) -> ()  [unwired: 10 in, 3 out]
              }
            }
            n1249 = property on="currentNO" class="Str"("Value"="F1") -> ()  [unwired: 2 in, 2 out]
          }
          event "F2": Value Change {
            n1250 = event-data() -> ("NewVal"=w1937:bool)  [unwired: 1 in, 5 out]
            n1251 = property on="移动" class="Bool (strict)"() -> ("Value"=w1938:bool)  [unwired: 2 in, 2 out]
            n1252 = Not(x=w1938) -> (.not. x?=w1939:bool)
            n1253 = And(x=w1939, y=w1937) -> (x .and. y?=w1940:bool)
            n1254 = case shown="True" w1940 {
              frame False {
              }
              frame True {
                n1255 = property on="A1-position-X" class="DigNum (strict)"() -> (error out=w1947:errorcluster, "Value"=w1954:dbl)  [unwired: 2 in, 1 out]
                n1256 = property on="A1-position-Y" class="DigNum (strict)"(error in=w1947) -> (error out=w1946:errorcluster, "Value"=w1943:dbl)  [unwired: 1 in, 1 out]
                n1257 = Subtract(x=w1943, y=22.5) -> (x-y=w1942:dbl)
                n1258 = Subtract(x=w1954, y=4.5) -> (x-y=w1945:dbl)
                n1259 = vi-ref "goto.vi"() -> (w1952:refnum<vi>)
                n1260 = property class="VI"(reference=w1952, error in=w1946) -> ("Name"=w1951:string)  [unwired: 2 out]
                n1261 = Open VI Reference(type specifier VI Refnum (for type only)=refnum<vi> refnum, vi path=w1951, options=128) -> (vi reference=w1949:refnum<vi>)  [unwired: 3 in, 1 out]
                n1262 = call-by-ref "Start Asynchronous Call"(reference=w1949, "Y(mm)"=w1942, "X(mm)"=w1945) -> ()  [unwired: 10 in, 3 out]
              }
            }
            n1263 = property on="currentNO" class="Str"("Value"="F2") -> ()  [unwired: 2 in, 2 out]
          }
          event "F3": Value Change {
            n1264 = event-data() -> ("NewVal"=w1956:bool)  [unwired: 1 in, 5 out]
            n1265 = property on="移动" class="Bool (strict)"() -> ("Value"=w1957:bool)  [unwired: 2 in, 2 out]
            n1266 = Not(x=w1957) -> (.not. x?=w1958:bool)
            n1267 = And(x=w1958, y=w1956) -> (x .and. y?=w1959:bool)
            n1268 = case shown="True" w1959 {
              frame False {
              }
              frame True {
                n1269 = property on="A1-position-X" class="DigNum (strict)"() -> (error out=w1966:errorcluster, "Value"=w1973:dbl)  [unwired: 2 in, 1 out]
                n1270 = property on="A1-position-Y" class="DigNum (strict)"(error in=w1966) -> (error out=w1965:errorcluster, "Value"=w1962:dbl)  [unwired: 1 in, 1 out]
                n1271 = Subtract(x=w1962, y=22.5) -> (x-y=w1961:dbl)
                n1272 = Subtract(x=w1973, y=9) -> (x-y=w1964:dbl)
                n1273 = vi-ref "goto.vi"() -> (w1971:refnum<vi>)
                n1274 = property class="VI"(reference=w1971, error in=w1965) -> ("Name"=w1970:string)  [unwired: 2 out]
                n1275 = Open VI Reference(type specifier VI Refnum (for type only)=refnum<vi> refnum, vi path=w1970, options=128) -> (vi reference=w1968:refnum<vi>)  [unwired: 3 in, 1 out]
                n1276 = call-by-ref "Start Asynchronous Call"(reference=w1968, "Y(mm)"=w1961, "X(mm)"=w1964) -> ()  [unwired: 10 in, 3 out]
              }
            }
            n1277 = property on="currentNO" class="Str"("Value"="F3") -> ()  [unwired: 2 in, 2 out]
          }
          event "F4": Value Change {
            n1278 = event-data() -> ("NewVal"=w1975:bool)  [unwired: 1 in, 5 out]
            n1279 = property on="移动" class="Bool (strict)"() -> ("Value"=w1978:bool)  [unwired: 2 in, 2 out]
            n1280 = Not(x=w1978) -> (.not. x?=w1977:bool)
            n1281 = And(x=w1977, y=w1975) -> (x .and. y?=w1976:bool)
            n1282 = case shown="True" w1976 {
              frame False {
              }
              frame True {
                n1283 = property on="A1-position-X" class="DigNum (strict)"() -> (error out=w1985:errorcluster, "Value"=w1992:dbl)  [unwired: 2 in, 1 out]
                n1284 = property on="A1-position-Y" class="DigNum (strict)"(error in=w1985) -> (error out=w1984:errorcluster, "Value"=w1981:dbl)  [unwired: 1 in, 1 out]
                n1285 = Subtract(x=w1981, y=22.5) -> (x-y=w1980:dbl)
                n1286 = Subtract(x=w1992, y=13.5) -> (x-y=w1983:dbl)
                n1287 = vi-ref "goto.vi"() -> (w1990:refnum<vi>)
                n1288 = property class="VI"(reference=w1990, error in=w1984) -> ("Name"=w1989:string)  [unwired: 2 out]
                n1289 = Open VI Reference(type specifier VI Refnum (for type only)=refnum<vi> refnum, vi path=w1989, options=128) -> (vi reference=w1987:refnum<vi>)  [unwired: 3 in, 1 out]
                n1290 = call-by-ref "Start Asynchronous Call"(reference=w1987, "Y(mm)"=w1980, "X(mm)"=w1983) -> ()  [unwired: 10 in, 3 out]
              }
            }
            n1291 = property on="currentNO" class="Str"("Value"="F4") -> ()  [unwired: 2 in, 2 out]
          }
          event "F5": Value Change {
            n1292 = event-data() -> ("NewVal"=w1994:bool)  [unwired: 1 in, 5 out]
            n1293 = property on="移动" class="Bool (strict)"() -> ("Value"=w1997:bool)  [unwired: 2 in, 2 out]
            n1294 = Not(x=w1997) -> (.not. x?=w1996:bool)
            n1295 = And(x=w1996, y=w1994) -> (x .and. y?=w1995:bool)
            n1296 = case shown="True" w1995 {
              frame False {
              }
              frame True {
                n1297 = property on="A1-position-X" class="DigNum (strict)"() -> (error out=w2004:errorcluster, "Value"=w2011:dbl)  [unwired: 2 in, 1 out]
                n1298 = property on="A1-position-Y" class="DigNum (strict)"(error in=w2004) -> (error out=w2003:errorcluster, "Value"=w2000:dbl)  [unwired: 1 in, 1 out]
                n1299 = Subtract(x=w2000, y=22.5) -> (x-y=w1999:dbl)
                n1300 = Subtract(x=w2011, y=18.0) -> (x-y=w2002:dbl)
                n1301 = vi-ref "goto.vi"() -> (w2009:refnum<vi>)
                n1302 = property class="VI"(reference=w2009, error in=w2003) -> ("Name"=w2008:string)  [unwired: 2 out]
                n1303 = Open VI Reference(type specifier VI Refnum (for type only)=refnum<vi> refnum, vi path=w2008, options=128) -> (vi reference=w2006:refnum<vi>)  [unwired: 3 in, 1 out]
                n1304 = call-by-ref "Start Asynchronous Call"(reference=w2006, "Y(mm)"=w1999, "X(mm)"=w2002) -> ()  [unwired: 10 in, 3 out]
              }
            }
            n1305 = property on="currentNO" class="Str"("Value"="F5") -> ()  [unwired: 2 in, 2 out]
          }
          event "F6": Value Change {
            n1306 = event-data() -> ("NewVal"=w2013:bool)  [unwired: 1 in, 5 out]
            n1307 = property on="移动" class="Bool (strict)"() -> ("Value"=w2016:bool)  [unwired: 2 in, 2 out]
            n1308 = Not(x=w2016) -> (.not. x?=w2015:bool)
            n1309 = And(x=w2015, y=w2013) -> (x .and. y?=w2014:bool)
            n1310 = case shown="True" w2014 {
              frame False {
              }
              frame True {
                n1311 = property on="A1-position-X" class="DigNum (strict)"() -> (error out=w2023:errorcluster, "Value"=w2030:dbl)  [unwired: 2 in, 1 out]
                n1312 = property on="A1-position-Y" class="DigNum (strict)"(error in=w2023) -> (error out=w2022:errorcluster, "Value"=w2019:dbl)  [unwired: 1 in, 1 out]
                n1313 = Subtract(x=w2019, y=22.5) -> (x-y=w2018:dbl)
                n1314 = Subtract(x=w2030, y=22.5) -> (x-y=w2021:dbl)
                n1315 = vi-ref "goto.vi"() -> (w2028:refnum<vi>)
                n1316 = property class="VI"(reference=w2028, error in=w2022) -> ("Name"=w2027:string)  [unwired: 2 out]
                n1317 = Open VI Reference(type specifier VI Refnum (for type only)=refnum<vi> refnum, vi path=w2027, options=128) -> (vi reference=w2025:refnum<vi>)  [unwired: 3 in, 1 out]
                n1318 = call-by-ref "Start Asynchronous Call"(reference=w2025, "Y(mm)"=w2018, "X(mm)"=w2021) -> ()  [unwired: 10 in, 3 out]
              }
            }
            n1319 = property on="currentNO" class="Str"("Value"="F6") -> ()  [unwired: 2 in, 2 out]
          }
          event "F7": Value Change {
            n1320 = event-data() -> ("NewVal"=w2032:bool)  [unwired: 1 in, 5 out]
            n1321 = property on="移动" class="Bool (strict)"() -> ("Value"=w2035:bool)  [unwired: 2 in, 2 out]
            n1322 = Not(x=w2035) -> (.not. x?=w2034:bool)
            n1323 = And(x=w2034, y=w2032) -> (x .and. y?=w2033:bool)
            n1324 = case shown="True" w2033 {
              frame False {
              }
              frame True {
                n1325 = property on="A1-position-X" class="DigNum (strict)"() -> (error out=w2042:errorcluster, "Value"=w2049:dbl)  [unwired: 2 in, 1 out]
                n1326 = property on="A1-position-Y" class="DigNum (strict)"(error in=w2042) -> (error out=w2041:errorcluster, "Value"=w2038:dbl)  [unwired: 1 in, 1 out]
                n1327 = Subtract(x=w2038, y=22.5) -> (x-y=w2037:dbl)
                n1328 = Subtract(x=w2049, y=27) -> (x-y=w2040:dbl)
                n1329 = vi-ref "goto.vi"() -> (w2047:refnum<vi>)
                n1330 = property class="VI"(reference=w2047, error in=w2041) -> ("Name"=w2046:string)  [unwired: 2 out]
                n1331 = Open VI Reference(type specifier VI Refnum (for type only)=refnum<vi> refnum, vi path=w2046, options=128) -> (vi reference=w2044:refnum<vi>)  [unwired: 3 in, 1 out]
                n1332 = call-by-ref "Start Asynchronous Call"(reference=w2044, "Y(mm)"=w2037, "X(mm)"=w2040) -> ()  [unwired: 10 in, 3 out]
              }
            }
            n1333 = property on="currentNO" class="Str"("Value"="F7") -> ()  [unwired: 2 in, 2 out]
          }
          event "F8": Value Change {
            n1334 = event-data() -> ("NewVal"=w2051:bool)  [unwired: 1 in, 5 out]
            n1335 = property on="移动" class="Bool (strict)"() -> ("Value"=w2054:bool)  [unwired: 2 in, 2 out]
            n1336 = Not(x=w2054) -> (.not. x?=w2053:bool)
            n1337 = And(x=w2053, y=w2051) -> (x .and. y?=w2052:bool)
            n1338 = case shown="True" w2052 {
              frame False {
              }
              frame True {
                n1339 = property on="A1-position-X" class="DigNum (strict)"() -> (error out=w2061:errorcluster, "Value"=w2068:dbl)  [unwired: 2 in, 1 out]
                n1340 = property on="A1-position-Y" class="DigNum (strict)"(error in=w2061) -> (error out=w2060:errorcluster, "Value"=w2057:dbl)  [unwired: 1 in, 1 out]
                n1341 = Subtract(x=w2057, y=22.5) -> (x-y=w2056:dbl)
                n1342 = Subtract(x=w2068, y=31.5) -> (x-y=w2059:dbl)
                n1343 = vi-ref "goto.vi"() -> (w2066:refnum<vi>)
                n1344 = property class="VI"(reference=w2066, error in=w2060) -> ("Name"=w2065:string)  [unwired: 2 out]
                n1345 = Open VI Reference(type specifier VI Refnum (for type only)=refnum<vi> refnum, vi path=w2065, options=128) -> (vi reference=w2063:refnum<vi>)  [unwired: 3 in, 1 out]
                n1346 = call-by-ref "Start Asynchronous Call"(reference=w2063, "Y(mm)"=w2056, "X(mm)"=w2059) -> ()  [unwired: 10 in, 3 out]
              }
            }
            n1347 = property on="currentNO" class="Str"("Value"="F8") -> ()  [unwired: 2 in, 2 out]
          }
          event "F9": Value Change {
            n1348 = event-data() -> ("NewVal"=w2070:bool)  [unwired: 1 in, 5 out]
            n1349 = property on="移动" class="Bool (strict)"() -> ("Value"=w2073:bool)  [unwired: 2 in, 2 out]
            n1350 = Not(x=w2073) -> (.not. x?=w2072:bool)
            n1351 = And(x=w2072, y=w2070) -> (x .and. y?=w2071:bool)
            n1352 = case shown="True" w2071 {
              frame False {
              }
              frame True {
                n1353 = property on="A1-position-X" class="DigNum (strict)"() -> (error out=w2080:errorcluster, "Value"=w2087:dbl)  [unwired: 2 in, 1 out]
                n1354 = property on="A1-position-Y" class="DigNum (strict)"(error in=w2080) -> (error out=w2079:errorcluster, "Value"=w2076:dbl)  [unwired: 1 in, 1 out]
                n1355 = Subtract(x=w2076, y=22.5) -> (x-y=w2075:dbl)
                n1356 = Subtract(x=w2087, y=36) -> (x-y=w2078:dbl)
                n1357 = vi-ref "goto.vi"() -> (w2085:refnum<vi>)
                n1358 = property class="VI"(reference=w2085, error in=w2079) -> ("Name"=w2084:string)  [unwired: 2 out]
                n1359 = Open VI Reference(type specifier VI Refnum (for type only)=refnum<vi> refnum, vi path=w2084, options=128) -> (vi reference=w2082:refnum<vi>)  [unwired: 3 in, 1 out]
                n1360 = call-by-ref "Start Asynchronous Call"(reference=w2082, "Y(mm)"=w2075, "X(mm)"=w2078) -> ()  [unwired: 10 in, 3 out]
              }
            }
            n1361 = property on="currentNO" class="Str"("Value"="F9") -> ()  [unwired: 2 in, 2 out]
          }
          event "F10": Value Change {
            n1362 = event-data() -> ("NewVal"=w2089:bool)  [unwired: 1 in, 5 out]
            n1363 = property on="移动" class="Bool (strict)"() -> ("Value"=w2092:bool)  [unwired: 2 in, 2 out]
            n1364 = Not(x=w2092) -> (.not. x?=w2091:bool)
            n1365 = And(x=w2091, y=w2089) -> (x .and. y?=w2090:bool)
            n1366 = case shown="True" w2090 {
              frame False {
              }
              frame True {
                n1367 = property on="A1-position-X" class="DigNum (strict)"() -> (error out=w2099:errorcluster, "Value"=w2106:dbl)  [unwired: 2 in, 1 out]
                n1368 = property on="A1-position-Y" class="DigNum (strict)"(error in=w2099) -> (error out=w2098:errorcluster, "Value"=w2095:dbl)  [unwired: 1 in, 1 out]
                n1369 = Subtract(x=w2095, y=22.5) -> (x-y=w2094:dbl)
                n1370 = Subtract(x=w2106, y=40.5) -> (x-y=w2097:dbl)
                n1371 = vi-ref "goto.vi"() -> (w2104:refnum<vi>)
                n1372 = property class="VI"(reference=w2104, error in=w2098) -> ("Name"=w2103:string)  [unwired: 2 out]
                n1373 = Open VI Reference(type specifier VI Refnum (for type only)=refnum<vi> refnum, vi path=w2103, options=128) -> (vi reference=w2101:refnum<vi>)  [unwired: 3 in, 1 out]
                n1374 = call-by-ref "Start Asynchronous Call"(reference=w2101, "Y(mm)"=w2094, "X(mm)"=w2097) -> ()  [unwired: 10 in, 3 out]
              }
            }
            n1375 = property on="currentNO" class="Str"("Value"="F10") -> ()  [unwired: 2 in, 2 out]
          }
          event "F11": Value Change {
            n1376 = event-data() -> ("NewVal"=w2108:bool)  [unwired: 1 in, 5 out]
            n1377 = property on="移动" class="Bool (strict)"() -> ("Value"=w2111:bool)  [unwired: 2 in, 2 out]
            n1378 = Not(x=w2111) -> (.not. x?=w2110:bool)
            n1379 = And(x=w2110, y=w2108) -> (x .and. y?=w2109:bool)
            n1380 = case shown="True" w2109 {
              frame False {
              }
              frame True {
                n1381 = property on="A1-position-X" class="DigNum (strict)"() -> (error out=w2118:errorcluster, "Value"=w2125:dbl)  [unwired: 2 in, 1 out]
                n1382 = property on="A1-position-Y" class="DigNum (strict)"(error in=w2118) -> (error out=w2117:errorcluster, "Value"=w2114:dbl)  [unwired: 1 in, 1 out]
                n1383 = Subtract(x=w2114, y=22.5) -> (x-y=w2113:dbl)
                n1384 = Subtract(x=w2125, y=45) -> (x-y=w2116:dbl)
                n1385 = vi-ref "goto.vi"() -> (w2123:refnum<vi>)
                n1386 = property class="VI"(reference=w2123, error in=w2117) -> ("Name"=w2122:string)  [unwired: 2 out]
                n1387 = Open VI Reference(type specifier VI Refnum (for type only)=refnum<vi> refnum, vi path=w2122, options=128) -> (vi reference=w2120:refnum<vi>)  [unwired: 3 in, 1 out]
                n1388 = call-by-ref "Start Asynchronous Call"(reference=w2120, "Y(mm)"=w2113, "X(mm)"=w2116) -> ()  [unwired: 10 in, 3 out]
              }
            }
            n1389 = property on="currentNO" class="Str"("Value"="F11") -> ()  [unwired: 2 in, 2 out]
          }
          event "F12": Value Change {
            n1390 = event-data() -> ("NewVal"=w2127:bool)  [unwired: 1 in, 5 out]
            n1391 = property on="移动" class="Bool (strict)"() -> ("Value"=w2130:bool)  [unwired: 2 in, 2 out]
            n1392 = Not(x=w2130) -> (.not. x?=w2129:bool)
            n1393 = And(x=w2129, y=w2127) -> (x .and. y?=w2128:bool)
            n1394 = case shown="True" w2128 {
              frame False {
              }
              frame True {
                n1395 = property on="A1-position-X" class="DigNum (strict)"() -> (error out=w2137:errorcluster, "Value"=w2144:dbl)  [unwired: 2 in, 1 out]
                n1396 = property on="A1-position-Y" class="DigNum (strict)"(error in=w2137) -> (error out=w2136:errorcluster, "Value"=w2133:dbl)  [unwired: 1 in, 1 out]
                n1397 = Subtract(x=w2133, y=22.5) -> (x-y=w2132:dbl)
                n1398 = Subtract(x=w2144, y=49.5) -> (x-y=w2135:dbl)
                n1399 = vi-ref "goto.vi"() -> (w2142:refnum<vi>)
                n1400 = property class="VI"(reference=w2142, error in=w2136) -> ("Name"=w2141:string)  [unwired: 2 out]
                n1401 = Open VI Reference(type specifier VI Refnum (for type only)=refnum<vi> refnum, vi path=w2141, options=128) -> (vi reference=w2139:refnum<vi>)  [unwired: 3 in, 1 out]
                n1402 = call-by-ref "Start Asynchronous Call"(reference=w2139, "Y(mm)"=w2132, "X(mm)"=w2135) -> ()  [unwired: 10 in, 3 out]
              }
            }
            n1403 = property on="currentNO" class="Str"("Value"="F12") -> ()  [unwired: 2 in, 2 out]
          }
          event "G1": Value Change {
            n1404 = event-data() -> ("NewVal"=w2146:bool)  [unwired: 1 in, 5 out]
            n1405 = property on="移动" class="Bool (strict)"() -> ("Value"=w2149:bool)  [unwired: 2 in, 2 out]
            n1406 = Not(x=w2149) -> (.not. x?=w2148:bool)
            n1407 = And(x=w2148, y=w2146) -> (x .and. y?=w2147:bool)
            n1408 = case shown="True" w2147 {
              frame False {
              }
              frame True {
                n1409 = property on="A1-position-X" class="DigNum (strict)"() -> (error out=w2156:errorcluster, "Value"=w2163:dbl)  [unwired: 2 in, 1 out]
                n1410 = property on="A1-position-Y" class="DigNum (strict)"(error in=w2156) -> (error out=w2155:errorcluster, "Value"=w2152:dbl)  [unwired: 1 in, 1 out]
                n1411 = Subtract(x=w2152, y=27.0) -> (x-y=w2151:dbl)
                n1412 = Subtract(x=w2163, y=0) -> (x-y=w2154:dbl)
                n1413 = vi-ref "goto.vi"() -> (w2161:refnum<vi>)
                n1414 = property class="VI"(reference=w2161, error in=w2155) -> ("Name"=w2160:string)  [unwired: 2 out]
                n1415 = Open VI Reference(type specifier VI Refnum (for type only)=refnum<vi> refnum, vi path=w2160, options=128) -> (vi reference=w2158:refnum<vi>)  [unwired: 3 in, 1 out]
                n1416 = call-by-ref "Start Asynchronous Call"(reference=w2158, "Y(mm)"=w2151, "X(mm)"=w2154) -> ()  [unwired: 10 in, 3 out]
              }
            }
            n1417 = property on="currentNO" class="Str"("Value"="G1") -> ()  [unwired: 2 in, 2 out]
          }
          event "G2": Value Change {
            n1418 = event-data() -> ("NewVal"=w2165:bool)  [unwired: 1 in, 5 out]
            n1419 = property on="移动" class="Bool (strict)"() -> ("Value"=w2168:bool)  [unwired: 2 in, 2 out]
            n1420 = Not(x=w2168) -> (.not. x?=w2167:bool)
            n1421 = And(x=w2167, y=w2165) -> (x .and. y?=w2166:bool)
            n1422 = case shown="True" w2166 {
              frame False {
              }
              frame True {
                n1423 = property on="A1-position-X" class="DigNum (strict)"() -> (error out=w2175:errorcluster, "Value"=w2182:dbl)  [unwired: 2 in, 1 out]
                n1424 = property on="A1-position-Y" class="DigNum (strict)"(error in=w2175) -> (error out=w2174:errorcluster, "Value"=w2171:dbl)  [unwired: 1 in, 1 out]
                n1425 = Subtract(x=w2171, y=27.0) -> (x-y=w2170:dbl)
                n1426 = Subtract(x=w2182, y=4.5) -> (x-y=w2173:dbl)
                n1427 = vi-ref "goto.vi"() -> (w2180:refnum<vi>)
                n1428 = property class="VI"(reference=w2180, error in=w2174) -> ("Name"=w2179:string)  [unwired: 2 out]
                n1429 = Open VI Reference(type specifier VI Refnum (for type only)=refnum<vi> refnum, vi path=w2179, options=128) -> (vi reference=w2177:refnum<vi>)  [unwired: 3 in, 1 out]
                n1430 = call-by-ref "Start Asynchronous Call"(reference=w2177, "Y(mm)"=w2170, "X(mm)"=w2173) -> ()  [unwired: 10 in, 3 out]
              }
            }
            n1431 = property on="currentNO" class="Str"("Value"="G2") -> ()  [unwired: 2 in, 2 out]
          }
          event "G3": Value Change {
            n1432 = event-data() -> ("NewVal"=w2184:bool)  [unwired: 1 in, 5 out]
            n1433 = property on="移动" class="Bool (strict)"() -> ("Value"=w2187:bool)  [unwired: 2 in, 2 out]
            n1434 = Not(x=w2187) -> (.not. x?=w2186:bool)
            n1435 = And(x=w2186, y=w2184) -> (x .and. y?=w2185:bool)
            n1436 = case shown="True" w2185 {
              frame False {
              }
              frame True {
                n1437 = property on="A1-position-X" class="DigNum (strict)"() -> (error out=w2194:errorcluster, "Value"=w2201:dbl)  [unwired: 2 in, 1 out]
                n1438 = property on="A1-position-Y" class="DigNum (strict)"(error in=w2194) -> (error out=w2193:errorcluster, "Value"=w2190:dbl)  [unwired: 1 in, 1 out]
                n1439 = Subtract(x=w2190, y=27.0) -> (x-y=w2189:dbl)
                n1440 = Subtract(x=w2201, y=9.0) -> (x-y=w2192:dbl)
                n1441 = vi-ref "goto.vi"() -> (w2199:refnum<vi>)
                n1442 = property class="VI"(reference=w2199, error in=w2193) -> ("Name"=w2198:string)  [unwired: 2 out]
                n1443 = Open VI Reference(type specifier VI Refnum (for type only)=refnum<vi> refnum, vi path=w2198, options=128) -> (vi reference=w2196:refnum<vi>)  [unwired: 3 in, 1 out]
                n1444 = call-by-ref "Start Asynchronous Call"(reference=w2196, "Y(mm)"=w2189, "X(mm)"=w2192) -> ()  [unwired: 10 in, 3 out]
              }
            }
            n1445 = property on="currentNO" class="Str"("Value"="G3") -> ()  [unwired: 2 in, 2 out]
          }
          event "G4": Value Change {
            n1446 = event-data() -> ("NewVal"=w2203:bool)  [unwired: 1 in, 5 out]
            n1447 = property on="移动" class="Bool (strict)"() -> ("Value"=w2206:bool)  [unwired: 2 in, 2 out]
            n1448 = Not(x=w2206) -> (.not. x?=w2205:bool)
            n1449 = And(x=w2205, y=w2203) -> (x .and. y?=w2204:bool)
            n1450 = case shown="True" w2204 {
              frame False {
              }
              frame True {
                n1451 = property on="A1-position-X" class="DigNum (strict)"() -> (error out=w2213:errorcluster, "Value"=w2220:dbl)  [unwired: 2 in, 1 out]
                n1452 = property on="A1-position-Y" class="DigNum (strict)"(error in=w2213) -> (error out=w2212:errorcluster, "Value"=w2209:dbl)  [unwired: 1 in, 1 out]
                n1453 = Subtract(x=w2209, y=27.0) -> (x-y=w2208:dbl)
                n1454 = Subtract(x=w2220, y=13.5) -> (x-y=w2211:dbl)
                n1455 = vi-ref "goto.vi"() -> (w2218:refnum<vi>)
                n1456 = property class="VI"(reference=w2218, error in=w2212) -> ("Name"=w2217:string)  [unwired: 2 out]
                n1457 = Open VI Reference(type specifier VI Refnum (for type only)=refnum<vi> refnum, vi path=w2217, options=128) -> (vi reference=w2215:refnum<vi>)  [unwired: 3 in, 1 out]
                n1458 = call-by-ref "Start Asynchronous Call"(reference=w2215, "Y(mm)"=w2208, "X(mm)"=w2211) -> ()  [unwired: 10 in, 3 out]
              }
            }
            n1459 = property on="currentNO" class="Str"("Value"="G4") -> ()  [unwired: 2 in, 2 out]
          }
          event "G5": Value Change {
            n1460 = event-data() -> ("NewVal"=w2222:bool)  [unwired: 1 in, 5 out]
            n1461 = property on="移动" class="Bool (strict)"() -> ("Value"=w2225:bool)  [unwired: 2 in, 2 out]
            n1462 = Not(x=w2225) -> (.not. x?=w2224:bool)
            n1463 = And(x=w2224, y=w2222) -> (x .and. y?=w2223:bool)
            n1464 = case shown="True" w2223 {
              frame False {
              }
              frame True {
                n1465 = property on="A1-position-X" class="DigNum (strict)"() -> (error out=w2232:errorcluster, "Value"=w2239:dbl)  [unwired: 2 in, 1 out]
                n1466 = property on="A1-position-Y" class="DigNum (strict)"(error in=w2232) -> (error out=w2231:errorcluster, "Value"=w2228:dbl)  [unwired: 1 in, 1 out]
                n1467 = Subtract(x=w2228, y=27.0) -> (x-y=w2227:dbl)
                n1468 = Subtract(x=w2239, y=18) -> (x-y=w2230:dbl)
                n1469 = vi-ref "goto.vi"() -> (w2237:refnum<vi>)
                n1470 = property class="VI"(reference=w2237, error in=w2231) -> ("Name"=w2236:string)  [unwired: 2 out]
                n1471 = Open VI Reference(type specifier VI Refnum (for type only)=refnum<vi> refnum, vi path=w2236, options=128) -> (vi reference=w2234:refnum<vi>)  [unwired: 3 in, 1 out]
                n1472 = call-by-ref "Start Asynchronous Call"(reference=w2234, "Y(mm)"=w2227, "X(mm)"=w2230) -> ()  [unwired: 10 in, 3 out]
              }
            }
            n1473 = property on="currentNO" class="Str"("Value"="G5") -> ()  [unwired: 2 in, 2 out]
          }
          event "G6": Value Change {
            n1474 = event-data() -> ("NewVal"=w2241:bool)  [unwired: 1 in, 5 out]
            n1475 = property on="移动" class="Bool (strict)"() -> ("Value"=w2244:bool)  [unwired: 2 in, 2 out]
            n1476 = Not(x=w2244) -> (.not. x?=w2243:bool)
            n1477 = And(x=w2243, y=w2241) -> (x .and. y?=w2242:bool)
            n1478 = case shown="True" w2242 {
              frame False {
              }
              frame True {
                n1479 = property on="A1-position-X" class="DigNum (strict)"() -> (error out=w2251:errorcluster, "Value"=w2258:dbl)  [unwired: 2 in, 1 out]
                n1480 = property on="A1-position-Y" class="DigNum (strict)"(error in=w2251) -> (error out=w2250:errorcluster, "Value"=w2247:dbl)  [unwired: 1 in, 1 out]
                n1481 = Subtract(x=w2247, y=27.0) -> (x-y=w2246:dbl)
                n1482 = Subtract(x=w2258, y=22.5) -> (x-y=w2249:dbl)
                n1483 = vi-ref "goto.vi"() -> (w2256:refnum<vi>)
                n1484 = property class="VI"(reference=w2256, error in=w2250) -> ("Name"=w2255:string)  [unwired: 2 out]
                n1485 = Open VI Reference(type specifier VI Refnum (for type only)=refnum<vi> refnum, vi path=w2255, options=128) -> (vi reference=w2253:refnum<vi>)  [unwired: 3 in, 1 out]
                n1486 = call-by-ref "Start Asynchronous Call"(reference=w2253, "Y(mm)"=w2246, "X(mm)"=w2249) -> ()  [unwired: 10 in, 3 out]
              }
            }
            n1487 = property on="currentNO" class="Str"("Value"="G6") -> ()  [unwired: 2 in, 2 out]
          }
          event "G7": Value Change {
            n1488 = event-data() -> ("NewVal"=w2260:bool)  [unwired: 1 in, 5 out]
            n1489 = property on="移动" class="Bool (strict)"() -> ("Value"=w2263:bool)  [unwired: 2 in, 2 out]
            n1490 = Not(x=w2263) -> (.not. x?=w2262:bool)
            n1491 = And(x=w2262, y=w2260) -> (x .and. y?=w2261:bool)
            n1492 = case shown="True" w2261 {
              frame False {
              }
              frame True {
                n1493 = property on="A1-position-X" class="DigNum (strict)"() -> (error out=w2270:errorcluster, "Value"=w2277:dbl)  [unwired: 2 in, 1 out]
                n1494 = property on="A1-position-Y" class="DigNum (strict)"(error in=w2270) -> (error out=w2269:errorcluster, "Value"=w2266:dbl)  [unwired: 1 in, 1 out]
                n1495 = Subtract(x=w2266, y=27.0) -> (x-y=w2265:dbl)
                n1496 = Subtract(x=w2277, y=27) -> (x-y=w2268:dbl)
                n1497 = vi-ref "goto.vi"() -> (w2275:refnum<vi>)
                n1498 = property class="VI"(reference=w2275, error in=w2269) -> ("Name"=w2274:string)  [unwired: 2 out]
                n1499 = Open VI Reference(type specifier VI Refnum (for type only)=refnum<vi> refnum, vi path=w2274, options=128) -> (vi reference=w2272:refnum<vi>)  [unwired: 3 in, 1 out]
                n1500 = call-by-ref "Start Asynchronous Call"(reference=w2272, "Y(mm)"=w2265, "X(mm)"=w2268) -> ()  [unwired: 10 in, 3 out]
              }
            }
            n1501 = property on="currentNO" class="Str"("Value"="G7") -> ()  [unwired: 2 in, 2 out]
          }
          event "G8": Value Change {
            n1502 = event-data() -> ("NewVal"=w2279:bool)  [unwired: 1 in, 5 out]
            n1503 = property on="移动" class="Bool (strict)"() -> ("Value"=w2282:bool)  [unwired: 2 in, 2 out]
            n1504 = Not(x=w2282) -> (.not. x?=w2281:bool)
            n1505 = And(x=w2281, y=w2279) -> (x .and. y?=w2280:bool)
            n1506 = case shown="True" w2280 {
              frame False {
              }
              frame True {
                n1507 = property on="A1-position-X" class="DigNum (strict)"() -> (error out=w2289:errorcluster, "Value"=w2296:dbl)  [unwired: 2 in, 1 out]
                n1508 = property on="A1-position-Y" class="DigNum (strict)"(error in=w2289) -> (error out=w2288:errorcluster, "Value"=w2285:dbl)  [unwired: 1 in, 1 out]
                n1509 = Subtract(x=w2285, y=27.0) -> (x-y=w2284:dbl)
                n1510 = Subtract(x=w2296, y=31.5) -> (x-y=w2287:dbl)
                n1511 = vi-ref "goto.vi"() -> (w2294:refnum<vi>)
                n1512 = property class="VI"(reference=w2294, error in=w2288) -> ("Name"=w2293:string)  [unwired: 2 out]
                n1513 = Open VI Reference(type specifier VI Refnum (for type only)=refnum<vi> refnum, vi path=w2293, options=128) -> (vi reference=w2291:refnum<vi>)  [unwired: 3 in, 1 out]
                n1514 = call-by-ref "Start Asynchronous Call"(reference=w2291, "Y(mm)"=w2284, "X(mm)"=w2287) -> ()  [unwired: 10 in, 3 out]
              }
            }
            n1515 = property on="currentNO" class="Str"("Value"="G8") -> ()  [unwired: 2 in, 2 out]
          }
          event "G9": Value Change {
            n1516 = event-data() -> ("NewVal"=w2298:bool)  [unwired: 1 in, 5 out]
            n1517 = property on="移动" class="Bool (strict)"() -> ("Value"=w2301:bool)  [unwired: 2 in, 2 out]
            n1518 = Not(x=w2301) -> (.not. x?=w2300:bool)
            n1519 = And(x=w2300, y=w2298) -> (x .and. y?=w2299:bool)
            n1520 = case shown="True" w2299 {
              frame False {
              }
              frame True {
                n1521 = property on="A1-position-X" class="DigNum (strict)"() -> (error out=w2308:errorcluster, "Value"=w2315:dbl)  [unwired: 2 in, 1 out]
                n1522 = property on="A1-position-Y" class="DigNum (strict)"(error in=w2308) -> (error out=w2307:errorcluster, "Value"=w2304:dbl)  [unwired: 1 in, 1 out]
                n1523 = Subtract(x=w2304, y=27.0) -> (x-y=w2303:dbl)
                n1524 = Subtract(x=w2315, y=36.0) -> (x-y=w2306:dbl)
                n1525 = vi-ref "goto.vi"() -> (w2313:refnum<vi>)
                n1526 = property class="VI"(reference=w2313, error in=w2307) -> ("Name"=w2312:string)  [unwired: 2 out]
                n1527 = Open VI Reference(type specifier VI Refnum (for type only)=refnum<vi> refnum, vi path=w2312, options=128) -> (vi reference=w2310:refnum<vi>)  [unwired: 3 in, 1 out]
                n1528 = call-by-ref "Start Asynchronous Call"(reference=w2310, "Y(mm)"=w2303, "X(mm)"=w2306) -> ()  [unwired: 10 in, 3 out]
              }
            }
            n1529 = property on="currentNO" class="Str"("Value"="G9") -> ()  [unwired: 2 in, 2 out]
          }
          event "G10": Value Change {
            n1530 = event-data() -> ("NewVal"=w2317:bool)  [unwired: 1 in, 5 out]
            n1531 = property on="移动" class="Bool (strict)"() -> ("Value"=w2320:bool)  [unwired: 2 in, 2 out]
            n1532 = Not(x=w2320) -> (.not. x?=w2319:bool)
            n1533 = And(x=w2319, y=w2317) -> (x .and. y?=w2318:bool)
            n1534 = case shown="True" w2318 {
              frame False {
              }
              frame True {
                n1535 = property on="A1-position-X" class="DigNum (strict)"() -> (error out=w2327:errorcluster, "Value"=w2334:dbl)  [unwired: 2 in, 1 out]
                n1536 = property on="A1-position-Y" class="DigNum (strict)"(error in=w2327) -> (error out=w2326:errorcluster, "Value"=w2323:dbl)  [unwired: 1 in, 1 out]
                n1537 = Subtract(x=w2323, y=27.0) -> (x-y=w2322:dbl)
                n1538 = Subtract(x=w2334, y=40.5) -> (x-y=w2325:dbl)
                n1539 = vi-ref "goto.vi"() -> (w2332:refnum<vi>)
                n1540 = property class="VI"(reference=w2332, error in=w2326) -> ("Name"=w2331:string)  [unwired: 2 out]
                n1541 = Open VI Reference(type specifier VI Refnum (for type only)=refnum<vi> refnum, vi path=w2331, options=128) -> (vi reference=w2329:refnum<vi>)  [unwired: 3 in, 1 out]
                n1542 = call-by-ref "Start Asynchronous Call"(reference=w2329, "Y(mm)"=w2322, "X(mm)"=w2325) -> ()  [unwired: 10 in, 3 out]
              }
            }
            n1543 = property on="currentNO" class="Str"("Value"="G10") -> ()  [unwired: 2 in, 2 out]
          }
          event "G11": Value Change {
            n1544 = event-data() -> ("NewVal"=w2336:bool)  [unwired: 1 in, 5 out]
            n1545 = property on="移动" class="Bool (strict)"() -> ("Value"=w2339:bool)  [unwired: 2 in, 2 out]
            n1546 = Not(x=w2339) -> (.not. x?=w2338:bool)
            n1547 = And(x=w2338, y=w2336) -> (x .and. y?=w2337:bool)
            n1548 = case shown="True" w2337 {
              frame False {
              }
              frame True {
                n1549 = property on="A1-position-X" class="DigNum (strict)"() -> (error out=w2346:errorcluster, "Value"=w2353:dbl)  [unwired: 2 in, 1 out]
                n1550 = property on="A1-position-Y" class="DigNum (strict)"(error in=w2346) -> (error out=w2345:errorcluster, "Value"=w2342:dbl)  [unwired: 1 in, 1 out]
                n1551 = Subtract(x=w2342, y=27.0) -> (x-y=w2341:dbl)
                n1552 = Subtract(x=w2353, y=45) -> (x-y=w2344:dbl)
                n1553 = vi-ref "goto.vi"() -> (w2351:refnum<vi>)
                n1554 = property class="VI"(reference=w2351, error in=w2345) -> ("Name"=w2350:string)  [unwired: 2 out]
                n1555 = Open VI Reference(type specifier VI Refnum (for type only)=refnum<vi> refnum, vi path=w2350, options=128) -> (vi reference=w2348:refnum<vi>)  [unwired: 3 in, 1 out]
                n1556 = call-by-ref "Start Asynchronous Call"(reference=w2348, "Y(mm)"=w2341, "X(mm)"=w2344) -> ()  [unwired: 10 in, 3 out]
              }
            }
            n1557 = property on="currentNO" class="Str"("Value"="G11") -> ()  [unwired: 2 in, 2 out]
          }
          event "G12": Value Change {
            n1558 = event-data() -> ("NewVal"=w2355:bool)  [unwired: 1 in, 5 out]
            n1559 = property on="移动" class="Bool (strict)"() -> ("Value"=w2358:bool)  [unwired: 2 in, 2 out]
            n1560 = Not(x=w2358) -> (.not. x?=w2357:bool)
            n1561 = And(x=w2357, y=w2355) -> (x .and. y?=w2356:bool)
            n1562 = case shown="True" w2356 {
              frame False {
              }
              frame True {
                n1563 = property on="A1-position-X" class="DigNum (strict)"() -> (error out=w2365:errorcluster, "Value"=w2372:dbl)  [unwired: 2 in, 1 out]
                n1564 = property on="A1-position-Y" class="DigNum (strict)"(error in=w2365) -> (error out=w2364:errorcluster, "Value"=w2361:dbl)  [unwired: 1 in, 1 out]
                n1565 = Subtract(x=w2361, y=27.0) -> (x-y=w2360:dbl)
                n1566 = Subtract(x=w2372, y=49.5) -> (x-y=w2363:dbl)
                n1567 = vi-ref "goto.vi"() -> (w2370:refnum<vi>)
                n1568 = property class="VI"(reference=w2370, error in=w2364) -> ("Name"=w2369:string)  [unwired: 2 out]
                n1569 = Open VI Reference(type specifier VI Refnum (for type only)=refnum<vi> refnum, vi path=w2369, options=128) -> (vi reference=w2367:refnum<vi>)  [unwired: 3 in, 1 out]
                n1570 = call-by-ref "Start Asynchronous Call"(reference=w2367, "Y(mm)"=w2360, "X(mm)"=w2363) -> ()  [unwired: 10 in, 3 out]
              }
            }
            n1571 = property on="currentNO" class="Str"("Value"="G12") -> ()  [unwired: 2 in, 2 out]
          }
          event "H1": Value Change {
            n1572 = event-data() -> ("NewVal"=w2374:bool)  [unwired: 1 in, 5 out]
            n1573 = property on="移动" class="Bool (strict)"() -> ("Value"=w2377:bool)  [unwired: 2 in, 2 out]
            n1574 = Not(x=w2377) -> (.not. x?=w2376:bool)
            n1575 = And(x=w2376, y=w2374) -> (x .and. y?=w2375:bool)
            n1576 = case shown="True" w2375 {
              frame False {
              }
              frame True {
                n1577 = property on="A1-position-X" class="DigNum (strict)"() -> (error out=w2384:errorcluster, "Value"=w2391:dbl)  [unwired: 2 in, 1 out]
                n1578 = property on="A1-position-Y" class="DigNum (strict)"(error in=w2384) -> (error out=w2383:errorcluster, "Value"=w2380:dbl)  [unwired: 1 in, 1 out]
                n1579 = Subtract(x=w2380, y=31.5) -> (x-y=w2379:dbl)
                n1580 = Subtract(x=w2391, y=0) -> (x-y=w2382:dbl)
                n1581 = vi-ref "goto.vi"() -> (w2389:refnum<vi>)
                n1582 = property class="VI"(reference=w2389, error in=w2383) -> ("Name"=w2388:string)  [unwired: 2 out]
                n1583 = Open VI Reference(type specifier VI Refnum (for type only)=refnum<vi> refnum, vi path=w2388, options=128) -> (vi reference=w2386:refnum<vi>)  [unwired: 3 in, 1 out]
                n1584 = call-by-ref "Start Asynchronous Call"(reference=w2386, "Y(mm)"=w2379, "X(mm)"=w2382) -> ()  [unwired: 10 in, 3 out]
              }
            }
            n1585 = property on="currentNO" class="Str"("Value"="H1") -> ()  [unwired: 2 in, 2 out]
          }
          event "H2": Value Change {
            n1586 = event-data() -> ("NewVal"=w2393:bool)  [unwired: 1 in, 5 out]
            n1587 = property on="移动" class="Bool (strict)"() -> ("Value"=w2396:bool)  [unwired: 2 in, 2 out]
            n1588 = Not(x=w2396) -> (.not. x?=w2395:bool)
            n1589 = And(x=w2395, y=w2393) -> (x .and. y?=w2394:bool)
            n1590 = case shown="True" w2394 {
              frame False {
              }
              frame True {
                n1591 = property on="A1-position-X" class="DigNum (strict)"() -> (error out=w2403:errorcluster, "Value"=w2410:dbl)  [unwired: 2 in, 1 out]
                n1592 = property on="A1-position-Y" class="DigNum (strict)"(error in=w2403) -> (error out=w2402:errorcluster, "Value"=w2399:dbl)  [unwired: 1 in, 1 out]
                n1593 = Subtract(x=w2399, y=31.5) -> (x-y=w2398:dbl)
                n1594 = Subtract(x=w2410, y=4.5) -> (x-y=w2401:dbl)
                n1595 = vi-ref "goto.vi"() -> (w2408:refnum<vi>)
                n1596 = property class="VI"(reference=w2408, error in=w2402) -> ("Name"=w2407:string)  [unwired: 2 out]
                n1597 = Open VI Reference(type specifier VI Refnum (for type only)=refnum<vi> refnum, vi path=w2407, options=128) -> (vi reference=w2405:refnum<vi>)  [unwired: 3 in, 1 out]
                n1598 = call-by-ref "Start Asynchronous Call"(reference=w2405, "Y(mm)"=w2398, "X(mm)"=w2401) -> ()  [unwired: 10 in, 3 out]
              }
            }
            n1599 = property on="currentNO" class="Str"("Value"="H2") -> ()  [unwired: 2 in, 2 out]
          }
          event "H3": Value Change {
            n1600 = event-data() -> ("NewVal"=w2412:bool)  [unwired: 1 in, 5 out]
            n1601 = property on="移动" class="Bool (strict)"() -> ("Value"=w2415:bool)  [unwired: 2 in, 2 out]
            n1602 = Not(x=w2415) -> (.not. x?=w2414:bool)
            n1603 = And(x=w2414, y=w2412) -> (x .and. y?=w2413:bool)
            n1604 = case shown="True" w2413 {
              frame False {
              }
              frame True {
                n1605 = property on="A1-position-X" class="DigNum (strict)"() -> (error out=w2422:errorcluster, "Value"=w2429:dbl)  [unwired: 2 in, 1 out]
                n1606 = property on="A1-position-Y" class="DigNum (strict)"(error in=w2422) -> (error out=w2421:errorcluster, "Value"=w2418:dbl)  [unwired: 1 in, 1 out]
                n1607 = Subtract(x=w2418, y=31.5) -> (x-y=w2417:dbl)
                n1608 = Subtract(x=w2429, y=9.0) -> (x-y=w2420:dbl)
                n1609 = vi-ref "goto.vi"() -> (w2427:refnum<vi>)
                n1610 = property class="VI"(reference=w2427, error in=w2421) -> ("Name"=w2426:string)  [unwired: 2 out]
                n1611 = Open VI Reference(type specifier VI Refnum (for type only)=refnum<vi> refnum, vi path=w2426, options=128) -> (vi reference=w2424:refnum<vi>)  [unwired: 3 in, 1 out]
                n1612 = call-by-ref "Start Asynchronous Call"(reference=w2424, "Y(mm)"=w2417, "X(mm)"=w2420) -> ()  [unwired: 10 in, 3 out]
              }
            }
            n1613 = property on="currentNO" class="Str"("Value"="H3") -> ()  [unwired: 2 in, 2 out]
          }
          event "H4": Value Change {
            n1614 = event-data() -> ("NewVal"=w2431:bool)  [unwired: 1 in, 5 out]
            n1615 = property on="移动" class="Bool (strict)"() -> ("Value"=w2434:bool)  [unwired: 2 in, 2 out]
            n1616 = Not(x=w2434) -> (.not. x?=w2433:bool)
            n1617 = And(x=w2433, y=w2431) -> (x .and. y?=w2432:bool)
            n1618 = case shown="True" w2432 {
              frame False {
              }
              frame True {
                n1619 = property on="A1-position-X" class="DigNum (strict)"() -> (error out=w2441:errorcluster, "Value"=w2448:dbl)  [unwired: 2 in, 1 out]
                n1620 = property on="A1-position-Y" class="DigNum (strict)"(error in=w2441) -> (error out=w2440:errorcluster, "Value"=w2437:dbl)  [unwired: 1 in, 1 out]
                n1621 = Subtract(x=w2437, y=31.5) -> (x-y=w2436:dbl)
                n1622 = Subtract(x=w2448, y=13.5) -> (x-y=w2439:dbl)
                n1623 = vi-ref "goto.vi"() -> (w2446:refnum<vi>)
                n1624 = property class="VI"(reference=w2446, error in=w2440) -> ("Name"=w2445:string)  [unwired: 2 out]
                n1625 = Open VI Reference(type specifier VI Refnum (for type only)=refnum<vi> refnum, vi path=w2445, options=128) -> (vi reference=w2443:refnum<vi>)  [unwired: 3 in, 1 out]
                n1626 = call-by-ref "Start Asynchronous Call"(reference=w2443, "Y(mm)"=w2436, "X(mm)"=w2439) -> ()  [unwired: 10 in, 3 out]
              }
            }
            n1627 = property on="currentNO" class="Str"("Value"="H4") -> ()  [unwired: 2 in, 2 out]
          }
          event "H5": Value Change {
            n1628 = event-data() -> ("NewVal"=w2450:bool)  [unwired: 1 in, 5 out]
            n1629 = property on="移动" class="Bool (strict)"() -> ("Value"=w2453:bool)  [unwired: 2 in, 2 out]
            n1630 = Not(x=w2453) -> (.not. x?=w2452:bool)
            n1631 = And(x=w2452, y=w2450) -> (x .and. y?=w2451:bool)
            n1632 = case shown="True" w2451 {
              frame False {
              }
              frame True {
                n1633 = property on="A1-position-X" class="DigNum (strict)"() -> (error out=w2460:errorcluster, "Value"=w2467:dbl)  [unwired: 2 in, 1 out]
                n1634 = property on="A1-position-Y" class="DigNum (strict)"(error in=w2460) -> (error out=w2459:errorcluster, "Value"=w2456:dbl)  [unwired: 1 in, 1 out]
                n1635 = Subtract(x=w2456, y=31.5) -> (x-y=w2455:dbl)
                n1636 = Subtract(x=w2467, y=18) -> (x-y=w2458:dbl)
                n1637 = vi-ref "goto.vi"() -> (w2465:refnum<vi>)
                n1638 = property class="VI"(reference=w2465, error in=w2459) -> ("Name"=w2464:string)  [unwired: 2 out]
                n1639 = Open VI Reference(type specifier VI Refnum (for type only)=refnum<vi> refnum, vi path=w2464, options=128) -> (vi reference=w2462:refnum<vi>)  [unwired: 3 in, 1 out]
                n1640 = call-by-ref "Start Asynchronous Call"(reference=w2462, "Y(mm)"=w2455, "X(mm)"=w2458) -> ()  [unwired: 10 in, 3 out]
              }
            }
            n1641 = property on="currentNO" class="Str"("Value"="H5") -> ()  [unwired: 2 in, 2 out]
          }
          event "H6": Value Change {
            n1642 = event-data() -> ("NewVal"=w2469:bool)  [unwired: 1 in, 5 out]
            n1643 = property on="移动" class="Bool (strict)"() -> ("Value"=w2472:bool)  [unwired: 2 in, 2 out]
            n1644 = Not(x=w2472) -> (.not. x?=w2471:bool)
            n1645 = And(x=w2471, y=w2469) -> (x .and. y?=w2470:bool)
            n1646 = case shown="True" w2470 {
              frame False {
              }
              frame True {
                n1647 = property on="A1-position-X" class="DigNum (strict)"() -> (error out=w2479:errorcluster, "Value"=w2486:dbl)  [unwired: 2 in, 1 out]
                n1648 = property on="A1-position-Y" class="DigNum (strict)"(error in=w2479) -> (error out=w2478:errorcluster, "Value"=w2475:dbl)  [unwired: 1 in, 1 out]
                n1649 = Subtract(x=w2475, y=31.5) -> (x-y=w2474:dbl)
                n1650 = Subtract(x=w2486, y=22.5) -> (x-y=w2477:dbl)
                n1651 = vi-ref "goto.vi"() -> (w2484:refnum<vi>)
                n1652 = property class="VI"(reference=w2484, error in=w2478) -> ("Name"=w2483:string)  [unwired: 2 out]
                n1653 = Open VI Reference(type specifier VI Refnum (for type only)=refnum<vi> refnum, vi path=w2483, options=128) -> (vi reference=w2481:refnum<vi>)  [unwired: 3 in, 1 out]
                n1654 = call-by-ref "Start Asynchronous Call"(reference=w2481, "Y(mm)"=w2474, "X(mm)"=w2477) -> ()  [unwired: 10 in, 3 out]
              }
            }
            n1655 = property on="currentNO" class="Str"("Value"="H6") -> ()  [unwired: 2 in, 2 out]
          }
          event "H7": Value Change {
            n1656 = event-data() -> ("NewVal"=w2488:bool)  [unwired: 1 in, 5 out]
            n1657 = property on="移动" class="Bool (strict)"() -> ("Value"=w2491:bool)  [unwired: 2 in, 2 out]
            n1658 = Not(x=w2491) -> (.not. x?=w2490:bool)
            n1659 = And(x=w2490, y=w2488) -> (x .and. y?=w2489:bool)
            n1660 = case shown="True" w2489 {
              frame False {
              }
              frame True {
                n1661 = property on="A1-position-X" class="DigNum (strict)"() -> (error out=w2498:errorcluster, "Value"=w2505:dbl)  [unwired: 2 in, 1 out]
                n1662 = property on="A1-position-Y" class="DigNum (strict)"(error in=w2498) -> (error out=w2497:errorcluster, "Value"=w2494:dbl)  [unwired: 1 in, 1 out]
                n1663 = Subtract(x=w2494, y=31.5) -> (x-y=w2493:dbl)
                n1664 = Subtract(x=w2505, y=27) -> (x-y=w2496:dbl)
                n1665 = vi-ref "goto.vi"() -> (w2503:refnum<vi>)
                n1666 = property class="VI"(reference=w2503, error in=w2497) -> ("Name"=w2502:string)  [unwired: 2 out]
                n1667 = Open VI Reference(type specifier VI Refnum (for type only)=refnum<vi> refnum, vi path=w2502, options=128) -> (vi reference=w2500:refnum<vi>)  [unwired: 3 in, 1 out]
                n1668 = call-by-ref "Start Asynchronous Call"(reference=w2500, "Y(mm)"=w2493, "X(mm)"=w2496) -> ()  [unwired: 10 in, 3 out]
              }
            }
            n1669 = property on="currentNO" class="Str"("Value"="H7") -> ()  [unwired: 2 in, 2 out]
          }
          event "H8": Value Change {
            n1670 = event-data() -> ("NewVal"=w2507:bool)  [unwired: 1 in, 5 out]
            n1671 = property on="移动" class="Bool (strict)"() -> ("Value"=w2510:bool)  [unwired: 2 in, 2 out]
            n1672 = Not(x=w2510) -> (.not. x?=w2509:bool)
            n1673 = And(x=w2509, y=w2507) -> (x .and. y?=w2508:bool)
            n1674 = case shown="True" w2508 {
              frame False {
              }
              frame True {
                n1675 = property on="A1-position-X" class="DigNum (strict)"() -> (error out=w2517:errorcluster, "Value"=w2524:dbl)  [unwired: 2 in, 1 out]
                n1676 = property on="A1-position-Y" class="DigNum (strict)"(error in=w2517) -> (error out=w2516:errorcluster, "Value"=w2513:dbl)  [unwired: 1 in, 1 out]
                n1677 = Subtract(x=w2513, y=31.5) -> (x-y=w2512:dbl)
                n1678 = Subtract(x=w2524, y=31.5) -> (x-y=w2515:dbl)
                n1679 = vi-ref "goto.vi"() -> (w2522:refnum<vi>)
                n1680 = property class="VI"(reference=w2522, error in=w2516) -> ("Name"=w2521:string)  [unwired: 2 out]
                n1681 = Open VI Reference(type specifier VI Refnum (for type only)=refnum<vi> refnum, vi path=w2521, options=128) -> (vi reference=w2519:refnum<vi>)  [unwired: 3 in, 1 out]
                n1682 = call-by-ref "Start Asynchronous Call"(reference=w2519, "Y(mm)"=w2512, "X(mm)"=w2515) -> ()  [unwired: 10 in, 3 out]
              }
            }
            n1683 = property on="currentNO" class="Str"("Value"="H8") -> ()  [unwired: 2 in, 2 out]
          }
          event "H9": Value Change {
            n1684 = event-data() -> ("NewVal"=w2526:bool)  [unwired: 1 in, 5 out]
            n1685 = property on="移动" class="Bool (strict)"() -> ("Value"=w2529:bool)  [unwired: 2 in, 2 out]
            n1686 = Not(x=w2529) -> (.not. x?=w2528:bool)
            n1687 = And(x=w2528, y=w2526) -> (x .and. y?=w2527:bool)
            n1688 = case shown="True" w2527 {
              frame False {
              }
              frame True {
                n1689 = property on="A1-position-X" class="DigNum (strict)"() -> (error out=w2536:errorcluster, "Value"=w2543:dbl)  [unwired: 2 in, 1 out]
                n1690 = property on="A1-position-Y" class="DigNum (strict)"(error in=w2536) -> (error out=w2535:errorcluster, "Value"=w2532:dbl)  [unwired: 1 in, 1 out]
                n1691 = Subtract(x=w2532, y=31.5) -> (x-y=w2531:dbl)
                n1692 = Subtract(x=w2543, y=36) -> (x-y=w2534:dbl)
                n1693 = vi-ref "goto.vi"() -> (w2541:refnum<vi>)
                n1694 = property class="VI"(reference=w2541, error in=w2535) -> ("Name"=w2540:string)  [unwired: 2 out]
                n1695 = Open VI Reference(type specifier VI Refnum (for type only)=refnum<vi> refnum, vi path=w2540, options=128) -> (vi reference=w2538:refnum<vi>)  [unwired: 3 in, 1 out]
                n1696 = call-by-ref "Start Asynchronous Call"(reference=w2538, "Y(mm)"=w2531, "X(mm)"=w2534) -> ()  [unwired: 10 in, 3 out]
              }
            }
            n1697 = property on="currentNO" class="Str"("Value"="H9") -> ()  [unwired: 2 in, 2 out]
          }
          event "H10": Value Change {
            n1698 = event-data() -> ("NewVal"=w2545:bool)  [unwired: 1 in, 5 out]
            n1699 = property on="移动" class="Bool (strict)"() -> ("Value"=w2548:bool)  [unwired: 2 in, 2 out]
            n1700 = Not(x=w2548) -> (.not. x?=w2547:bool)
            n1701 = And(x=w2547, y=w2545) -> (x .and. y?=w2546:bool)
            n1702 = case shown="True" w2546 {
              frame False {
              }
              frame True {
                n1703 = property on="A1-position-X" class="DigNum (strict)"() -> (error out=w2555:errorcluster, "Value"=w2562:dbl)  [unwired: 2 in, 1 out]
                n1704 = property on="A1-position-Y" class="DigNum (strict)"(error in=w2555) -> (error out=w2554:errorcluster, "Value"=w2551:dbl)  [unwired: 1 in, 1 out]
                n1705 = Subtract(x=w2551, y=31.5) -> (x-y=w2550:dbl)
                n1706 = Subtract(x=w2562, y=40.5) -> (x-y=w2553:dbl)
                n1707 = vi-ref "goto.vi"() -> (w2560:refnum<vi>)
                n1708 = property class="VI"(reference=w2560, error in=w2554) -> ("Name"=w2559:string)  [unwired: 2 out]
                n1709 = Open VI Reference(type specifier VI Refnum (for type only)=refnum<vi> refnum, vi path=w2559, options=128) -> (vi reference=w2557:refnum<vi>)  [unwired: 3 in, 1 out]
                n1710 = call-by-ref "Start Asynchronous Call"(reference=w2557, "Y(mm)"=w2550, "X(mm)"=w2553) -> ()  [unwired: 10 in, 3 out]
              }
            }
            n1711 = property on="currentNO" class="Str"("Value"="H10") -> ()  [unwired: 2 in, 2 out]
          }
          event "H11": Value Change {
            n1712 = event-data() -> ("NewVal"=w2564:bool)  [unwired: 1 in, 5 out]
            n1713 = property on="移动" class="Bool (strict)"() -> ("Value"=w2567:bool)  [unwired: 2 in, 2 out]
            n1714 = Not(x=w2567) -> (.not. x?=w2566:bool)
            n1715 = And(x=w2566, y=w2564) -> (x .and. y?=w2565:bool)
            n1716 = case shown="True" w2565 {
              frame False {
              }
              frame True {
                n1717 = property on="A1-position-X" class="DigNum (strict)"() -> (error out=w2574:errorcluster, "Value"=w2581:dbl)  [unwired: 2 in, 1 out]
                n1718 = property on="A1-position-Y" class="DigNum (strict)"(error in=w2574) -> (error out=w2573:errorcluster, "Value"=w2570:dbl)  [unwired: 1 in, 1 out]
                n1719 = Subtract(x=w2570, y=31.5) -> (x-y=w2569:dbl)
                n1720 = Subtract(x=w2581, y=45) -> (x-y=w2572:dbl)
                n1721 = vi-ref "goto.vi"() -> (w2579:refnum<vi>)
                n1722 = property class="VI"(reference=w2579, error in=w2573) -> ("Name"=w2578:string)  [unwired: 2 out]
                n1723 = Open VI Reference(type specifier VI Refnum (for type only)=refnum<vi> refnum, vi path=w2578, options=128) -> (vi reference=w2576:refnum<vi>)  [unwired: 3 in, 1 out]
                n1724 = call-by-ref "Start Asynchronous Call"(reference=w2576, "Y(mm)"=w2569, "X(mm)"=w2572) -> ()  [unwired: 10 in, 3 out]
              }
            }
            n1725 = property on="currentNO" class="Str"("Value"="H11") -> ()  [unwired: 2 in, 2 out]
          }
          event "H12": Value Change {
            n1726 = event-data() -> ("NewVal"=w2583:bool)  [unwired: 1 in, 5 out]
            n1727 = property on="移动" class="Bool (strict)"() -> ("Value"=w2586:bool)  [unwired: 2 in, 2 out]
            n1728 = Not(x=w2586) -> (.not. x?=w2585:bool)
            n1729 = And(x=w2585, y=w2583) -> (x .and. y?=w2584:bool)
            n1730 = case shown="True" w2584 {
              frame False {
              }
              frame True {
                n1731 = property on="A1-position-X" class="DigNum (strict)"() -> (error out=w2593:errorcluster, "Value"=w2600:dbl)  [unwired: 2 in, 1 out]
                n1732 = property on="A1-position-Y" class="DigNum (strict)"(error in=w2593) -> (error out=w2592:errorcluster, "Value"=w2589:dbl)  [unwired: 1 in, 1 out]
                n1733 = Subtract(x=w2589, y=31.5) -> (x-y=w2588:dbl)
                n1734 = Subtract(x=w2600, y=49.5) -> (x-y=w2591:dbl)
                n1735 = vi-ref "goto.vi"() -> (w2598:refnum<vi>)
                n1736 = property class="VI"(reference=w2598, error in=w2592) -> ("Name"=w2597:string)  [unwired: 2 out]
                n1737 = Open VI Reference(type specifier VI Refnum (for type only)=refnum<vi> refnum, vi path=w2597, options=128) -> (vi reference=w2595:refnum<vi>)  [unwired: 3 in, 1 out]
                n1738 = call-by-ref "Start Asynchronous Call"(reference=w2595, "Y(mm)"=w2588, "X(mm)"=w2591) -> ()  [unwired: 10 in, 3 out]
              }
            }
            n1739 = property on="currentNO" class="Str"("Value"="H12") -> ()  [unwired: 2 in, 2 out]
          }
          event "ShutDownSystem": Value Change {
            n1740 = event-data() -> ("NewVal"=w2603:bool)  [unwired: 1 in, 5 out]
            n1741 = case shown="True" w2603 {
              tunnel: w2602 -> [_ w2607]
              frame False {
              }
              frame True {
                n1742 = Unbundle By Name(w2607) -> ("ConfiguredPumpCom"=w2606:refnum<visa-resource-name>, "ConfiguredLaserCom"=w2605:refnum<visa-resource-name>)
                n1743 = VISA Close(VISA resource name=w2606) -> (error out=w2604:errorcluster)  [unwired: 1 in]
                n1744 = VISA Close(VISA resource name=w2605, error in (no error)=w2604) -> ()  [unwired: 1 out]
              }
            }
          }
        }
      }
      n1745 = while {
        tunnel: w91 -> [w97]
        stop <- FALSE stop-if-true
        n1746 = event shown="[2] <motor status>: User Event" {
          selector: w97 -> [_ _ _ _]
          dyn-events: _ -> [_ _ _ _]
          timeout: _ -> [_ _ _ _]
          event Timeout {
            n1747 = event-data() -> ()  [unwired: 1 in, 3 out]
          }
          event User Event {
            n1748 = event-data() -> ("AI"=w99:dbl[], "DI"=w98:bool[])  [unwired: 1 in, 4 out]
            n1749 = Index Array(array=w99, index=0) -> (element=w117:dbl)
            n1750 = Index Array(array=w98, index=0) -> (element=→"X0":bool)
            n1751 = Divide(x=w117, y=10.0) -> (x/y=w119:dbl)
            n1752 = Multiply(x=w119, y=2000.0) -> (x*y=w121:dbl)
            n1753 = property on="MCPHV-Real" class="DigNum (strict)"("Value"=w121) -> (error out=w100:errorcluster)  [unwired: 2 in, 1 out]
            n1754 = Index Array(array=w98, index=4) -> (element=→"Y0":bool)
            n1755 = Index Array(array=w99, index=1) -> (element=w122:dbl)
            n1756 = Divide(x=w122, y=10.0) -> (x/y=w124:dbl)
            n1757 = Multiply(x=w124, y=20000.0) -> (x*y=w126:dbl)
            n1758 = Index Array(array=w98, index=1) -> (element=→"X满":bool)
            n1759 = property on="Tar.HV-Real" class="DigNum (strict)"(error in=w100, "Value"=w126) -> (error out=w101:errorcluster)  [unwired: 1 in, 1 out]
            n1760 = Index Array(array=w99, index=2) -> (element=w127:dbl)
            n1761 = Index Array(array=w98, index=3) -> (element=→"Y标":bool)
            n1762 = Divide(x=w127, y=10.0) -> (x/y=w129:dbl)
            n1763 = Multiply(x=w129, y=2000.0) -> (x*y=w131:dbl)
            n1764 = property on="Pul.HV-Real" class="DigNum (strict)"(error in=w101, "Value"=w131) -> (error out=w102:errorcluster)  [unwired: 1 in, 1 out]
            n1765 = Index Array(array=w99, index=3) -> (element=w132:dbl)
            n1766 = Index Array(array=w98, index=2) -> (element=→"Y满":bool)
            n1767 = Divide(x=w132, y=10.0) -> (x/y=w134:dbl)
            n1768 = Multiply(x=w134, y=10000.0) -> (x*y=w136:dbl)
            n1769 = property on="LensHV-Real" class="DigNum (strict)"(error in=w102, "Value"=w136) -> (error out=w138:errorcluster)  [unwired: 1 in, 1 out]
            n1770 = Index Array(array=w99, index=19) -> (element=w140:dbl)
            n1771 = Subtract(x=w140, y=3.572) -> (x-y=w142:dbl)
            n1772 = Divide(x=w142, y=1.286) -> (x/y=w144:dbl)
            n1773 = Power Of 10(x=w144) -> (10^x=w145:dbl)
            n1774 = Index Array(array=w99, index=18) -> (element=w146:dbl)
            n1775 = Subtract(x=w146, y=8.5) -> (x-y=w148:dbl)
            n1776 = property on="Lvaccum" class="DigNum (strict)"(error in=w138, "Value"=w145) -> (error out=w150:errorcluster)  [unwired: 1 in, 1 out]
            n1777 = Power Of 10(x=w148) -> (10^x=w149:dbl)
            n1778 = property on="Hvaccum" class="DigNum (strict)"(error in=w150, "Value"=w149) -> ()  [unwired: 1 in, 2 out]
          }
          event User Event {
            n1779 = event-data() -> ("status"=w151:string)  [unwired: 1 in, 5 out]
            n1780 = case shown="\"moving\"" w151 {
              frame "stop", Default {
                n1781 = property on="GO" class="Bool (strict)"("DisabledEnum"=T10."Enabled" ("Disabled")) -> (error out=w153:errorcluster)  [unwired: 2 in, 1 out]
                n1782 = property on="移动" class="Bool (strict)"(error in=w153, "Value"=FALSE ("移动")) -> ()  [unwired: 1 in, 2 out]
              }
              frame "moving" {
                n1783 = property on="GO" class="Bool (strict)"("DisabledEnum"=T10."Disabled and Grayed Out" ("Disabled")) -> (error out=w156:errorcluster)  [unwired: 2 in, 1 out]
                n1784 = property on="移动" class="Bool (strict)"(error in=w156, "Value"=TRUE ("移动")) -> ()  [unwired: 1 in, 2 out]
              }
            }
          }
          event User Event {
            n1785 = event-data() -> ("source"=w158:string, "value"=w159:dbl)  [unwired: 1 in, 4 out]
            n1786 = case shown="\"X\"" w158 {
              tunnel: w159 -> [w166 w174]
              tunnel: [w168 w175] -> w165
              frame "Y", Default {
                n1787 = property on="X当前" class="DigNum (strict)"() -> ("Value"=w170:dbl)  [unwired: 2 in, 2 out]
                n1788 = Multiply(x=w166, y=1000.0) -> (x*y=w171:dbl)
                n1789 = Divide(x=w170, y=1000.0) -> (x/y=w167:dbl)
                n1790 = Build Array "Build Array"(w167, w166) -> (w168:dbl[])
                n1791 = property on="Y当前" class="DigNum (strict)"("Value"=w171) -> ()  [unwired: 2 in, 2 out]
              }
              frame "X" {
                n1792 = property on="Y当前" class="DigNum (strict)"() -> ("Value"=w177:dbl)  [unwired: 2 in, 2 out]
                n1793 = Multiply(x=w174, y=1000.0) -> (x*y=w178:dbl)
                n1794 = Divide(x=w177, y=1000.0) -> (x/y=w173:dbl)
                n1795 = property on="X当前" class="DigNum (strict)"("Value"=w178) -> ()  [unwired: 2 in, 2 out]
                n1796 = Build Array(w174, w173) -> (w175:dbl[])
              }
            }
            n1797 = Current VI's Path() -> (path=w162:path)
            n1798 = Strip Path(path=w162) -> (stripped path=w163:path)  [unwired: 1 out]
            n1799 = Build Path(base path=w163, name or relative path="last_position") -> (appended path=w161:path)
            n1800 = call-poly <vilib>:"Write To Spreadsheet File.vi"("format (%.3f)"="%.9f", "1D data"=w165, "file path (dialog if empty)"=w161) -> ()  [unwired: 5 in, 1 out]
          }
        }
      }
    }
  }
  n1801 = Unbundle(w23) -> ("tasks"=w4:T13, "interface"=w3:T12, "error out"=w2:errorcluster)
  n1802 = call "USB6343_Control_v1.6.2.vi"("error in"=w2, "interface"=w3, "tasks"=w4) -> ()  [unwired: 9 in]
  n1803 = call <vilib>:"IMAQdx Enumerate Cameras.vi"() -> ("error out"=w13:errorcluster, "Camera Information Array"=w10:T18)  [unwired: 10 in]
  n1804 = while {
    tunnel: w25 -> [w2634]
    tunnel: w24 -> [w2632]
    stop <- FALSE stop-if-true
    n1805 = Unbundle By Name(w2634) -> ("pump semaphore"=w2633:T3, "laser semaphore"=w2629:T3)
    n1806 = Unbundle By Name(w2632) -> ("ConfiguredPumpCom"=w2631:refnum<visa-resource-name>, "ConfiguredLaserCom"=w2619:refnum<visa-resource-name>)
    n1807 = call <vilib>:"Acquire Semaphore.vi"("semaphore"=w2633) -> ("error out"=w2618:errorcluster, "semaphore out"=w2630:T3)  [unwired: 4 in, 1 out]
    n1808 = call "pumpStatus.vi"("VISA resource name"=w2631, "error in (no error)"=w2618) -> ("PumpKW"=→"PumpKW":dbl, "PumpTemp"=→"PumpTemp":u16, "PumpAmps"=→"PumpAmps":dbl, "PumpVolts"=→"PumpVolts":dbl, "TurboSpeed"=→"TurboSpeed":dbl, "error out"=w2617:errorcluster)  [unwired: 8 in]
    n1809 = call <vilib>:"Release Semaphore.vi"("error in (no error)"=w2617, "semaphore"=w2630) -> ("error out"=w2615:errorcluster)  [unwired: 4 in, 1 out]
    n1810 = call <vilib>:"Acquire Semaphore.vi"("error in (no error)"=w2615, "semaphore"=w2629) -> ("error out"=w2616:errorcluster, "semaphore out"=w2614:T3)  [unwired: 3 in, 1 out]
    n1811 = call "Laser-Get-Shotstatus.vi"("VISA resource name"=w2619, "error in (no error)"=w2616) -> ("VISA resource name out"=w2612:refnum<visa-resource-name>, "cluster"=→"cluster":T7, "error out"=w2610:errorcluster)
    n1812 = property on="SetLaserTransmission" class="Slide (strict)"(error in=w2610) -> (error out=w2609:errorcluster, "Value"=w2608:dbl)  [unwired: 1 in, 1 out]
    n1813 = call "Laser-Read-Energy.vi"("Transimission"=w2608, "error in (no error)"=w2609, "VISA resource name"=w2612) -> ("LaserEnergy uJ"=→"LaserEnergy uJ 2":dbl, "error out"=w2613:errorcluster)  [unwired: 1 out]
    n1814 = call <vilib>:"Release Semaphore.vi"("error in (no error)"=w2613, "semaphore"=w2614) -> ("error out"=w2628:errorcluster)  [unwired: 4 in, 1 out]
    n1815 = call "Time Delay2"("error in (no error)"=w2628, "Delay Time (s)"=0.3) -> ()  [unwired: 9 in, 1 out]
  }
  n1816 = Index Array(array=w10, index=0) -> (element=w12:T19)
  n1817 = Unbundle By Name(w12) -> ("InterfaceName"=w20:string)
  n1818 = call <vilib>:"IMAQdx Open Camera.vi"("error in"=w13, "Session In"=w20) -> ("error out"=w7:errorcluster, "Session Out"=w8:T20)  [unwired: 8 in]
  n1819 = property class="IMAQdx" props=["VideoMode", "Width", "Height"](reference=w8, error in=w7, "VideoMode"=u32 13) -> (reference out=w6:T20, error out=w5:errorcluster)  [unwired: 2 out]
  n1820 = call "IMAQ Create"("Image Name"=w20) -> ("New Image"=w15:T2)  [unwired: 4 in, 1 out]
  n1821 = call <vilib>:"IMAQdx Configure Grab.vi"("error in"=w5, "Session In"=w6) -> ("error out"=w19:errorcluster, "Session Out"=w14:T20)  [unwired: 8 in]
  n1822 = while {
    tunnel: w19 -> [w2641]
    tunnel: w14 -> [w2640]
    tunnel: w15 -> [w2639]
    tunnel: [w2638] -> w16
    tunnel: [w2637] -> w17
    tunnel: [w2636] -> w18
    stop <- FALSE stop-if-true
    n1823 = call <vilib>:"IMAQdx Grab.vi"("error in"=w2641, "Image In"=w2639, "Session In"=w2640) -> ("error out"=w2638:errorcluster, "Image Out"=w2636:T2, "Session Out"=w2637:T20)  [unwired: 5 in, 1 out]
    "Image" <- w2636
  }
  n1824 = call "IMAQ Dispose"("Image"=w18) -> ()  [unwired: 5 in, 1 out]
  n1825 = call <vilib>:"IMAQdx Close Camera.vi"("error in"=w16, "Session In"=w17) -> ()  [unwired: 9 in, 1 out]
